vi "BIMS_Collector (2010_03).vi"() -> ()   [LabVIEW 2015]
doc: "This program is currently beta software. It is designed to address the data requirements defined primarily by the DHB Ballistic Test Report.\n\nThe general operation of this program is based on the Ballistics Version 2005 application developed internally by DuPont as a research tool for the Spruance Plant Ballistics Lab in Richmond, VA.\n\nPlease note that the original trigger control logic was modified and no longer depends on a safety interlock system to enable operation of a ballistic test.\n\nDuPont makes no warranties and assumes no liabilities in connection with any use of this program."
uses:
  <vilib>/addons/database/NI_Database_API.lvlib
  <vilib>/addons/database/Connection.llb/Conn Execute.vi
  <vilib>/addons/database/Recordset.llb/Rec Destroy - Connection.vi
  <vilib>/Utility/config.llb/NI_LVConfig.lvlib
  <vilib>/Utility/config.llb/Write Key (I32).vi
  Shot Record.ctl
  BIMS_Collector Globals.vi
  Collector State.ctl
  DataSource.ctl
  <vilib>/registry/registry.llb/Registry RtKey.ctl
  <vilib>/Utility/config.llb/Write Key (String).vi
  <vilib>/addons/database/Connection.llb/DB Tools Open Connec (Path).vi
panel:
  out "Loading":u16(ring)
  in  "runtimeMenusVisible":bool=TRUE
  in  "diagPageVisible":bool
  in  "RESET All":bool
  out "ConfigName":string
  out "TimeNow":string
  in  "EXIT":bool
  in  "mainTabCntrl":enum32{"Setup", "Measure", "History", "System"}(tab)=enum."System"
  in  "SampleEntryTabCntrl":enum32{"Environment", "Sample"}(tab)
  in  "ThreatDetails":u16(ring) caption="Detail"
  in  "ThreatGroups":u16(ring) caption="Group" items=["", "RCC", "FSP", "44 Magnum", "40 S&W", "9mm Luger", "357 Magnum", "357 Sig", "5.56 NATO / 223", "7.62 Win"]
  in  "PowderTypes":u16(ring) caption="Type" items=["", "ACCURATE, NO.2", "ACCURATE, NO.9", "Alliant Herc. Bullseye", "Alliant 2400", "Hercules", "Hi-Skor 700x", "Hi-Skor 800x", "IMR-4198", "IMR-4756", "IMR-4895", "Power Pistol", "Winchester Ball", "WINCHESTER-231", "WINCHESTER-296", "OTHER"]
  in  "Ballisticians":u16(ring) caption="Ballistician" items=["", "Luke Jeter", "Pat Fitzgerald", "James Singletary", "Aldo Tavarez"]
  in  "Recorders":u16(ring) caption="Recorder"
  in  "Shooters":u16(ring) caption="Shooter"
  in  "Methods":u16(ring) caption="Method" items=["", "V50", "NIJ", "V0", "Custom"]
  in  "RoomT":sgl caption="Temperature (° F)" format="%.1f"
  in  "RoomHum":sgl caption="Humidity (%)" min=0 max=100 format="%.1f"
  in  "SampleBackings":u16(ring)=3 caption="Type" items=["", "Clay", "Aluminum", "Air"]
  in  "clayCalArray":i16[](array[numeric])=[0, 0, 0, 0, 0] caption="Calibration (mm)" min=0 max=99 format="%02.0f"
  out "clayAverage":sgl caption="Clay Average (mm)" format="%#.1f"
  in  "clayTemp":sgl caption="Clay Temp (° F)" format="%.1f"
  out "threatDetails":T1 caption="Description"
  in  "SampleClamping":u16(ring) caption="Clamping" items=["", "None", "12 x 12", "12 x 15", "15 x 15 Flat", "15 x 15 Teeth", "16 x 16 Flat", "16 x 16 Teeth", "18 x 18", "20 x 20", "Hydro Pneumatic"]
  in  "Sample SubTabCntrl":T2(tab)
  in  "SampleID":string caption="Sample ID"
  in  "SampleDimensions":u16(ring) caption="Dimensions" items=["", "15 x 15", "12 x 12", "10.25 x 11.75", "15 x 16", "26 x 26", "8.5 x 11", "12 x 15", "16 x 16", "18 x 18", "20 x 16", "15 x 18", "24 x 24", "13 x 13", "7.5 x 7.5", "VEST PANEL", "CHEST PLATE", "HELMET", "NOT APPLICABLE"]
  in  "ModelMfrs":u16(ring) caption="Manufacturer" items=["DuPont Experimental", "Clark Schwebel", "Industriales Textiles", "Maydown", "Second Chance Body Armor", "Point Blank-Marine Interceptor", "Safari Land", "American Body Armor", "Europe", "Force One", "Textile Filter", "Hexcel Schwebel", "BGF", "M.C. GILL", "COLUMBIA", "Britax HEATH TECN", "ARLON", "TEX TECH INC.", "TELAIR", "CADDIN BODY ARMOR", "GEPCO", "3 TEX", "PACA BODY ARMOR", "VON ROL ISOLA", "SIOUX MANUFACTURING", "APEJ-TAIWAN", "FLOPPY BODY ARMOR", "UNICOR", "n/a", "Point Blank", "Diamond Back", "Other"]
  in  "SampleTypes":u16(ring) caption="Sample Type" items=["", "Fabric", "Hard", "Helmet", "Vest", "Paper"]
  in  "Submitters":u16(ring) caption="Submitter" items=["", "Aldo Tavarez", "James Singletary", "Jeff Hanks", "Karl Chang", "Minshon Chiou", "Other", "Navin Tejani", "Pat Fitzgerald", "Ron Egres", "Bryce VanArsdalen", "Kevin Mulcahy"]
  in  "ProjectID":string caption="Project ID"
  in  "BackLayers":i32 caption="# of Layers" min=0 max=99 step=5
  in  "FrontLayers":i32 caption="# of Layers" min=0 max=99 step=5
  in  "BackLayer":u16(ring) caption="Back Layer" items=["", "n/a", "CORDURA 500d"]
  in  "FrontLayer":u16(ring) caption="Front Layer" items=["", "n/a", "CORDURA 1000d"]
  out "totalNumLayers":i32 caption="Total # of Layers" min=0 max=100 step=5
  out "totalBAW":sgl caption="Total BAW (psf)" format="%.2f"
  in  "LayerTabControl":enum32{"1", "2", "3", "4", "5", "6"}(tab) caption="Inner Layers"
  out "fab1_totalWt":sgl caption="Fab1 Wt" min=0 max=99 step=5 format="%.2f"
  out "SampleAttribs_1":T3 caption="fabricAttribs_1"
  in  "Layer_1":T4={"plyNum"=0, "LotNum"="n/a", "RollNum"="n/a"} caption="Fabric #1" {"plyNum" min=0 max=99 step=5}
  in  "SampleStyle_1":u16(ring) items=["", "15492"]
  in  "Mfr_1":u16(ring) caption="vendor" items=["", "Barrday", "DSM", "DuPont AFS", "Dyneema", "Honeywell", "JPS", "TexTech"]
  in  "layerStitch_1":u16(ring) caption="Stitch" items=["", "1-inch quilt", "2-inch quilt", "Corner Bartack", "Corners", "Custom (Panel)", "Custom (Vest)", "Diamond", "Edge", "n/a", "Normal"]
  out "fab2_totalWt":sgl caption="Fab2 Wt" min=0 max=99 step=5 format="%.2f"
  out "SampleAttribs_2":T3 caption="fabricAttribs_2"
  in  "Layer_2":T4={"plyNum"=0, "LotNum"="n/a", "RollNum"="n/a"} caption="Fabric #2" {"plyNum" min=0 max=99 step=5}
  in  "SampleStyle_2":u16(ring)
  in  "Mfr_2":u16(ring) caption="vendor" items=["", "Barrday", "DSM", "DuPont AFS", "Dyneema", "Honeywell", "JPS", "TexTech"]
  in  "layerStitch_2":u16(ring) caption="Stitch" items=["", "1-inch quilt", "2-inch quilt", "Corner Bartack", "Corners", "Custom (Panel)", "Custom (Vest)", "Diamond", "Edge", "n/a", "Normal"]
  out "fab3_totalWt":sgl caption="Fab3 Wt" min=0 max=99 step=5 format="%.2f"
  out "SampleAttribs_3":T3 caption="fabricAttribs_3"
  in  "Layer_3":T4={"plyNum"=0, "LotNum"="n/a", "RollNum"="n/a"} caption="Fabric #3" {"plyNum" min=0 max=99 step=5}
  in  "SampleStyle_3":u16(ring)
  in  "Mfr_3":u16(ring) caption="vendor" items=["", "Barrday", "DSM", "DuPont AFS", "Dyneema", "Honeywell", "JPS", "TexTech"]
  in  "layerStitch_3":u16(ring) caption="Stitch" items=["", "1-inch quilt", "2-inch quilt", "Corner Bartack", "Corners", "Custom (Panel)", "Custom (Vest)", "Diamond", "Edge", "n/a", "Normal"]
  out "fab4_totalWt":sgl caption="Fab4 Wt" min=0 max=99 step=5 format="%.2f"
  out "SampleAttribs_4":T3 caption="fabricAttribs_4"
  in  "Layer_4":T4={"plyNum"=0, "LotNum"="n/a", "RollNum"="n/a"} caption="Fabric #4" {"plyNum" min=0 max=99 step=5}
  in  "SampleStyle_4":u16(ring)
  in  "Mfr_4":u16(ring) caption="vendor" items=["", "Barrday", "DSM", "DuPont AFS", "Dyneema", "Honeywell", "JPS", "TexTech"]
  in  "layerStitch_4":u16(ring) caption="Stitch" items=["", "1-inch quilt", "2-inch quilt", "Corner Bartack", "Corners", "Custom (Panel)", "Custom (Vest)", "Diamond", "Edge", "n/a", "Normal"]
  out "fab5_totalWt":sgl caption="Fab5 Wt" min=0 max=99 step=5 format="%.2f"
  out "SampleAttribs_5":T3 caption="fabricAttribs_5"
  in  "Layer_5":T4={"plyNum"=0, "LotNum"="n/a", "RollNum"="n/a"} caption="Fabric #5" {"plyNum" min=0 max=99 step=5}
  in  "SampleStyle_5":u16(ring)
  in  "Mfr_5":u16(ring) caption="vendor" items=["", "Barrday", "DSM", "DuPont AFS", "Dyneema", "Honeywell", "JPS", "TexTech"]
  in  "layerStitch_5":u16(ring) caption="Stitch" items=["", "1-inch quilt", "2-inch quilt", "Corner Bartack", "Corners", "Custom (Panel)", "Custom (Vest)", "Diamond", "Edge", "n/a", "Normal"]
  out "fab6_totalWt":sgl caption="Fab6 Wt" min=0 max=99 step=5 format="%.2f"
  out "SampleAttribs_6":T3 caption="fabricAttribs_6"
  in  "Layer_6":T4={"plyNum"=0, "LotNum"="n/a", "RollNum"="n/a"} caption="Fabric #6" {"plyNum" min=0 max=99 step=5}
  in  "SampleStyle_6":u16(ring)
  in  "Mfr_6":u16(ring) caption="vendor" items=["", "Barrday", "DSM", "DuPont AFS", "Dyneema", "Honeywell", "JPS", "TexTech"]
  in  "layerStitch_6":u16(ring) caption="Stitch" items=["", "1-inch quilt", "2-inch quilt", "Corner Bartack", "Corners", "Custom (Panel)", "Custom (Vest)", "Diamond", "Edge", "n/a", "Normal"]
  in  "SampleCoverings":u16(ring) caption="Sample Covering" items=["None", "RipStop", "Plastic bag", "Other"]
  in  "Assemblers":u16(ring) caption="Technician" items=["", "Not Known", "none", "Ron Egres", "Bryce VanArsdalen", "Mary Revels", "Matthew Street", "Patty Whitlow", "Tom Boyer"]
  in  "Thickness":dbl caption="Thickness (in)" format="%.3f"
  in  "totalSampleWt":sgl caption="Total Weight (lbs)" format="%.3f"
  in  "Comments":string caption="Remarks (optional):"
  in  "TestConditions":u16(ring) caption="Sample Condition" items=["", "Dry", "Wet", "Hot 160 DEG. F", "Cold", "Weapon Lubricant", "Motor Oil", "Conditioned", "Accelerated Aging"]
  in  "shotsTabCntrl":T5(tab)
  in  "Frag Rod":sgl format="%.1f"
  in  "MeasSrc":T6=enum."Screens" caption="Source"
  in  "Drag Corrected":bool=TRUE
  in  "ARM":bool
  in  "readyClock":bool caption="Clock"
  out "Impact/speed":sgl caption="Chronograph 1" min=0 max=10000 step=0.1 format="%.1f"
  out "SHOT STATUS":u16(ring) caption="Penetration" items=["Partial", "Complete"]
  out "residual/speed":sgl caption="Residual" min=0 max=10000 step=0.1 format="%.1f"
  out "SUBMIT DATE/TIME":string
  out "BACKFACE DEPTH":sgl caption="Backface\nDepth" min=0 max=200 step=5
  in  "MeasVelScrnSet1":sgl caption="Set #1" min=0 max=10000 step=0.1 format="%.1f"
  in  "Current/sthotstatus":u16(ring) caption="Penetration" items=["Partial", "Complete"]
  in  "Current/residual/speed":sgl caption="Residual Set" min=0 max=10000 step=0.1 format="%.1f"
  in  "currentDateTime":string caption="Date/Time"
  in  "MeasVelScrnSet2":sgl caption="Set #2" min=0 max=1000000 step=0.1 format="%.1f"
  out "%_Difference":sgl caption="% Vel Diff" format="%.3f"
  in  "backdepth":sgl caption="BF Depth"
  out "Redundant/speed":sgl caption="Chronograph 2" min=0 max=10000 step=0.1 format="%.1f"
  out "Current/avg/speed":sgl caption="Average" min=0 max=1000000 step=0.1 format="%.1f"
  out "Avg/speed":sgl caption="Average" min=0 max=10000 step=0.1 format="%.1f"
  out "SafetyInterlock":cluster{"ARMED":bool}
  out "DC_ factor":sgl=1.0 caption="DC Factor" format="%.4f"
  in  "Barrel Temp":sgl format="%.1f"
  in  "Shot Description":string caption="Description (optional)"
  in  "Powder Loading":sgl caption="Powder Load" min=0 max=100 step=0.1 format="%.3f"
  in  "Shot Angle":u16 max=90 step=1
  out "Projectile Mass":sgl caption="Projectile Mass (grains)" min=0 step=1
  in  "N.I.J":u16(ring) items=["n/a", "PASS", "FAIL"]
  out "Device S/N":string
  in  "addShot":bool caption="RANGE SETUP must be selected before shots can be added."
  in  "loadingUnits":enum32{"grams", "grains"}(radio)
  out "instruct_addShot":string="RANGE SETUP and THREAT must be selected before shots can be added."
  out "Set#1 Separation":sgl=4.0 caption="Outer" format="%.2f"
  out "Set#2 Separation":sgl=4.0 caption="Inner" format="%.2f"
  out "saveReq":string="Number of layers in sample ply specification and number of shots in shots table must be greater than 0 to enable saving."
  in  "VsVr Report":bool caption="Report"
  out "Table of Shots":string[][](table) caption="Shot Table"
  in  "MC Listbox of Shots":i32(listbox)
  in  "saveShots":bool
  in  "clearShots":bool
  out "highPartial":i32 caption="High Partial" min=0 max=10000 step=1
  out "lowComplete":i32 caption="Low Complete" min=0 max=10000 step=1
  out "rangeOfResults":i32 caption="Range of Results" min=0 max=10000 step=1
  out "zmr 2":sgl caption="ZMR" format="%.1f"
  out "computed_V50":sgl caption="V50" format="%.1f"
  out "Pairs":i16 min=0 max=100 step=1
  in  "reportV50":bool caption="Report"
  in  "maxDev":sgl=125.0 caption="Max Deviation" min=0 max=300 step=25
  in  "undoLastShot":bool
  in  "deleteShot":bool
  in  "nextShot":bool
  in  "SHOTS":T7[](array[typedef]) {"Frag Rod" format="%.1f"; "UncorrectedAvgVel_PB" format="%.1f"; "UncorrectedRed_PB" format="%.1f"; "strikeVel_PB" format="%.1f"; "velLoss_PB" format="%.1f"; "avgVel_PB" format="%.1f"; "Redundant_Velocity" format="%.1f"; "Energy Loss (J)" format="%.3e"; "Projectile Mass" min=0 step=1 format="%.4f"; "Corrected residual" format="%.2f"; "Uncorrected Residual" format="%.1f"; "Corrected Impact" format="%.2f"; "Uncorrected Impact" format="%.1f"; "Shot Angle" max=90 step=1; "SHOT STATUS" items=["Partial", "Complete"]; "IMPACT VELOCITY" min=0 max=10000 step=0.1 format="%.1f"; "Barrel Temperature" format="%.1f"; "Powder Loading" format="%.4f"; "RESIDUAL  VELOCITY" min=0 max=10000 step=0.1 format="%.1f"}
  out "velProfile":cluster{dbl, dbl}[](graph) caption="Shot Velocity Measurement Profile"
  out "velCompProf":cluster{"vStrike":dbl, "vA":dbl} caption="Velocity in fps\n(computed)"
  out "velMeasProf":T8 caption="Velocity in fps\n(measured)"
  out "relativeTime":cluster{"ts2":dbl, "ts3":dbl, "ts1":dbl} caption="Relative time\n(microsec)"
  out "displacement":T9={"ds_v2"=6.75, "ds2"=5.0833, "ds_vB"=4.9167, "ds3"=4.75, "ds_vAvg"=6.9167, "ds_v1"=7.0833, "ds1"=8.75, "ds_vA"=8.9167, "ds0"=9.0833} caption="Distance from\ntarget (ft)" {"ds0" format="%_4g"; "ds_vA" format="%_4g"; "ds1" format="%_4g"; "ds_v1" format="%_4g"; "ds_vAvg" format="%_4g"; "ds3" format="%_4g"; "ds_vB" format="%#_4g"; "ds2" format="%#_4g"; "ds_v2" format="%_4g"}
  out "arrIDC":dbl[](array[numeric]) caption="Instantaneous Drag Coefficient"
  in  "rangeSetup":u16(ring)=1 caption="Range Dimensions" items=["Short (small frag)", "Standard (handgun)", "Long (rifle)"]
  out "mid_to_targ_dist":sgl=5.0 caption="Mid To Target (ft)"
  in  "historyTabCntrl":enum32{"Powder Loading", "Panel Search"}(tab)=enum."Panel Search"
  in  "Threat.freeTxt":string caption="Threat"
  in  "Powder.freeTxt":string caption="Powder"
  in  "QueryLoad":bool
  in  "lkupEndDate":timestamp caption="End Date" format="%<%x>T"
  in  "lkupStartDate":timestamp caption="Begin Date" format="%<%x>T"
  out "Vel.vs.Loading":cluster{dbl[], dbl[]}(graph)
  out "v50_table":string[][](table)
  in  "maxRecs":u16=1001 caption="Max # of SHOT Records" min=1 max=10000 step=100
  out "ActualNumRecs":i32=1001 caption="Actual # Returned"
  in  "ThreatSize_0":u16(ring) caption="Threat Size" items=["", "2", "4", "16", "17", "44", "55", "62", "64", "85", "123", "124", "125", "148", "158", "166", "180", "207", "240"]
  in  "panelSearch":bool
  in  "Mfr_0":u16(ring) caption="Manufacturer" items=["", "Barrday", "DSM", "DuPont AFS", "Dyneema", "Honeywell", "JPS", "TexTech"]
  in  "SampleStyle_0":u16(ring) caption="Sample Style"
  in  "srchParams":T10={"maxPanels"=1001, "lkupPanelStartDate"=timestamp(0 s since 1904-01-01), "lkupPanelEndDate"=timestamp(3345122114.0909824 s since 1904-01-01)} {"lkupPanelEndDate" format="%<%x>T"; "lkupPanelStartDate" format="%<%x>T"; "maxPanels" min=1 max=10000 step=100}
  out "actualNumPanels":i32 caption="Actual # Returned"
  out "pastPanels":string[][](table)
  in  "Record #":i32=1 min=0 max=16
  in  "reportV50_History":bool
  out "SampleAttribs_0":T11 caption="fabricAttribs_1"
  in  "Requestors_0":u16(ring) caption="Requestor" items=["", "Aldo Tavarez", "Bryce VanArsdalen", "James Singletary", "Jeff Hanks", "Karl Chang", "Kevin Mulcahy", "Minshon Chiou", "Navin Tejani", "Other", "Pat Fitzgerald", "Ron Egres"]
  in  "aboutTabCntrl":T12(tab)
  in  "RefreshMetadata":bool
  out "LastShot":i32 caption="Shot"
  out "LastSample":i32 caption="Sample"
  in  "PublishNewRecords":bool
  in  "clearErrors":bool
  in  "useBMC":bool caption="Use Message Center?"
  in  "Server":string="esvrs11"
  in  "Site":string="ICE1"
  in  "TestStandards":u16(ring)=2 caption="Standard" items=["n/a", "NIJ 0101.04", "MIL-STD-662F"]
  in  "WeaponTypes":u16(ring) caption="Weapon" items=["", "Universal Receiver", "Other"]
  in  "processShots":bool
  out "DIO":u32=21 format="%.0b"
  in  "line direction map":i32=1792 format="%.0b"
  out "Corrected Average":sgl=1527.9313 format="%.2f"
  out "CorrectedVelScrnSet2":sgl=1551.8816 caption="Corrected Redundant" format="%.2f"
  out "conversion factor":sgl=0.3048037 format="%.5f"
  out "#_completes":i32
  out "#_partials":i32
  in  "percent warning":sgl=1.0 format="%.2f"
  in  "SoftwareVersion":dbl caption="Version" format="%.2f"
  out "impact/ID":u32=83886081 format="%.0x"
  out "residual/ID":u32=83951617 format="%.0x"
  out "Red/ID":u32=84017153 format="%.0x"
  out "correction coefficient":sgl format="%.8f"
  out "Corrected Residual":sgl=751.9905 format="%.2f"
  out "CorrectedVelScrnSet1":sgl=1503.981 format="%.2f"
  out "Barrel to Screen":sgl=7.8333 format="%.2f"
  in  "Set#1_to_Target":sgl=7.083333 format="%.2f"
  out "Residual/Separation":sgl=4.0 format="%.2f"
  in  "Residual/Target Dist":sgl=7.083333 format="%.2f"
  out "Z.M.R.":sgl min=0 step=0.1 format="%.1f"
  in  "old threat":u16
  out "Complete":sgl[](array[numeric]) format="%.2f"
  out "factor array":sgl[](array[numeric]) format="%.4f"
  out "Partial":sgl[](array[numeric]) format="%.2f"
  in  "DAQ Card":i16=1
  in  "Impact Timer":i16 min=0 max=3 step=1
  in  "Redundant Timer":i16=1 min=0 max=3 step=1
  in  "Residual  Timer":i16=2 min=0 max=3 step=1
  out "Impact factor":sgl=1.0 caption="Impact" min=0 max=1 format="%.5f"
  out "Residual factor":sgl=1.0 caption="Residual" min=0 max=1 format="%.5f"
  in  "Areal Density":dbl format="%.2f"
  in  "Areal density text":string
  in  "Fabric Description":string caption="Fabric Desc"
  in  "clayCalib":string="##-##-##-##-##" caption="Calibration"
  in  "lookupRec":bool caption="lookup"
  out "STOP (Shots MC LB)":bool=TRUE
  out "configPath":path=path "P:/Private/My Projects/AFS/BIMS/2008/BIMS_Collector.ini" caption="Configuration Path (INI)"
  in  "minV50":i32=1500 caption="Minimum V50"
  in  "Type of work":string="QC"
  in  "Threat":u16(ring) caption="Threat (long description)"
  out "massUnits":string="GRAMS" caption="Weight Units"
  out "lengthUnits":string="FOOT" caption="Distance Units"
  in  "SampleDescrip":u16(ring) caption="Misc. Sample Description (legacy)"
  in  "serialNum":string caption="Serial #"
  in  "Models":u16(ring) caption="Model #" items=["n/a"]
  in  "InterlockExists":bool=TRUE caption="Safety Interlock Hardware Exist?"
  in  "ScreenSetAvgg":bool caption="Average Screen Sets?"
  in  "Sort by AVG":bool=TRUE caption="Sort shots by average velocity"
  in  "useBallisitican":bool=TRUE caption="Use Ballistician field in Setup?"
  in  "useRecorder":bool caption="Use Recorder field in Setup?"
  in  "useShooter":bool caption="Use Shooter field in Setup?"
  out "SMErr":errorcluster
  out "U/I EvErr":errorcluster
  out "booleanDump":bool
  out "GrainSize":u16 caption="Grain"
  in  "LayerStitchTypes":u16(ring) caption="Stitch" items=["", "Custom (Vest)", "Corners", "1-inch quilt", "2-inch quilt", "Normal", "Custom (Panel)", "Corner Bartack", "Diamond", "Edge", "n/a"]
  # "Effectively restarts the application from scratch, as if the user pressed the EXIT button and then restarted the application."
  # "Configured for"
  # "Threat"
  # "*"
  # "*"
  # "Test"
  # "Powder"
  # "*"
  # "Personnel"
  # "Room"
  # "*"
  # "Backing"
  # "*"
  # "*"
  # "*"
  # "Body Side"
  # "Strike Face"
  # "Layer"
  # "Mfr"
  # "Style"
  # "# of Plies"
  # "Lot"
  # "Roll"
  # "Stitch"
  # "Internal ID"
  # "Fiber"
  # "Denier"
  # "Construction"
  # "Weave"
  # "Finish"
  # "Basis weight (oz/yd²)"
  # "Yarn Merge"
  # "Total Weight"
  # "*"
  # "*"
  # "*"
  # "1"
  # "2"
  # "3"
  # "4"
  # "5"
  # "6"
  # "Required"
  # "*"
  # "Timing System"
  # "Shot Parameters"
  # "cm"
  # "deg"
  # "degF"
  # "Velocity Measurements"
  # "Observations"
  # "Screens\nSeparation"
  # "Ft"
  # "Table Functions"
  # "Summary"
  # "Reports"
  # "Test Record"
  # "Edit Shot Records"
  # "Corrected"
  # "Shot #"
  # "t0"
  # "0"
  # "S Strike"
  # "0"
  # "Internal ID#"
  # "Fiber"
  # "Denier"
  # "Pick"
  # "Weave"
  # "Finish"
  # "oz/yd²"
  # "Asset"
  # "DuPont Ballistics Information Management System\n\nBIMS\nEnterprise Edition\n\n\nSample Performance\nData Collector\n\nMarch 2010"
  # "DuET Measurement System Technologies\nDUCOM 8 695-2330 for technical support\n\nCopyright © 2009 DuPont Company"
  # "Last Assigned\nRecord Numbers"
  # "Deployment Configuration"
  # "Data items support Point Blank requirements:"
  # "Correction Factors"
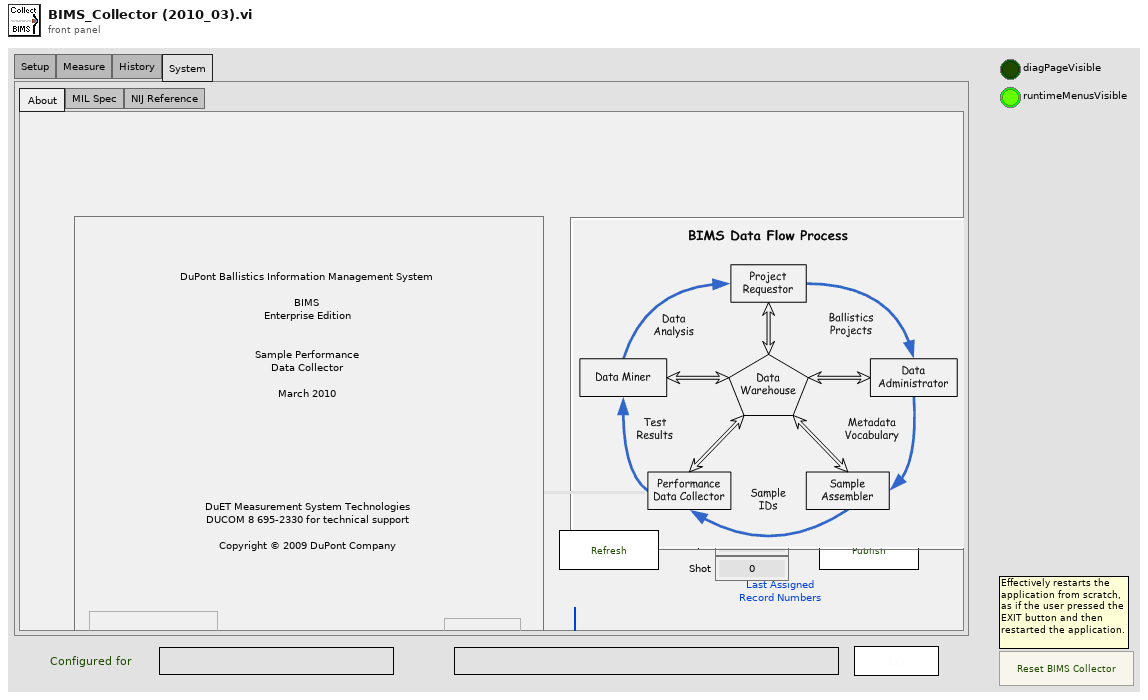
[diagram p1: front panel]
types:
  T1 = cluster{"barrelLength":string, "dragCorrection":string, "detailDescription":string, "barrelCaliber":string, "grainSize":string, "Make":string, "Model":string}
  T2 = enum32{"General Specification", "Ply Specification", "Preparation"}
  T3 = cluster{"Fabric.fiber":string, "Fabric.denier":string, "pick":string, "weave":string, "finish":string, "ozPerYd2":string, "fabricID_DHB":string, "yarnMerge":string}
  T4 = cluster{"plyNum":i32, "LotNum":string, "RollNum":string}
  T5 = enum32{"Ready-Aim-Fire", "Shots Table", "Edit", "Instantaneous DC"}
  T6 = typedef "DataSource.ctl" = enum16{"Simulated", "Radar", "Screens"}
  T7 = typedef "Shot Record.ctl" = cluster{"Uncorrected Impact":sgl, "Uncorrected Residual":sgl, "avgVel_PB":sgl, "IMPACT VELOCITY":sgl, "RESIDUAL  VELOCITY ":sgl, "Shot Description":string, "Powder Loading ":sgl, "Barrel Temperature":sgl, "TIME / DATE":string, "shot order":i32, "SHOT STATUS":u16, "Shot Angle":u16, "Corrected Impact":sgl, "Corrected residual":sgl, "Projectile Mass":sgl, "usedv50":bool, "Energy Loss (J)":sgl, "BackFace\nDepth":sgl, "BackFace\nDiameter":sgl, "Redundant_Velocity":sgl, "velLoss_PB":sgl, "strikeVel_PB":sgl, "UncorrectedRed_PB":sgl, "CorrectedRed_PB":sgl, "UncorrectedAvgVel_PB":sgl, "V50userExcl":bool, "Frag Rod":sgl}
  T8 = cluster{"v2":dbl, "vB":dbl, "vOuter":dbl, "v1":dbl, "vA":dbl, "vInner":dbl}
  T9 = cluster{"ds_v2":dbl, "ds2":dbl, "ds_vB":dbl, "ds3":dbl, "ds_vAvg":dbl, "ds_v1":dbl, "ds1":dbl, "ds_vA":dbl, "ds0":dbl}
  T10 = cluster{"maxPanels":u16, "lkupPanelStartDate":timestamp, "lkupPanelEndDate":timestamp}
  T11 = cluster{"Fabric.fiber":string, "Fabric.denier":string, "pick":string, "weave":string, "finish":string, "ozPerYd2":string, "fabricID_DHB":string, "asset":string}
  T12 = enum32{"About ", "MIL Spec", "NIJ Reference", "Internal Use"}
  T13 = typedef "Collector State.ctl" = enum16{"POLL", "INITIALIZE", "V50 Report or GET Record", "VsVr Report", "SAVE SHOTS", "ADD SHOT", "CLEAR SHOTS", "NEXT SHOT", "DELETE SHOT", "READY CLOCK", "PROC SHOTS", "CHECK DAQ"}
  T14 = enum8{"Enabled", "Disabled", "Disabled and Grayed Out"}
  T15 = enum32{"Page Enabled", "Page Disabled", "Page Disabled & Grayed"}
  T16 = typedef "Registry RtKey.ctl" = enum32{"HKEY_CLASSES_ROOT", "HKEY_CURRENT_USER", "HKEY_LOCAL_MACHINE", "HKEY_USERS", "HKEY_PERFORMANCE_DATA", "HKEY_CURRENT_CONFIG", "HKEY_DYN_DATA"}
  T17 = cluster{"[0]":string, "[1]":string, "[2]":string, "[3]":string, "[4]":string, "[5]":string, "[6]":string, "[7]":string, "[8]":string, "[9]":string}[]
  T18 = cluster{"[0]":string, "[1]":string, "[2]":string, "[3]":string, "[4]":string, "[5]":string, "[6]":string, "[7]":string, "[8]":string}[]
  T19 = typedef "Collector State.ctl" = enum16{"POLL", "INITIALIZE", "V50 Report or GET Record", "VsVr Report", "SAVE SHOTS", "ADD SHOT", "CLEAR SHOTS", "NEXT SHOT", "DELETE SHOT", "PROCESS SHOTS", "READY CLOCK", "CHECK DAQ"}
  T20 = cluster{"Fabric.fiber":string, "Fabric.denier":string, "pick":string, "weave":string, "finish":string, "ozPerYd2":string, "fabricID_DHB":string, "yarnMerge":string}[]
  T21 = cluster{"SampleTypes":refnum<vi>, "SampleDescrip":refnum<vi>}
  T22 = cluster{"max dev":sgl, "residual separation":sgl, "Set#1 Separation":sgl, "Set#2 Separation ":sgl, "impact target dist":sgl, "resid target dist":sgl, "barrel screen dist":sgl, "midpt_to_target_dist":sgl}
  T23 = cluster{"fiber":string, "denier":string, "pick":string, "weave":string, "finish":string, "ozPerYd2":string, "internal_ID":string, "asset":string}[]
  T24 = cluster{"numOfPlies":i32, "LotNum":string, "RollNum":string}[]
  T25 = cluster{string, string, string, string, string, string, string, string, "clayCalib":string, string}
  T26 = cluster{string, string, string, string, string, string, string}
  T27 = cluster{"SampleID":string, "element":string, "Type of work":string, "serialNum":string, "element":string, string, string, string, "element":string, string}
  T28 = cluster{"SampleID":string, "element":string, string, string, string, "element":string}
  T29 = cluster{"[0]":string, "[1]":string, "[2]":string, "[3]":string, "[4]":string, "[5]":string, "[6]":string, "[7]":string, "[8]":string, "[9]":string}
  T30 = cluster{"[0]":string, "[1]":string, "[2]":string, "[3]":string, "[4]":string, "[5]":string, "[6]":string, "[7]":string, "[8]":string}
  T31 = cluster{"element":string, "element":string, "grainSize":string, "element":string, "barrelLength":string, string, "element":string, "element":string, "element":string}
  T32 = cluster{"element":string, "grainSize":string, "element":string, "barrelLength":string, string, "element":string}
  T33 = typedef "NI_Database_API.lvlib/Conn ObjectReference.ctl" = refnum<k1>
  T34 = typedef "NI_Database_API.lvlib/Rec ObjectReference.ctl" = refnum<k1>
  T35 = typedef "NI_LVConfig.lvlib/Config Data RefNum.ctl" = refnum<k1>
  T36 = cluster{"task ID out":u32, "task ID out":u32, "task ID out":u32}
  T37 = enum32{"invalid app kind", "Development System", "Run Time System", "Student Edition", "Embedded LabVIEW", "Evaluation", "Custom"}
  T38 = typedef "LVRowAndColumnTypeDef.ctl" = cluster{"Row":i32, "Column":i32}
  T39 = cluster{"barrelLength":string, "dragCoefficient":string, "detailDescription":string, "barrelCaliber":string, "grainSize":string, "Make":string, "Model":string}
  T40 = cluster{"fiber":string, "denier":string, "construction":string, "weave":string, "finish":string, "ozPerYd2":string, "fabricStyle_DHB":string, "yarnMerge":string}
  T41 = cluster{"plyNum":i32, "LotNum":string, "RollNum":string}[]
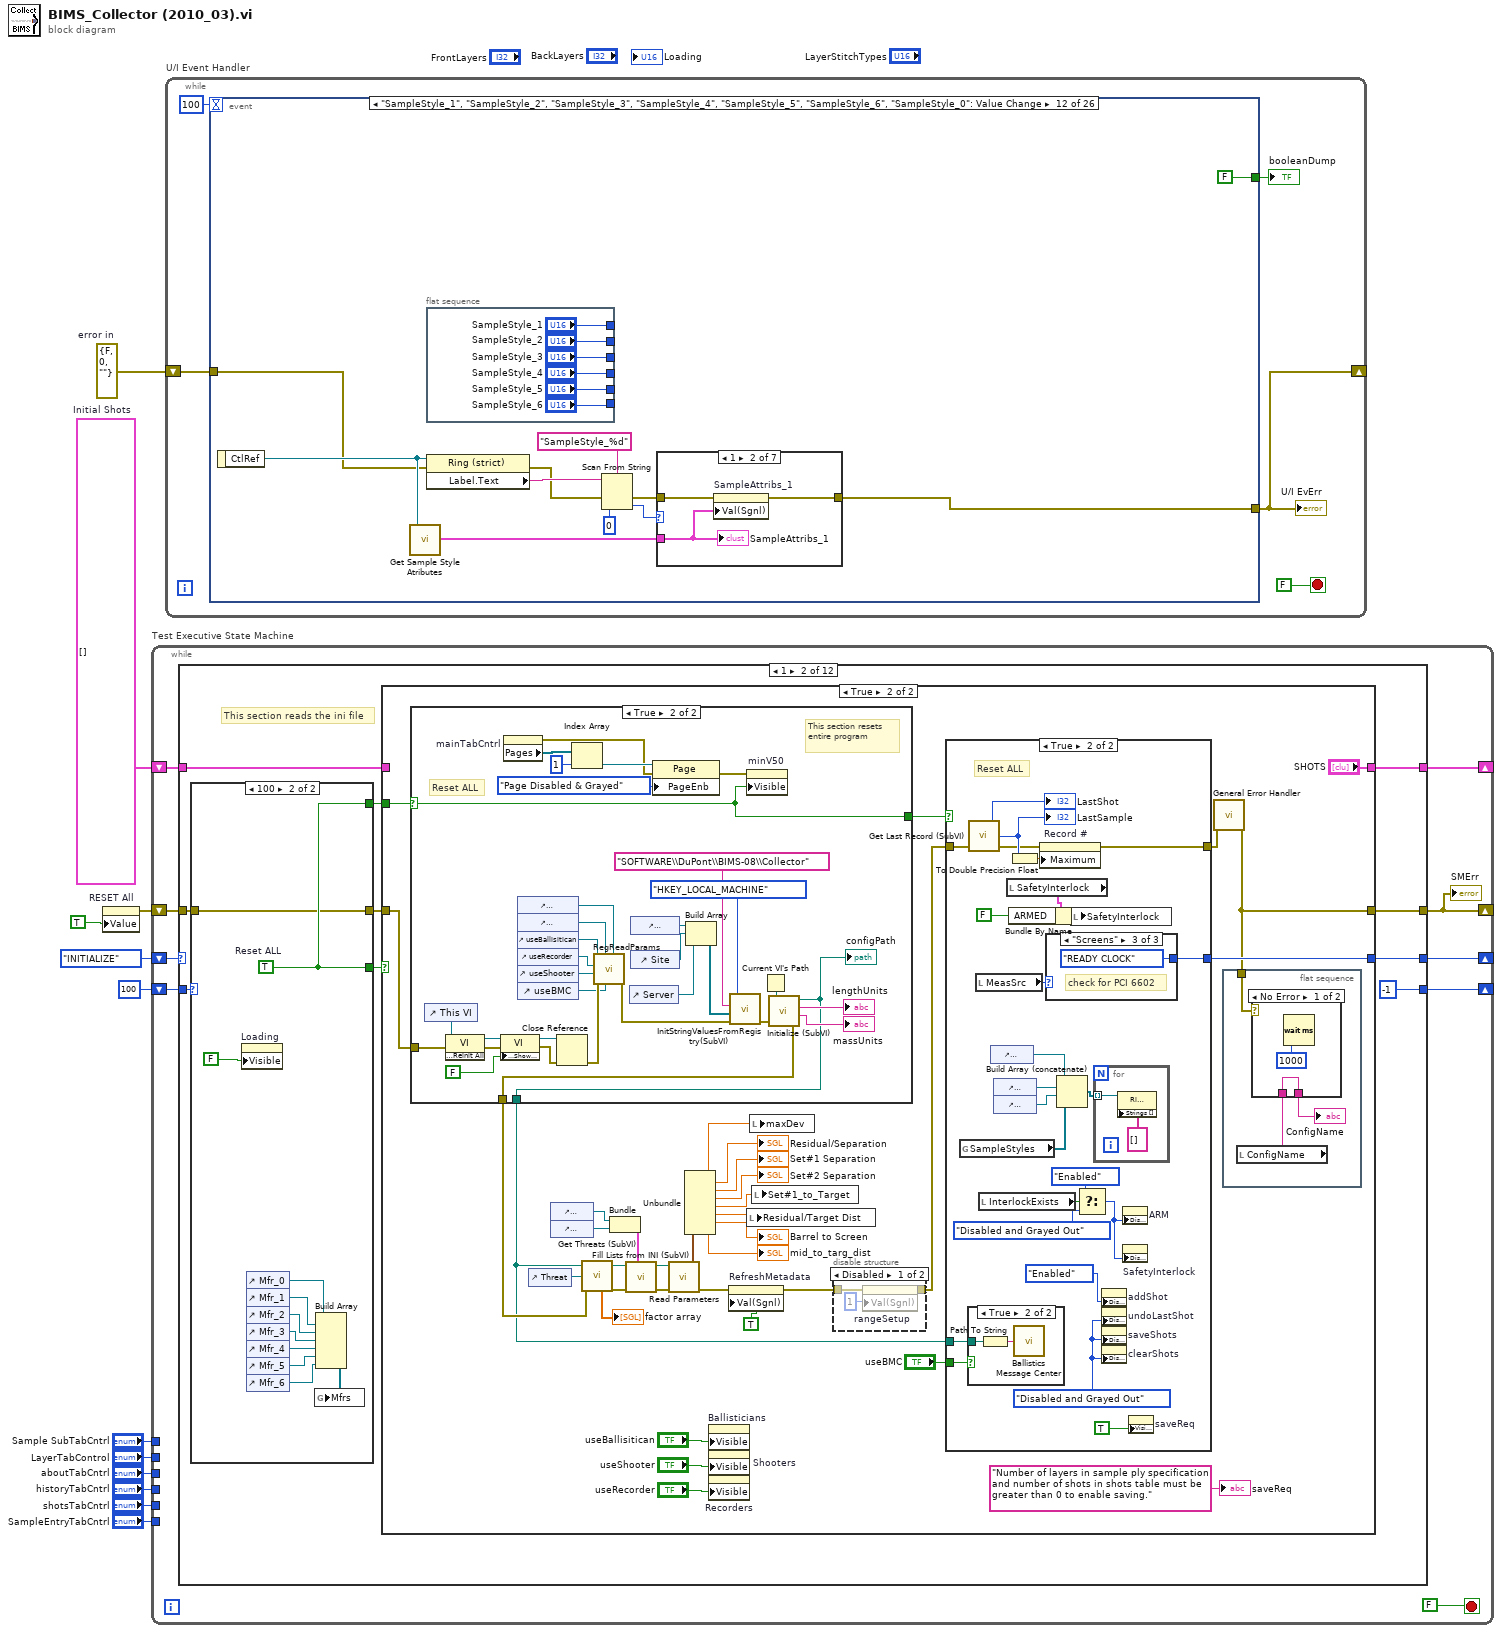
[diagram p0: block diagram]
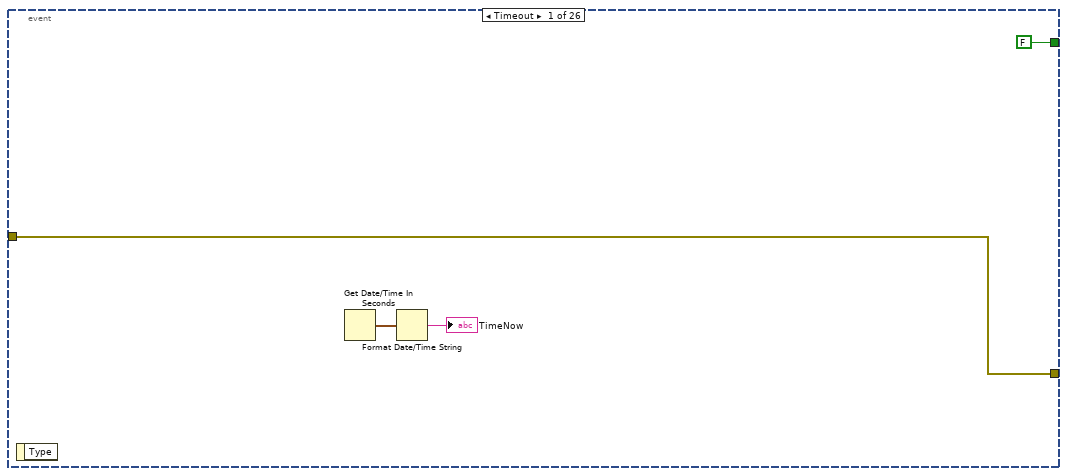
[diagram p2: hidden frame]
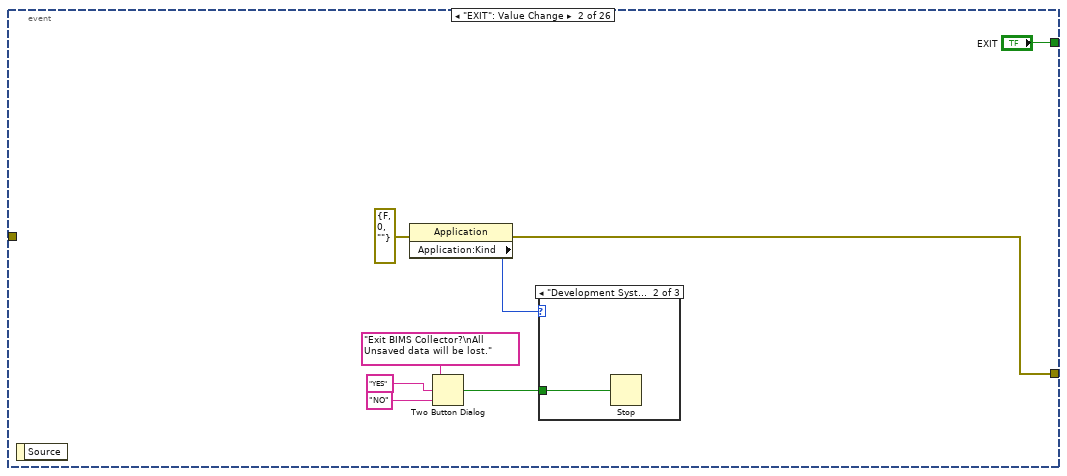
[diagram p3: hidden frame]
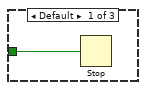
[diagram p4: hidden frame]
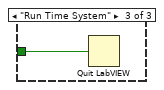
[diagram p5: hidden frame]
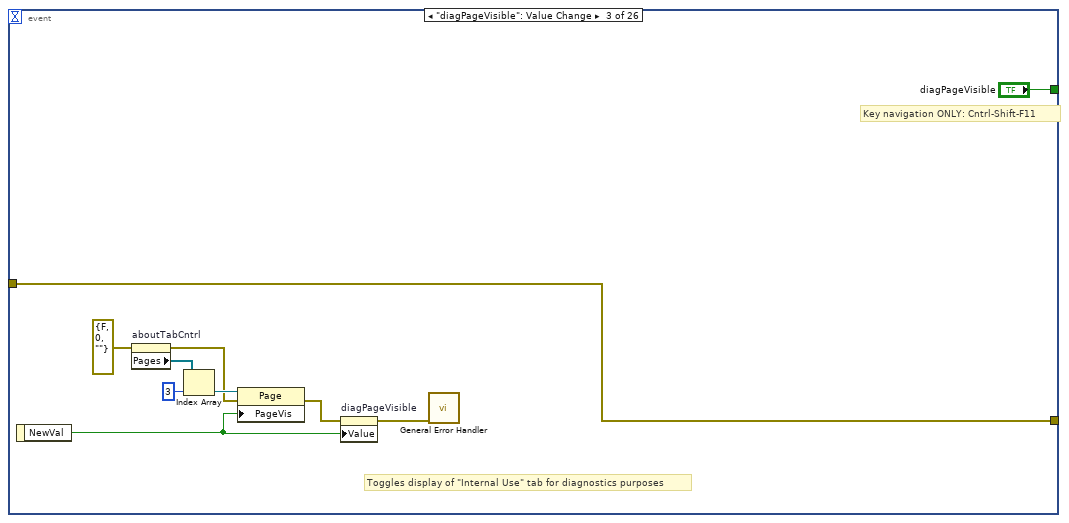
[diagram p6: hidden frame]
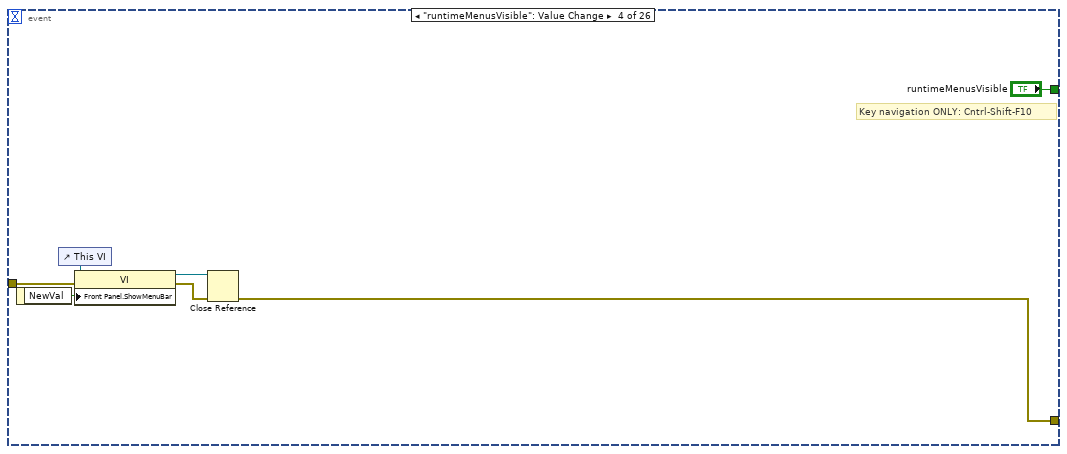
[diagram p7: hidden frame]
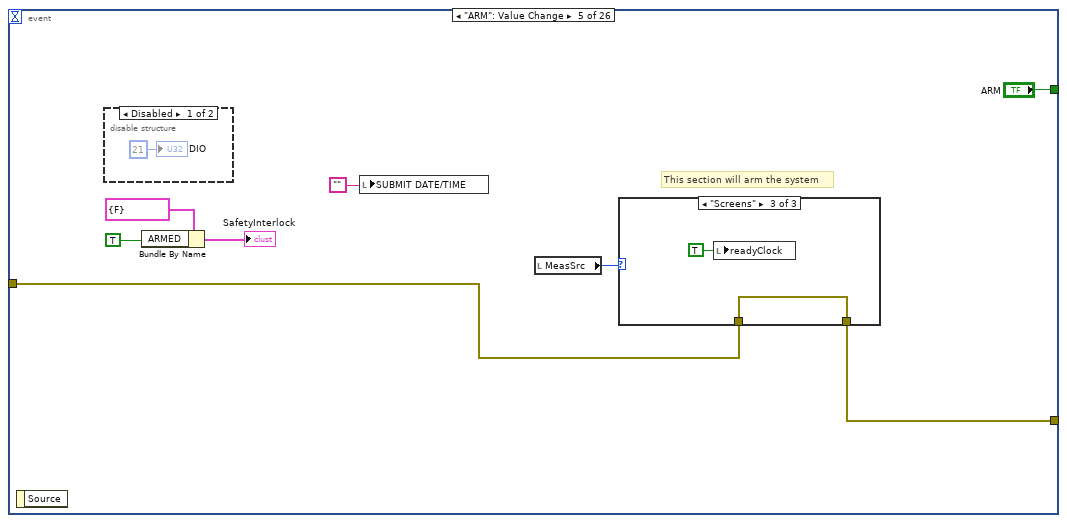
[diagram p8: hidden frame]
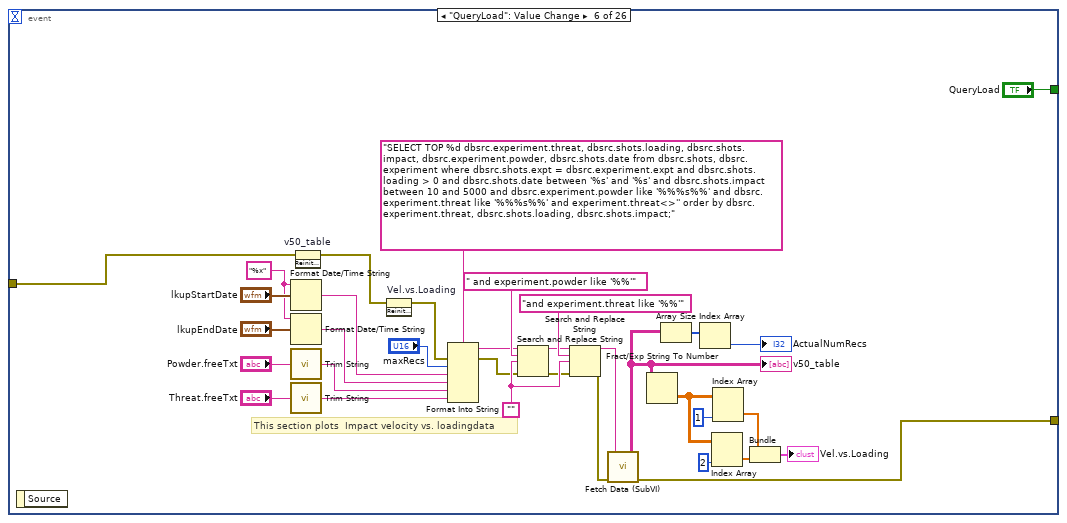
[diagram p12: hidden frame]
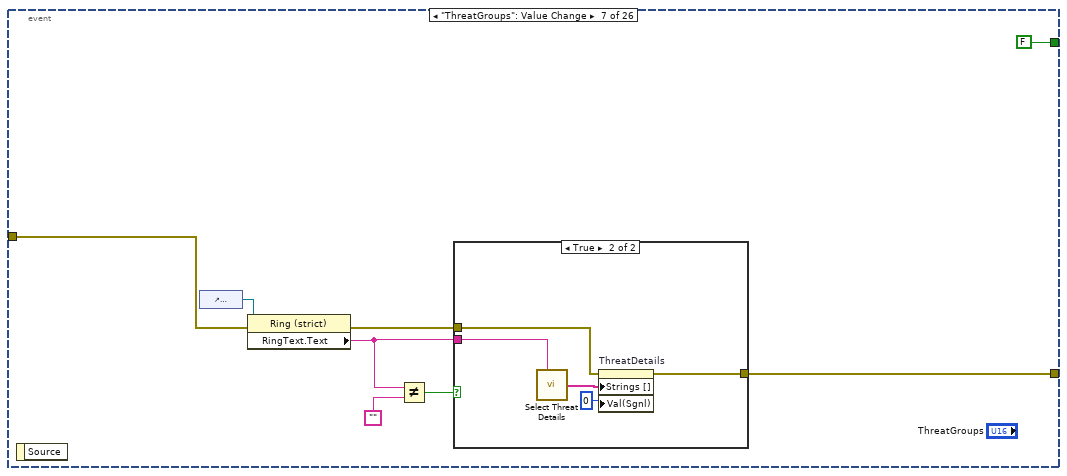
[diagram p13: hidden frame]
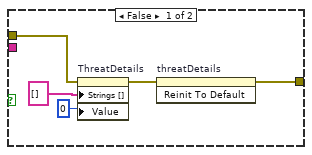
[diagram p14: hidden frame]
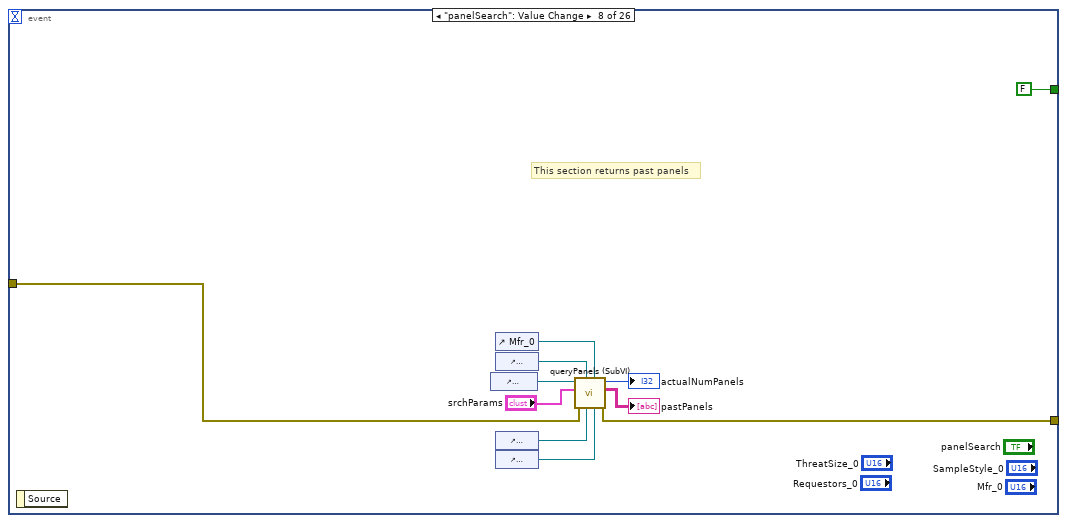
[diagram p15: hidden frame]
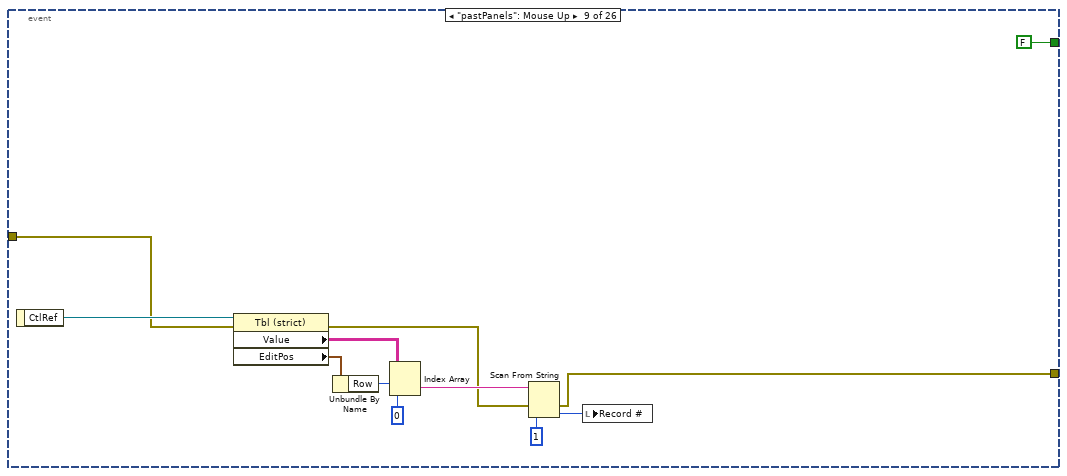
[diagram p16: hidden frame]
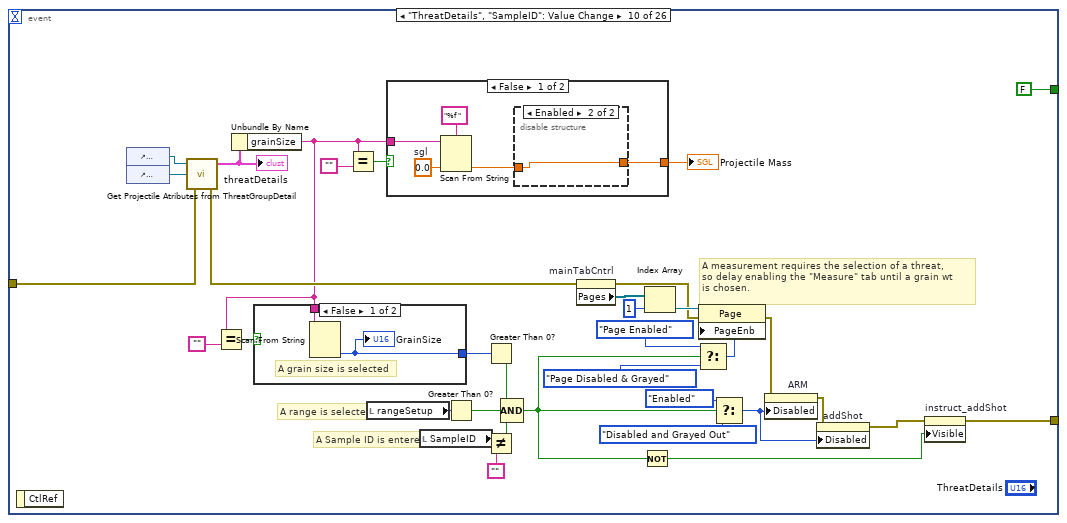
[diagram p17: hidden frame]
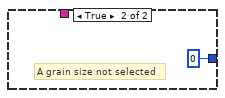
[diagram p18: hidden frame]
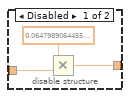
[diagram p19: hidden frame]
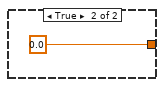
[diagram p20: hidden frame]
diagram:
  w7 = errorcluster {"status"=FALSE, "code"=0, "source"=""}  # error in
  w8 = T7[] []  # Initial Shots
  n1 = property on="RESET All" class="Bool (strict)"("Value"=TRUE ("RESET")) -> (error out=w10:errorcluster)  [unwired: 2 in, 1 out]
  n2 = while "Test Executive State Machine" {
    shift-left: 100 -> [w18]
    shift-right: [w19] -> _
    shift-left: Collector_State."INITIALIZE" ("progState") -> [w15]
    shift-right: [w20] -> _
    shift-right: [w16] -> _
    shift-left: w8 -> [w17]
    shift-right: [w13] -> _
    shift-left: w10 -> [w14]
    tunnel: "LayerTabControl" -> [_]
    tunnel: "aboutTabCntrl" -> [_]
    tunnel: "historyTabCntrl" -> [_]
    tunnel: "shotsTabCntrl" -> [_]
    tunnel: "SampleEntryTabCntrl" -> [_]
    tunnel: "Sample SubTabCntrl" -> [_]
    stop <- FALSE stop-if-true
    n3 = case shown="1" w15 {
      tunnel: [w38 w136 Collector_State."POLL" ("progState") Collector_State."POLL" ("progState") w1071 Collector_State."PROCESS SHOTS" ("progState") Collector_State."POLL" ("progState") Collector_State."PROCESS SHOTS" ("progState") Collector_State."PROCESS SHOTS" ("progState") Collector_State."POLL" ("progState") Collector_State."POLL" ("progState") w1734] -> w20
      tunnel: [-1 -1 ("index of element") -1 ("index of element") -1 ("index of element") w1070 -1 ("index of element") -1 -1 ("index of element") -1 ("index of element") -1 -1 ("index of element") w1733] -> w19
      tunnel: w18 -> [_ w137 _ _ _ _ _ _ _ _ _ _]
      tunnel: w17 -> [w34 w135 w291 w818 w1064 w1327 w1372 w1395 w1401 w1454 w1506 w1737]
      tunnel: [w34 w134 w291 w818 w1063 w1322 w1376 w1394 w1400 w1454 w1510 w1737] -> w16
      tunnel: w14 -> [_ w130 w288 w816 w1066 w1321 w1368 w1384 w1396 w1450 w1505 w1728]
      tunnel: [w28 w131 w287 w815 w1065 w1319 w1368 w1382 w1397 w1449 w1504 w1729] -> w13
      frame 0, Default {
        w54 = Collector_State."POLL"  # progStateType
        w44 = TRUE  # element
        w47 = 4  # SAVE
        # "This section checks for any buttons, maintains routine check of the paramters"
        n4 = case shown="\"Setup\", Default" "mainTabCntrl" {
          tunnel: w34 -> [_ w97 _ _]
          frame "Setup", Default {
            n5 = control-ref of="layerStitch_1"() -> (w65:refnum<vi>)
            n6 = control-ref of="layerStitch_2"() -> (w64:refnum<vi>)
            n7 = control-ref of="layerStitch_3"() -> (w63:refnum<vi>)
            n8 = control-ref of="layerStitch_4"() -> (w62:refnum<vi>)
            n9 = control-ref of="layerStitch_5"() -> (w61:refnum<vi>)
            n10 = control-ref of="layerStitch_6"() -> (w60:refnum<vi>)
            n11 = control-ref of="SampleStyle_0"() -> (w58:refnum<vi>)
            n12 = control-ref of="SampleStyle_1"() -> (w79:refnum<vi>)
            n13 = control-ref of="SampleStyle_2"() -> (w80:refnum<vi>)
            n14 = control-ref of="SampleStyle_3"() -> (w81:refnum<vi>)
            n15 = control-ref of="SampleStyle_4"() -> (w82:refnum<vi>)
            n16 = control-ref of="SampleStyle_5"() -> (w83:refnum<vi>)
            n17 = control-ref of="SampleStyle_6"() -> (w84:refnum<vi>)
            n18 = Build Array(w58, w79, w80, w81, w82, w83, w84) -> (w77:refnum<vi>[])
            n19 = global write "BIMS_Collector Globals.vi" "SampleStyles"(w77) -> ()
            n20 = Build Array(w65, w64, w63, w62, w61, w60) -> (w66:refnum<vi>[])
            n21 = global write "BIMS_Collector Globals.vi" "LayerStitchTypeRefs"(w66) -> ()
            n22 = local read "SampleAttribs_1"() -> (w71:T3)
            n23 = local read "SampleAttribs_2"() -> (w73:T3)
            n24 = local read "SampleAttribs_3"() -> (w74:T3)
            n25 = local read "SampleAttribs_4"() -> (w75:T3)
            n26 = local read "SampleAttribs_5"() -> (w76:T3)
            n27 = local read "SampleAttribs_6"() -> (w72:T3)
            n28 = Build Array(w71, w73, w74, w75, w76, w72) -> (w70:T20)
            n29 = global write "BIMS_Collector Globals.vi" "SampleAttribs"(w70) -> ()
            n30 = local read "Fabric Description"() -> (w69:string)
            n31 = control-ref of="Mfr_0"() -> (w59:refnum<vi>)
            n32 = control-ref of="Mfr_1"() -> (w90:refnum<vi>)
            n33 = control-ref of="Mfr_2"() -> (w89:refnum<vi>)
            n34 = control-ref of="Mfr_3"() -> (w88:refnum<vi>)
            n35 = control-ref of="Mfr_4"() -> (w87:refnum<vi>)
            n36 = control-ref of="Mfr_5"() -> (w86:refnum<vi>)
            n37 = control-ref of="Mfr_6"() -> (w85:refnum<vi>)
            n38 = String Subset(string=w69, length (rest)=75 ("length (rest)")) -> (substring=w68:string)  [unwired: 1 out]
            n39 = Build Array(w59, w90, w89, w88, w87, w86, w85) -> (w78:refnum<vi>[])
            n40 = local write "Fabric Description"(w68) -> ()
            n41 = global write "BIMS_Collector Globals.vi" "Mfrs"(w78) -> ()
          }
          frame "Measure" {
            # "Disable and gray out the \"Save\" button\nIF the shot table has no shots, \nOR if there are no plies; otherwise, enable it."
            # "Disable and gray out the \"Clear Shots\" button\nIF the shot table has no shots; otherwise, enable it."
            n42 = local read "totalNumLayers"() -> (w106:i32)
            n43 = Array Size(array=w97) -> (size(s)=w107:i32)
            n44 = Equal To 0?(x=w106) -> (x = 0?=w105:bool)
            n45 = Equal To 0?(x=w107) -> (x = 0?=w103:bool)
            n46 = Or(x=w103, y=w105) -> (x .or. y?=w96:bool)
            n47 = property on="saveReq" class="Str"("Visible"=w96) -> ()  [unwired: 2 in, 2 out]
            n48 = Select(t=T14."Disabled and Grayed Out" ("Disabled"), s=w103, f=T14."Enabled" ("Disabled")) -> (s? t:f=w104:T14)
            n49 = Select(t=T14."Disabled and Grayed Out" ("Disabled"), s=w96, f=T14."Enabled" ("Disabled")) -> (s? t:f=w91:T14)
            n50 = property on="reportV50" class="Bool"("Disabled"=w91) -> ()  [unwired: 2 in, 2 out]
            n51 = property on="saveShots" class="Bool"("Disabled"=w91) -> ()  [unwired: 2 in, 2 out]
            n52 = property on="clearShots" class="Bool"("Disabled"=w104) -> ()  [unwired: 2 in, 2 out]
            n53 = local read "Shot Description"() -> (w100:string)
            n54 = String Subset(string=w100, length (rest)=30 ("length (rest)")) -> (substring=w98:string)  [unwired: 1 out]
            n55 = local write "Shot Description"(w98) -> ()
            "SHOT STATUS" <- "Current/sthotstatus"
            "BACKFACE DEPTH" <- "backdepth"
          }
          frame "History" {
          }
          frame "System" {
          }
        }
        n56 = Get Date/Time String(want seconds? (F)=TRUE) -> (date string=w25:string, time string=w26:string)  [unwired: 2 in]
        n57 = call <vilib>:"Space Constant.vi"() -> ("String"=w23:string)
        n58 = Concatenate Strings(w25, w23, w26) -> (w24:string)
        n59 = local write "currentDateTime"(w24) -> ()
        n60 = Or(x="undoLastShot", y="deleteShot") -> (x .or. y?=w42:bool)
        n61 = Or(x="reportV50", y="reportV50_History") -> (x .or. y?=w50:bool)
        n62 = Build Array("RESET All", w50, "VsVr Report", "saveShots", "addShot", "clearShots", "nextShot", w42, "processShots", "readyClock") -> (w45:bool[])
        n63 = Search 1D Array(1D array=w45, element=w44) -> (index of element=w56:i32)  [unwired: 1 out]
        n64 = Increment(x=w56) -> (x+1=w57:i32)
        n65 = local read "SMErr"() -> (w27:errorcluster)
        n66 = Equal?(x=w57, y=w47) -> (x = y?=w48:bool)
        n67 = case shown="True" w48 {
          tunnel: w57 -> [w109 w121]
          tunnel: [w110 w126] -> w55
          tunnel: w27 -> [w108 w117]
          tunnel: [w108 w115] -> w28
          frame False {
            w112 = 0  # Not Found
            n68 = Equal?(x=w109, y=w112) -> (x = y?=w111:bool)
            n69 = case shown="True" w111 {
              tunnel: w109 -> [w113 _]
              tunnel: [w113 w114] -> w110
              frame False {
              }
              frame True {
                w114 = 11  # CheckDAQ
                # "USUAL SCENARIO"
              }
            }
          }
          frame True {
            # "Before allowing data record to be saved,\nprompt user to validate."
            n70 = call "Get Last Record (SubVI).vi"("error in"=w117) -> ("error out"=w116:errorcluster, "experiment record"=w118:i32, "shot record"=w119:i32)  [unwired: 2 out]
            n71 = local write "LastShot"(w119) -> ()
            n72 = local write "LastSample"(w118) -> ()
            n73 = To Double Precision Float(number=w118) -> (double precision float=w120:dbl)
            n74 = Two Button Dialog(message="Are ALL Data Valid?", 1:"NO" ("F button name (\"Cancel\")"), 2:"YES" ("T button name (\"OK\")")) -> (T button?=w125:bool)
            n75 = property on="Record #" class="DigNum (strict)"(error in=w116, "Maximum"=w120) -> (error out=w115:errorcluster)  [unwired: 1 in, 1 out]
            n76 = case shown="True" w125 {
              tunnel: [0 ("index of element") w128] -> w126
              tunnel: w121 -> [_ w128]
              frame False {
                # "POLL"
              }
              frame True {
              }
            }
          }
        }
        n77 = To Variant(anything=w55) -> (Variant=w53:variant)
        n78 = Variant To Data(type=w54, Variant=w53) -> (data=w38:T13)  [unwired: 1 in, 1 out]
        n79 = Wait (ms)(milliseconds to wait=u32 200 ("millisecond timer value")) -> ()  [unwired: 1 out]
        "STOP (Shots MC LB)" <- TRUE ("STOP (Shots MC LB)")
      }
      frame 1 {
        # "This section reads the ini file"
        n80 = case shown="100" w137 {
          tunnel: [w143 w162] -> w138
          tunnel: [w141 w162] -> w133
          tunnel: w130 -> [w140 w154]
          tunnel: [w139 w154] -> w129
          frame 0, Default {
            n81 = local read "RESET All"() -> (w142:bool)
            n82 = case shown="True" w142 {
              tunnel: [TRUE w150] -> w143
              tunnel: [FALSE w150] -> w141
              tunnel: w140 -> [w144 w147]
              tunnel: [w144 w147] -> w139
              frame False {
                # "Refresh"
              }
              frame True {
                n83 = Two Button Dialog(message="Resetting will remove all unsaved data.\n\nDo you really  want to reset? ", 1:"NO" ("F button name (\"Cancel\")"), 2:"YES" ("T button name (\"OK\")")) -> (T button?=w150:bool)
              }
            }
          }
          frame 100 {
            w162 = TRUE  # Reset ALL
            n84 = property on="Loading" class="Ring (strict)"("Visible"=FALSE) -> ()  [unwired: 2 in, 2 out]
            n85 = control-ref of="Mfr_0"() -> (w152:refnum<vi>)
            n86 = control-ref of="Mfr_1"() -> (w161:refnum<vi>)
            n87 = control-ref of="Mfr_2"() -> (w160:refnum<vi>)
            n88 = control-ref of="Mfr_3"() -> (w159:refnum<vi>)
            n89 = control-ref of="Mfr_4"() -> (w158:refnum<vi>)
            n90 = control-ref of="Mfr_5"() -> (w157:refnum<vi>)
            n91 = control-ref of="Mfr_6"() -> (w156:refnum<vi>)
            n92 = Build Array(w152, w161, w160, w159, w158, w157, w156) -> (w155:refnum<vi>[])
            n93 = global write "BIMS_Collector Globals.vi" "Mfrs"(w155) -> ()
          }
        }
        n94 = case shown="True" w138 {
          tunnel: [Collector_State."POLL" ("progState") w200] -> w136
          tunnel: w135 -> [w165 _]
          tunnel: [w165 "SHOTS"] -> w134
          tunnel: w133 -> [_ w201]
          tunnel: [w163 w180] -> w131
          tunnel: w129 -> [w163 w199]
          frame False {
            n95 = local write "RESET All"(FALSE ("RESET")) -> ()
          }
          frame True {
            n96 = case shown="True" w201 {
              selector: w201 -> [_ w231]
              tunnel: [w215 w231] -> w181
              tunnel: [w214 w246] -> w182
              tunnel: w199 -> [w214 w233]
              tunnel: [w213 w230] -> w178
              frame False {
                w215 = FALSE  # Reset All
                # "Refresh"
                n97 = local read "configPath"() -> (w213:path)
              }
              frame True {
                # "This section resets\nentire program"
                # "Reset ALL"
                n98 = control-ref of="This VI"() -> (w223:refnum<vi>)
                n99 = invoke on="Invoke Node" class="VI" method="Default Vals.Reinit All"(reference=w223, error in=w233) -> (reference out=w222:refnum<vi>, error out=w221:errorcluster)  [unwired: 1 in, 1 out]
                n100 = property class="VI"(reference=w222, error in=w221, "Front Panel.ShowMenuBar"=FALSE ("Front Panel Window:Show Menu Bar")) -> (reference out=w219:refnum<vi>, error out=w217:errorcluster)
                n101 = property on="mainTabCntrl" class="TabCtl (strict)"() -> (error out=w225:errorcluster, "Pages"=w227:refnum<vi>[])  [unwired: 2 in, 1 out]
                n102 = control-ref of="ScreenSetAvgg"() -> (w241:refnum<vi>)
                n103 = control-ref of="InterlockExists"() -> (w242:refnum<vi>)
                n104 = control-ref of="useBallisitican"() -> (w243:refnum<vi>)
                n105 = control-ref of="useRecorder"() -> (w244:refnum<vi>)
                n106 = control-ref of="useShooter"() -> (w245:refnum<vi>)
                n107 = control-ref of="useBMC"() -> (w216:refnum<vi>)
                n108 = Close Reference(reference=w219, error in (no error)=w217) -> (error out=w218:errorcluster)
                n109 = Index Array(array=w227, index=1) -> (element=w229:refnum<vi>)
                n110 = call "RegReadParams.vi"("ScreenSetAveraging_Ref"=w241, "useBMC_Ref"=w216, "InterlockExist_Ref"=w242, "errorIN"=w218, "useShooter_Ref"=w245, "useRecorder_Ref"=w244, "useBallistician_Ref"=w243) -> ("error out"=w240:errorcluster)  [unwired: 4 out]
                n111 = control-ref of="Server"() -> (w232:refnum<vi>)
                n112 = control-ref of="ConfigName"() -> (w236:refnum<vi>)
                n113 = control-ref of="Site"() -> (w234:refnum<vi>)
                n114 = property on="Property Node" class="Page"(reference=w229, error in=w225, "PageEnb"=T15."Page Disabled & Grayed" ("Page Enabled State")) -> (error out=w224:errorcluster)  [unwired: 1 out]
                n115 = Build Array(w236, w234, w232) -> (w237:refnum<vi>[])
                n116 = call "InitStringValuesFromRegistry(SubVI).vi"("error in"=w240, "String References"=w237, "subkey"="SOFTWARE\\DuPont\\BIMS-08\\Collector", "root key (HKEY_LOCAL_MACHINE)"=Registry_RtKey."HKEY_LOCAL_MACHINE") -> ("error out"=w239:errorcluster)  [unwired: 3 out]
                n117 = property on="minV50" class="DigNum (strict)"(error in=w224, "Visible"=w231) -> ()  [unwired: 1 in, 2 out]
                n118 = Current VI's Path() -> (path=w249:path)
                n119 = call "Initialize (SubVI).vi"("path"=w249, "error IN"=w239) -> ("pathConfigOUT"=w230:path, "lengthUnits"=→"lengthUnits":string, "massUnits"=→"massUnits":string, "error out"=w246:errorcluster)  [unwired: 1 out]
                "configPath" <- w230
              }
            }
            n120 = control-ref of="Threat"() -> (w185:refnum<vi>)
            n121 = control-ref of="SampleTypes"() -> (w187:refnum<vi>)
            n122 = control-ref of="SampleDescrip"() -> (w194:refnum<vi>)
            n123 = call "Get Threats (SubVI).vi"("pathConfigIN"=w178, "refThreat"=w185, "error in"=w182) -> ("pathConfigOUT"=w189:path, "factorOut"=→"factor array":sgl[], "error out"=w192:errorcluster)  [unwired: 4 out]
            n124 = Bundle("SampleTypes"=w187, "SampleDescrip"=w194) -> (w193:T21)  [unwired: 1 out]
            n125 = call "Fill Lists from INI (SubVI).vi"("clusterListboxes"=w193, "error in"=w192, "pathConfigIN"=w189) -> ("error out"=w191:errorcluster, "pathConfigOUT"=w190:path)  [unwired: 4 out]
            n126 = call "Read Parameters.vi"("error in (no error)"=w191, "appended path"=w190) -> ("error out"=w184:errorcluster, "rangeParams"=w186:T22)  [unwired: 4 out]
            n127 = Unbundle(w186) -> ("max dev"=w167:sgl, "residual separation"=→"Residual/Separation":sgl, "Set#1 Separation"=→"Set#1 Separation":sgl, "Set#2 Separation"=→"Set#2 Separation":sgl, "impact target dist"=w171:sgl, "resid target dist"=w172:sgl, "barrel screen dist"=→"Barrel to Screen":sgl, "midpt_to_target_dist"=→"mid_to_targ_dist":sgl)
            n128 = property on="Ballisticians" class="Ring (strict)"("Visible"="useBallisitican") -> ()  [unwired: 2 in, 2 out]
            n129 = property on="Shooters" class="Ring (strict)"("Visible"="useShooter") -> ()  [unwired: 2 in, 2 out]
            n130 = property on="Recorders" class="Ring (strict)"("Visible"="useRecorder") -> ()  [unwired: 2 in, 2 out]
            n131 = property on="RefreshMetadata" class="Bool (strict)"(error in=w184, "Val(Sgnl)"=TRUE) -> (error out=w179:errorcluster)  [unwired: 1 in, 1 out]
            n132 = local write "Residual/Target Dist"(w172) -> ()
            n133 = local write "maxDev"(w167) -> ()
            n134 = local write "Set#1_to_Target"(w171) -> ()
            n135 = disable-structure shown="Disabled" {
              disable-tunnel: w179 -> [w204 w206]
              disable-tunnel: [w203 w206] -> w175
              frame Disabled {
                n136 = property on="rangeSetup" class="Ring (strict)"(error in=w204, "Val(Sgnl)"=u16 1 ("Value (Signaling)")) -> (error out=w203:errorcluster)  [unwired: 1 in, 1 out]
              }
              frame Enabled {
              }
            }
            n137 = case shown="True" w181 {
              tunnel: [Collector_State."POLL" ("progState") w275] -> w200
              tunnel: [w250 w260] -> w198
              tunnel: w175 -> [w250 w269]
              tunnel: w178 -> [_ w259]
              tunnel: "useBMC" -> [_ w258]
              frame False {
                # "Refresh"
              }
              frame True {
                w252 = T14."Disabled and Grayed Out" ("Disabled")
                # "Reset ALL"
                n138 = global read "BIMS_Collector Globals.vi" "SampleStyles"() -> (w262:refnum<vi>[])
                n139 = case shown="True" w258 {
                  tunnel: w259 -> [_ w277]
                  frame False {
                  }
                  frame True {
                    n140 = Path To String(path=w277) -> (string=w278:string)
                    n141 = call "Ballistics Message Center.vi"("INI File Name"=w278) -> ()
                  }
                }
                n142 = call "Get Last Record (SubVI).vi"("error in"=w269) -> ("error out"=w261:errorcluster, "experiment record"=w267:i32, "shot record"=→"LastShot":i32)  [unwired: 2 out]
                "LastSample" <- w267
                n143 = local read "MeasSrc"() -> (w276:T6)
                n144 = local read "InterlockExists"() -> (w274:bool)
                n145 = control-ref of="ThreatDetails"() -> (w257:refnum<vi>)
                n146 = control-ref of="SampleStyle_0"() -> (w264:refnum<vi>)
                n147 = control-ref of="ThreatGroups"() -> (w263:refnum<vi>)
                n148 = local read "SafetyInterlock"() -> (w272:cluster{"ARMED":bool})
                n149 = Bundle By Name(cluster=w272, "ARMED"=FALSE) -> (w271:cluster{"ARMED":bool})
                n150 = To Double Precision Float(number=w267) -> (double precision float=w266:dbl)
                n151 = property on="Record #" class="DigNum (strict)"(error in=w261, "Maximum"=w266) -> (error out=w260:errorcluster)  [unwired: 1 in, 1 out]
                n152 = case shown="\"Screens\"" w276 {
                  tunnel: [Collector_State."POLL" ("progState") Collector_State."POLL" ("progState") Collector_State."READY CLOCK" ("progState")] -> w275
                  frame "Simulated", Default {
                  }
                  frame "Radar" {
                  }
                  frame "Screens" {
                    # "check for PCI 6602"
                  }
                }
                n153 = Build Array (concatenate)(w257, w264, w263, w262) -> (w265:refnum<vi>[])
                n154 = local write "SafetyInterlock"(w271) -> ()
                n155 = Select(t=T14."Enabled" ("Disabled"), s=w274, f=T14."Disabled and Grayed Out" ("Disabled")) -> (s? t:f=w273:T14)
                n156 = for {
                  tunnel: w265 -> [w279] mode=indexing
                  n157 = property on="Property Node" class="Ring (strict)"(reference=w279, "Strings []"=string[] []) -> ()  [unwired: 1 in, 2 out]
                }
                n158 = property on="addShot" class="Bool"("Disabled"=T14."Enabled") -> ()  [unwired: 2 in, 2 out]
                n159 = property on="undoLastShot" class="Bool"("Disabled"=w252) -> ()  [unwired: 2 in, 2 out]
                n160 = property on="saveShots" class="Bool"("Disabled"=w252) -> ()  [unwired: 2 in, 2 out]
                n161 = property on="clearShots" class="Bool"("Disabled"=w252) -> ()  [unwired: 2 in, 2 out]
                n162 = property on="ARM" class="Bool"("Disabled"=w273) -> ()  [unwired: 2 in, 2 out]
                n163 = property on="SafetyInterlock" class="Clust (strict)"("Disabled"=w273) -> ()  [unwired: 2 in, 2 out]
                n164 = property on="saveReq" class="Str"("Visible"=TRUE) -> ()  [unwired: 2 in, 2 out]
              }
            }
            n165 = call <vilib>:"General Error Handler.vi"("error in (no error)"=w198) -> ("error out"=w180:errorcluster)  [unwired: 2 in, 12 out]
            n166 = flat-sequence {
              tunnel: w180 -> [w207]
              frame #0 {
                n167 = local read "ConfigName"() -> (w208:string)
                n168 = case shown="No Error" w207 {
                  tunnel: [w211 "NOT READY!" ("ConfigName")] -> w209
                  tunnel: w208 -> [w211 _]
                  frame No Error {
                    n169 = Wait (ms)(milliseconds to wait=u32 1000) -> ()  [unwired: 1 out]
                  }
                  frame Error {
                  }
                }
                "ConfigName" <- w209
              }
            }
            "saveReq" <- "Number of layers in sample ply specification and number of shots in shots table must be greater than 0 to enable saving." ("saveReq")
          }
        }
      }
      frame 2 {
        w317 = TRUE  # Enable
        # "The custom Excel template file is \nexpected in the C:\\Ballistics folder."
        n170 = case shown="False" "lookupRec" {
          selector: "lookupRec" -> [_ w797]
          tunnel: [w334 w784] -> w315
          tunnel: [w333 w770] -> w314
          tunnel: [w332 w787] -> w313
          tunnel: [w331 w789] -> w312
          tunnel: [w330 w785] -> w311
          tunnel: [w329 w747] -> w310
          tunnel: [w328 w734] -> w297
          tunnel: [w327 w736] -> w296
          tunnel: [w326 w737] -> w295
          tunnel: [w325 "Record #"] -> w294
          tunnel: [w324 w786] -> w293
          tunnel: [w323 w736] -> w286
          tunnel: w291 -> [w322 _]
          tunnel: [w321 w759] -> w289
          tunnel: w288 -> [w321 w760]
          tunnel: [w320 w731] -> w284
          frame False {
            n171 = stacked-sequence {
              tunnel: [_ _ _ _ _ w657] -> w329
              tunnel: [_ w396 _ _ _ _] -> w333
              tunnel: [_ _ _ _ w501 _] -> w330
              tunnel: [_ _ _ w447 _ _] -> w331
              tunnel: [_ _ w418 _ _ _] -> w332
              tunnel: [w340 _ _ _ _ _] -> w334
              tunnel: [_ _ _ _ _ w663] -> w328
              tunnel: [_ _ _ _ _ w659] -> w327
              tunnel: [_ _ _ _ _ w658] -> w326
              tunnel: [_ _ _ _ _ w662] -> w325
              tunnel: [_ _ _ _ _ w661] -> w324
              tunnel: [_ _ _ _ _ w660] -> w323
              tunnel: w322 -> [_ _ w417 _ w500 _]
              frame #0 {
                # "FABRIC"
                n172 = local read "fab1_totalWt"() -> (w343:sgl)
                n173 = local read "fab3_totalWt"() -> (w345:sgl)
                n174 = local read "fab5_totalWt"() -> (w347:sgl)
                n175 = global read "BIMS_Collector Globals.vi" "LayerStitchTypeRefs"() -> (w335:refnum<vi>[])
                n176 = global read "BIMS_Collector Globals.vi" "SampleAttribs"() -> (w336:T23)
                n177 = global read "BIMS_Collector Globals.vi" "SampleStyles"() -> (w338:refnum<vi>[])
                n178 = global read "BIMS_Collector Globals.vi" "LayerSpecs"() -> (w337:T24)
                n179 = global read "BIMS_Collector Globals.vi" "Mfrs"() -> (w339:refnum<vi>[])
                n180 = local read "fab2_totalWt"() -> (w344:sgl)
                n181 = local read "fab4_totalWt"() -> (w346:sgl)
                n182 = local read "fab6_totalWt"() -> (w348:sgl)
                n183 = Build Array(w343, w344, w345, w346, w347, w348) -> (w342:sgl[])
                n184 = for {
                  tunnel: w342 -> [w350] mode=indexing
                  tunnel: [w356] -> w341 mode=indexing
                  tunnel: w336 -> [w354] mode=indexing
                  tunnel: w337 -> [w353] mode=indexing
                  tunnel: w339 -> [w352] mode=indexing
                  tunnel: w338 -> [w351] mode=indexing
                  tunnel: w335 -> [w349] mode=indexing
                  n185 = Less Or Equal To 0?(x=w350) -> (x <= 0?=w355:bool)
                  n186 = case shown="False" w355 {
                    tunnel: [w378 w380] -> w356
                    tunnel: w354 -> [w377 _]
                    tunnel: w353 -> [w362 _]
                    tunnel: w352 -> [w371 _]
                    tunnel: w351 -> [w368 _]
                    tunnel: w350 -> [w361 _]
                    tunnel: w349 -> [w357 _]
                    frame False {
                      n187 = Unbundle By Name(w362) -> ("numOfPlies"=w360:i32, "LotNum"=w374:string, "RollNum"=w375:string)
                      n188 = Unbundle By Name(w377) -> ("internal_ID"=w365:string, "fiber"=w366:string, "denier"=w373:string, "pick"=w372:string, "weave"=w363:string, "finish"=w364:string, "ozPerYd2"=w376:string)
                      n189 = Format Into String(w360) -> (resulting string=w370:string)  [unwired: 3 in, 1 out]
                      n190 = call "Dropdown Selection (SubVI).vi"("reference"=w371) -> ("element"=w369:string)
                      n191 = call "Dropdown Selection (SubVI).vi"("reference"=w368) -> ("element"=w367:string)
                      n192 = Format Into String(w361) -> (resulting string=w359:string)  [unwired: 3 in, 1 out]
                      n193 = call "Dropdown Selection (SubVI).vi"("reference"=w357) -> ("element"=w358:string)
                      n194 = Build Array(w370, w369, w367, w365, w366, w373, w372, w363, w364, w374, w375, w376, w359, w358) -> (w378:string[])
                    }
                    frame True {
                      n195 = call <vilib>:"Space Constant.vi"() -> ("String"=w381:string)
                      n196 = Initialize Array(w381, 12 ("dimension size")) -> (w380:string[])
                    }
                  }
                }
                n197 = Transpose 2D Array(2D array=w341) -> (transposed array=w340:string[][])
              }
              frame #1 {
                w382 = "%.1f" ("format string")
                # "muzzel / midpoint"
                # "muzzle / scr#1"
                # "muzzle / target"
                # "scr#2 / target"
                # "RANGE"
                n198 = local read "Set#1 Separation"() -> (w389:sgl)
                n199 = local read "mid_to_targ_dist"() -> (w386:sgl)
                n200 = local read "Barrel to Screen"() -> (w383:sgl)
                n201 = local read "clayAverage"() -> (w404:sgl)
                n202 = Divide(x=w389, y=sgl 2.0) -> (x/y=w384:sgl)
                n203 = local read "RoomHum"() -> (w399:sgl)
                n204 = local read "clayTemp"() -> (w402:sgl)
                n205 = local read "clayCalib"() -> (w405:string)
                n206 = local read "RoomT"() -> (w400:sgl)
                n207 = Add(x=w383, y=w386) -> (x+y=w390:sgl)
                n208 = Subtract(x=w383, y=w384) -> (x-y=w385:sgl)
                n209 = Subtract(x=w386, y=w384) -> (x-y=w387:sgl)
                n210 = Format Into String(w390) -> (resulting string=w391:string)  [unwired: 3 in, 1 out]
                n211 = Format Into String(w385) -> (resulting string=w392:string)  [unwired: 3 in, 1 out]
                n212 = Format Into String(w389) -> (resulting string=w393:string)  [unwired: 3 in, 1 out]
                n213 = Format Into String(w387) -> (resulting string=w394:string)  [unwired: 3 in, 1 out]
                n214 = Format Into String(w386) -> (resulting string=w395:string)  [unwired: 3 in, 1 out]
                n215 = Format Into String(w399) -> (resulting string=w397:string)  [unwired: 3 in, 1 out]
                n216 = Format Into String(format string=w382, w400) -> (resulting string=w398:string)  [unwired: 2 in, 1 out]
                n217 = Format Into String(format string=w382, w402) -> (resulting string=w401:string)  [unwired: 2 in, 1 out]
                n218 = Format Into String(format string=w382, w404) -> (resulting string=w403:string)  [unwired: 2 in, 1 out]
                n219 = Bundle(w391, w392, w393, w394, w395, w397, w398, w401, "clayCalib"=w405, w403) -> (w406:T25)  [unwired: 1 out]
                n220 = Cluster To Array(cluster=w406) -> (array=w396:string[])
              }
              frame #2 {
                # "RESULTS"
                n221 = control-ref of="Methods"() -> (w407:refnum<vi>)
                n222 = call "Dropdown Selection (SubVI).vi"("reference"=w407) -> ("element"=w408:string)
                n223 = for {
                  tunnel: w417 -> [w445] mode=indexing
                  tunnel: [w444] -> w416 mode=indexing
                  tunnel: [w443] -> w415
                  i -> [w443]
                  n224 = Unbundle By Name(w445) -> ("BackFace\nDepth"=w444:sgl)
                }
                n225 = Increment(x=w415) -> (x+1=w413:i32)
                n226 = Add Array Elements(numeric array=w416) -> (sum=w414:sgl)
                n227 = To Single Precision Float(number=w413) -> (single precision float=w412:sgl)
                n228 = Divide(x=w414, y=w412) -> (x/y=w411:sgl)
                n229 = Format Into String(format string="%1.1f", w411) -> (resulting string=w410:string)  [unwired: 2 in, 1 out]
                n230 = case shown="\"V50\"" w408 {
                  tunnel: [w433 w442] -> w420
                  tunnel: w410 -> [w421 w441]
                  frame "V50" {
                    w427 = "%1d" ("format string")
                    n231 = local read "Z.M.R."() -> (w425:sgl)
                    n232 = Less Than 0?(x=w425) -> (x < 0?=w426:bool)
                    n233 = local read "rangeOfResults"() -> (w429:i32)
                    n234 = local read "computed_V50"() -> (w432:sgl)
                    n235 = local read "lowComplete"() -> (w430:i32)
                    n236 = local read "highPartial"() -> (w431:i32)
                    n237 = case shown="True" w426 {
                      tunnel: w425 -> [w438 _]
                      tunnel: [w438 sgl 0.0 ("Z.M.R.")] -> w424
                      frame False {
                      }
                      frame True {
                      }
                    }
                    n238 = Format Into String(format string="%1.1f", w432) -> (resulting string=w436:string)  [unwired: 2 in, 1 out]
                    n239 = Format Into String(format string=w427, w431) -> (resulting string=w435:string)  [unwired: 2 in, 1 out]
                    n240 = Format Into String(format string=w427, w430) -> (resulting string=w434:string)  [unwired: 2 in, 1 out]
                    n241 = Format Into String(format string=w427, w429) -> (resulting string=w437:string)  [unwired: 2 in, 1 out]
                    n242 = Format Into String(format string="%1.1f", w424) -> (resulting string=w423:string)  [unwired: 2 in, 1 out]
                    n243 = Bundle(w436, w435, w434, w437, w423, w421, w421) -> (w433:T26)  [unwired: 1 out]
                  }
                  frame Default {
                    w440 = "" ("Empty String Constant")
                    n244 = Bundle(w440, w440, w440, w440, w440, w441, w441) -> (w442:T26)  [unwired: 1 out]
                  }
                }
                n245 = Cluster To Array(cluster=w420) -> (array=w419:string[])
                n246 = Build Array(w419) -> (w418:string[][])
              }
              frame #3 {
                # "SAMPLE"
                n247 = local read "Site"() -> (w446:string)
                n248 = case shown="\"SPR1\"" w446 {
                  tunnel: [w449 w473 w486] -> w447
                  frame "ICE1", Default {
                    # "PB Req"
                    n249 = control-ref of="Methods"() -> (w450:refnum<vi>)
                    n250 = call "Dropdown Selection (SubVI).vi"("reference"=w450) -> ("element"=w452:string)
                    n251 = Equal?(x=w452, y="V50") -> (x = y?=w451:bool)
                    n252 = local read "totalSampleWt"() -> (w462:sgl)
                    n253 = case shown="True" w451 {
                      tunnel: ["n/a" w472] -> w456
                      frame False {
                      }
                      frame True {
                        n254 = local read "minV50"() -> (w471:i32)
                        n255 = Format Into String(w471) -> (resulting string=w472:string)  [unwired: 3 in, 1 out]
                      }
                    }
                    n256 = control-ref of="SampleDimensions"() -> (w468:refnum<vi>)
                    n257 = control-ref of="SampleCoverings"() -> (w469:refnum<vi>)
                    n258 = control-ref of="Models"() -> (w455:refnum<vi>)
                    n259 = local read "serialNum"() -> (w464:string)
                    n260 = local read "SampleID"() -> (w466:string)
                    n261 = local read "Thickness"() -> (w459:dbl)
                    n262 = local read "totalBAW"() -> (w458:sgl)
                    n263 = call "Dropdown Selection (SubVI).vi"("reference"=w468) -> ("element"=w465:string)
                    n264 = call "Dropdown Selection (SubVI).vi"("reference"=w455) -> ("element"=w454:string)
                    n265 = call "Dropdown Selection (SubVI).vi"("reference"=w469) -> ("element"=w463:string)
                    n266 = Format Into String(w462) -> (resulting string=w461:string)  [unwired: 3 in, 1 out]
                    n267 = Format Into String(w459) -> (resulting string=w460:string)  [unwired: 3 in, 1 out]
                    n268 = Format Into String(w458) -> (resulting string=w457:string)  [unwired: 3 in, 1 out]
                    n269 = Bundle("SampleID"=w466, "element"=w465, "Type of work"="Type of work", "serialNum"=w464, "element"=w454, w461, w460, w457, "element"=w463, w456) -> (w467:T27)  [unwired: 1 out]
                    n270 = Cluster To Array(cluster=w467) -> (array=w449:string[])
                  }
                  frame "SPR0" {
                    n271 = local read "totalSampleWt"() -> (w479:sgl)
                    n272 = control-ref of="SampleDimensions"() -> (w484:refnum<vi>)
                    n273 = control-ref of="SampleCoverings"() -> (w485:refnum<vi>)
                    n274 = local read "SampleID"() -> (w482:string)
                    n275 = local read "Thickness"() -> (w476:dbl)
                    n276 = local read "totalBAW"() -> (w475:sgl)
                    n277 = call "Dropdown Selection (SubVI).vi"("reference"=w484) -> ("element"=w481:string)
                    n278 = call "Dropdown Selection (SubVI).vi"("reference"=w485) -> ("element"=w480:string)
                    n279 = Format Into String(w479) -> (resulting string=w478:string)  [unwired: 3 in, 1 out]
                    n280 = Format Into String(w476) -> (resulting string=w477:string)  [unwired: 3 in, 1 out]
                    n281 = Format Into String(w475) -> (resulting string=w474:string)  [unwired: 3 in, 1 out]
                    n282 = Bundle("SampleID"=w482, "element"=w481, w478, w477, w474, "element"=w480) -> (w483:T28)  [unwired: 1 out]
                    n283 = Cluster To Array(cluster=w483) -> (array=w473:string[])
                  }
                  frame "SPR1" {
                    n284 = local read "totalSampleWt"() -> (w492:sgl)
                    n285 = control-ref of="SampleDimensions"() -> (w497:refnum<vi>)
                    n286 = control-ref of="SampleCoverings"() -> (w498:refnum<vi>)
                    n287 = local read "SampleID"() -> (w495:string)
                    n288 = local read "Thickness"() -> (w489:dbl)
                    n289 = local read "totalBAW"() -> (w488:sgl)
                    n290 = call "Dropdown Selection (SubVI).vi"("reference"=w497) -> ("element"=w494:string)
                    n291 = call "Dropdown Selection (SubVI).vi"("reference"=w498) -> ("element"=w493:string)
                    n292 = Format Into String(w492) -> (resulting string=w491:string)  [unwired: 3 in, 1 out]
                    n293 = Format Into String(w489) -> (resulting string=w490:string)  [unwired: 3 in, 1 out]
                    n294 = Format Into String(w488) -> (resulting string=w487:string)  [unwired: 3 in, 1 out]
                    n295 = Bundle("SampleID"=w495, "element"=w494, w491, w490, w487, "element"=w493) -> (w496:T28)  [unwired: 1 out]
                    n296 = Cluster To Array(cluster=w496) -> (array=w486:string[])
                  }
                }
              }
              frame #4 {
                n297 = local read "Site"() -> (w499:string)
                n298 = case shown="\"ICE1\", Default" w499 {
                  tunnel: [w511 w561 w613] -> w501
                  tunnel: w500 -> [w504 w554 w606]
                  frame "ICE1", Default {
                    # "SHOT TABLE"
                    n299 = control-ref of="Methods"() -> (w503:refnum<vi>)
                    n300 = call "Dropdown Selection (SubVI).vi"("reference"=w503) -> ("element"=w502:string)
                    n301 = for {
                      tunnel: w504 -> [w543] mode=indexing
                      shift-right: [w520] -> _
                      shift-left: T17 [] -> [w522]
                      tunnel: [w520] -> w507
                      tunnel: w502 -> [w516]
                      n302 = Unbundle By Name(w543) -> ("shot order"=w542:i32, "Powder Loading"=w541:sgl, "Uncorrected Impact"=w540:sgl, "UncorrectedRed_PB"=w539:sgl, "UncorrectedAvgVel_PB"=w538:sgl, "velLoss_PB"=w537:sgl, "strikeVel_PB"=w536:sgl, "SHOT STATUS"=w525:u16, "usedv50"=w535:bool, "Shot Angle"=w517:u16, "BackFace\nDepth"=w518:sgl)
                      n303 = case shown="\"V50\"" w516 {
                        tunnel: w535 -> [w545 _]
                        tunnel: [w544 w549] -> w534
                        tunnel: w517 -> [_ w548]
                        frame "V50" {
                          n304 = case shown="True" w545 {
                            tunnel: ["" ("Empty String Constant") "*"] -> w544
                            frame False {
                            }
                            frame True {
                            }
                          }
                        }
                        frame Default {
                          n305 = Format Into String(w548) -> (resulting string=w549:string)  [unwired: 3 in, 1 out]
                        }
                      }
                      n306 = case shown="1" w525 {
                        tunnel: ["P" "C"] -> w524
                        frame 0, Default {
                        }
                        frame 1 {
                        }
                      }
                      n307 = Format Into String(format string="%2d", w542) -> (resulting string=w527:string)  [unwired: 2 in, 1 out]
                      n308 = Format Into String(w541) -> (resulting string=w528:string)  [unwired: 3 in, 1 out]
                      n309 = Format Into String(w540) -> (resulting string=w529:string)  [unwired: 3 in, 1 out]
                      n310 = Format Into String(w539) -> (resulting string=w530:string)  [unwired: 3 in, 1 out]
                      n311 = Format Into String(w538) -> (resulting string=w531:string)  [unwired: 3 in, 1 out]
                      n312 = Format Into String(w537) -> (resulting string=w532:string)  [unwired: 3 in, 1 out]
                      n313 = Format Into String(w536) -> (resulting string=w533:string)  [unwired: 3 in, 1 out]
                      n314 = Format Into String(w518) -> (resulting string=w526:string)  [unwired: 3 in, 1 out]
                      n315 = Build Array(w527, w528, w529, w530, w531, w532, w533, w524, w534, w526) -> (w521:string[])
                      n316 = Array To Cluster(array=w521) -> (cluster=w523:T29)
                      n317 = Build Array (concatenate)(w522, w523) -> (w520:T17)
                    }
                    n318 = Array Size(array=w507) -> (size(s)=w509:i32)
                    n319 = Equal To 0?(x=w509) -> (x = 0?=w505:bool)
                    n320 = case shown="True" w505 {
                      tunnel: [w512 T17 [{"[0]"="", "[1]"="", "[2]"="", "[3]"="", "[4]"="", "[5]"="", "[6]"="", "[7]"="", "[8]"="", "[9]"=""}]] -> w506
                      tunnel: w507 -> [w512 _]
                      frame False {
                      }
                      frame True {
                      }
                    }
                    n321 = Sort 1D Array(array=w506) -> (sorted array=w508:T17)
                    n322 = for {
                      tunnel: w508 -> [w515] mode=indexing
                      tunnel: [w514] -> w511 mode=indexing
                      n323 = Cluster To Array(cluster=w515) -> (array=w514:string[])
                    }
                  }
                  frame "SPR0" {
                    # "SHOT TABLE"
                    n324 = control-ref of="Methods"() -> (w553:refnum<vi>)
                    n325 = call "Dropdown Selection (SubVI).vi"("reference"=w553) -> ("element"=w552:string)
                    n326 = for {
                      tunnel: w554 -> [w591] mode=indexing
                      shift-right: [w572] -> _
                      shift-left: T18 [] -> [w574]
                      tunnel: [w572] -> w557
                      tunnel: w552 -> [w568]
                      n327 = Unbundle By Name(w591) -> ("shot order"=w590:i32, "Powder Loading"=w589:sgl, "Uncorrected Impact"=w588:sgl, "UncorrectedRed_PB"=w587:sgl, "strikeVel_PB"=w586:sgl, "SHOT STATUS"=w577:u16, "usedv50"=w585:bool, "Shot Angle"=w569:u16, "BackFace\nDepth"=w570:sgl, "V50userExcl"=w567:bool, "Shot Description"=w566:string)
                      n328 = case shown="\"V50\"" w568 {
                        tunnel: w585 -> [w594 _]
                        tunnel: [w593 w601] -> w584
                        tunnel: w569 -> [_ w600]
                        tunnel: w567 -> [w592 _]
                        frame "V50" {
                          n329 = case shown="True" w592 {
                            tunnel: w594 -> [w596 _]
                            tunnel: [w595 "!"] -> w593
                            frame False {
                              n330 = case shown="False" w596 {
                                tunnel: ["" ("Empty String Constant") "*"] -> w595
                                frame False {
                                }
                                frame True {
                                }
                              }
                            }
                            frame True {
                            }
                          }
                        }
                        frame Default {
                          n331 = Format Into String(w600) -> (resulting string=w601:string)  [unwired: 3 in, 1 out]
                        }
                      }
                      n332 = case shown="1" w577 {
                        tunnel: ["P" "C"] -> w576
                        frame 0, Default {
                        }
                        frame 1 {
                        }
                      }
                      n333 = Format Into String(format string="%2d", w590) -> (resulting string=w579:string)  [unwired: 2 in, 1 out]
                      n334 = Format Into String(w589) -> (resulting string=w580:string)  [unwired: 3 in, 1 out]
                      n335 = Format Into String(w588) -> (resulting string=w581:string)  [unwired: 3 in, 1 out]
                      n336 = Format Into String(w587) -> (resulting string=w582:string)  [unwired: 3 in, 1 out]
                      n337 = Format Into String(w586) -> (resulting string=w583:string)  [unwired: 3 in, 1 out]
                      n338 = Format Into String(w570) -> (resulting string=w578:string)  [unwired: 3 in, 1 out]
                      n339 = Build Array(w579, w580, w581, w582, w583, w576, w584, w578, w566) -> (w573:string[])
                      n340 = Array To Cluster(array=w573) -> (cluster=w575:T30)
                      n341 = Build Array (concatenate)(w574, w575) -> (w572:T18)
                    }
                    n342 = Array Size(array=w557) -> (size(s)=w559:i32)
                    n343 = Equal To 0?(x=w559) -> (x = 0?=w555:bool)
                    n344 = case shown="True" w555 {
                      tunnel: [w562 T18 [{"[0]"="", "[1]"="", "[2]"="", "[3]"="", "[4]"="", "[5]"="", "[6]"="", "[7]"="", "[8]"=""}]] -> w556
                      tunnel: w557 -> [w562 _]
                      frame False {
                      }
                      frame True {
                      }
                    }
                    n345 = Sort 1D Array(array=w556) -> (sorted array=w558:T18)
                    n346 = for {
                      tunnel: w558 -> [w565] mode=indexing
                      tunnel: [w564] -> w561 mode=indexing
                      n347 = Cluster To Array(cluster=w565) -> (array=w564:string[])
                    }
                  }
                  frame "SPR1" {
                    # "SHOT TABLE"
                    n348 = control-ref of="Methods"() -> (w605:refnum<vi>)
                    n349 = call "Dropdown Selection (SubVI).vi"("reference"=w605) -> ("element"=w604:string)
                    n350 = for {
                      tunnel: w606 -> [w643] mode=indexing
                      shift-right: [w624] -> _
                      shift-left: T18 [] -> [w626]
                      tunnel: [w624] -> w609
                      tunnel: w604 -> [w620]
                      n351 = Unbundle By Name(w643) -> ("shot order"=w642:i32, "Powder Loading"=w641:sgl, "Uncorrected Impact"=w640:sgl, "UncorrectedRed_PB"=w639:sgl, "strikeVel_PB"=w638:sgl, "SHOT STATUS"=w629:u16, "usedv50"=w637:bool, "Shot Angle"=w621:u16, "BackFace\nDepth"=w622:sgl, "V50userExcl"=w619:bool, "Shot Description"=w618:string)
                      n352 = case shown="\"V50\"" w620 {
                        tunnel: w637 -> [w646 _]
                        tunnel: [w645 w653] -> w636
                        tunnel: w621 -> [_ w652]
                        tunnel: w619 -> [w644 _]
                        frame "V50" {
                          n353 = case shown="True" w644 {
                            tunnel: w646 -> [w648 _]
                            tunnel: [w647 "!"] -> w645
                            frame False {
                              n354 = case shown="False" w648 {
                                tunnel: ["" ("Empty String Constant") "*"] -> w647
                                frame False {
                                }
                                frame True {
                                }
                              }
                            }
                            frame True {
                            }
                          }
                        }
                        frame Default {
                          n355 = Format Into String(w652) -> (resulting string=w653:string)  [unwired: 3 in, 1 out]
                        }
                      }
                      n356 = case shown="1" w629 {
                        tunnel: ["P" "C"] -> w628
                        frame 0, Default {
                        }
                        frame 1 {
                        }
                      }
                      n357 = Format Into String(format string="%2d", w642) -> (resulting string=w631:string)  [unwired: 2 in, 1 out]
                      n358 = Format Into String(w641) -> (resulting string=w632:string)  [unwired: 3 in, 1 out]
                      n359 = Format Into String(w640) -> (resulting string=w633:string)  [unwired: 3 in, 1 out]
                      n360 = Format Into String(w639) -> (resulting string=w634:string)  [unwired: 3 in, 1 out]
                      n361 = Format Into String(w638) -> (resulting string=w635:string)  [unwired: 3 in, 1 out]
                      n362 = Format Into String(w622) -> (resulting string=w630:string)  [unwired: 3 in, 1 out]
                      n363 = Build Array(w631, w632, w633, w634, w635, w628, w636, w630, w618) -> (w625:string[])
                      n364 = Array To Cluster(array=w625) -> (cluster=w627:T30)
                      n365 = Build Array (concatenate)(w626, w627) -> (w624:T18)
                    }
                    n366 = Array Size(array=w609) -> (size(s)=w611:i32)
                    n367 = Equal To 0?(x=w611) -> (x = 0?=w607:bool)
                    n368 = case shown="True" w607 {
                      tunnel: [w614 T18 [{"[0]"="", "[1]"="", "[2]"="", "[3]"="", "[4]"="", "[5]"="", "[6]"="", "[7]"="", "[8]"=""}]] -> w608
                      tunnel: w609 -> [w614 _]
                      frame False {
                      }
                      frame True {
                      }
                    }
                    n369 = Sort 1D Array(array=w608) -> (sorted array=w610:T18)
                    n370 = for {
                      tunnel: w610 -> [w617] mode=indexing
                      tunnel: [w616] -> w613 mode=indexing
                      n371 = Cluster To Array(cluster=w617) -> (array=w616:string[])
                    }
                  }
                }
              }
              frame #5 {
                n372 = local read "Site"() -> (w656:string)
                n373 = case shown="\"SPR1\"" w656 {
                  tunnel: [w687 w708 w728] -> w663
                  tunnel: [w686 w707 w727] -> w662
                  tunnel: [w685 w706 w726] -> w661
                  tunnel: [w684 w691 w711] -> w660
                  tunnel: ["" ("projNum") w691 w711] -> w659
                  tunnel: [w682 w705 w725] -> w658
                  tunnel: [w666 w694 w714] -> w657
                  frame "ICE1", Default {
                    # "THREAT"
                    # "Range # (supports a PB reporting requirement)"
                    # "Project Name goes here.\nSupports a PB reporting requirement."
                    # "GENERAL"
                    n374 = local read "threatDetails"() -> (w665:T1)
                    n375 = Unbundle By Name(w665) -> ("barrelLength"=w669:string)
                    n376 = Unbundle By Name(w665) -> ("grainSize"=w664:string)
                    n377 = local read "Shot Angle"() -> (w670:u16)
                    n378 = control-ref of="WeaponTypes"() -> (w679:refnum<vi>)
                    n379 = control-ref of="ThreatGroups"() -> (w678:refnum<vi>)
                    n380 = control-ref of="PowderTypes"() -> (w677:refnum<vi>)
                    n381 = control-ref of="Recorders"() -> (w680:refnum<vi>)
                    n382 = control-ref of="Shooters"() -> (w681:refnum<vi>)
                    n383 = Format Into String(w670) -> (resulting string=w671:string)  [unwired: 3 in, 1 out]
                    n384 = call "Dropdown Selection (SubVI).vi"("reference"=w679) -> ("element"=w675:string)
                    n385 = call "Dropdown Selection (SubVI).vi"("reference"=w678) -> ("element"=w674:string)
                    n386 = call "Dropdown Selection (SubVI).vi"("reference"=w677) -> ("element"=w673:string)
                    n387 = call "Dropdown Selection (SubVI).vi"("reference"=w680) -> ("element"=w672:string)
                    n388 = call "Dropdown Selection (SubVI).vi"("reference"=w681) -> ("element"=w668:string)
                    n389 = local read "Comments"() -> (w685:string)
                    n390 = local read "ProjectID"() -> (w682:string)
                    n391 = local read "LastSample"() -> (w690:i32)
                    n392 = Bundle("element"=w675, "element"=w674, "grainSize"=w664, "element"=w673, "barrelLength"=w669, w671, "element"="1", "element"=w668, "element"=w672) -> (w676:T31)  [unwired: 1 out]
                    n393 = control-ref of="TestStandards"() -> (w689:refnum<vi>)
                    n394 = control-ref of="Methods"() -> (w688:refnum<vi>)
                    n395 = Cluster To Array(cluster=w676) -> (array=w666:string[])
                    n396 = call "Dropdown Selection (SubVI).vi"("reference"=w689) -> ("element"=w684:string)
                    n397 = call "Dropdown Selection (SubVI).vi"("reference"=w688) -> ("element"=w687:string)
                    n398 = Increment(x=w690) -> (x+1=w686:i32)
                  }
                  frame "SPR0" {
                    w691 = "" ("projNum")
                    # "THREAT"
                    # "Project Name goes here.\nSupports a PB reporting requirement."
                    # "GENERAL"
                    n399 = local read "threatDetails"() -> (w693:T1)
                    n400 = Unbundle By Name(w693) -> ("barrelLength"=w696:string)
                    n401 = Unbundle By Name(w693) -> ("grainSize"=w692:string)
                    n402 = local read "Shot Angle"() -> (w697:u16)
                    n403 = control-ref of="ThreatGroups"() -> (w703:refnum<vi>)
                    n404 = control-ref of="PowderTypes"() -> (w702:refnum<vi>)
                    n405 = control-ref of="Ballisticians"() -> (w704:refnum<vi>)
                    n406 = Format Into String(w697) -> (resulting string=w698:string)  [unwired: 3 in, 1 out]
                    n407 = call "Dropdown Selection (SubVI).vi"("reference"=w703) -> ("element"=w700:string)
                    n408 = call "Dropdown Selection (SubVI).vi"("reference"=w702) -> ("element"=w699:string)
                    n409 = call "Dropdown Selection (SubVI).vi"("reference"=w704) -> ("element"=w695:string)
                    n410 = local read "Comments"() -> (w706:string)
                    n411 = local read "ProjectID"() -> (w705:string)
                    n412 = local read "LastSample"() -> (w710:i32)
                    n413 = Bundle("element"=w700, "grainSize"=w692, "element"=w699, "barrelLength"=w696, w698, "element"=w695) -> (w701:T32)  [unwired: 1 out]
                    n414 = control-ref of="Methods"() -> (w709:refnum<vi>)
                    n415 = Cluster To Array(cluster=w701) -> (array=w694:string[])
                    n416 = call "Dropdown Selection (SubVI).vi"("reference"=w709) -> ("element"=w708:string)
                    n417 = Increment(x=w710) -> (x+1=w707:i32)
                  }
                  frame "SPR1" {
                    w711 = "" ("projNum")
                    # "THREAT"
                    # "Project Name goes here.\nSupports a PB reporting requirement."
                    # "GENERAL"
                    n418 = local read "threatDetails"() -> (w713:T1)
                    n419 = Unbundle By Name(w713) -> ("barrelLength"=w716:string)
                    n420 = Unbundle By Name(w713) -> ("grainSize"=w712:string)
                    n421 = local read "Shot Angle"() -> (w717:u16)
                    n422 = control-ref of="ThreatGroups"() -> (w723:refnum<vi>)
                    n423 = control-ref of="PowderTypes"() -> (w722:refnum<vi>)
                    n424 = control-ref of="Ballisticians"() -> (w724:refnum<vi>)
                    n425 = Format Into String(w717) -> (resulting string=w718:string)  [unwired: 3 in, 1 out]
                    n426 = call "Dropdown Selection (SubVI).vi"("reference"=w723) -> ("element"=w720:string)
                    n427 = call "Dropdown Selection (SubVI).vi"("reference"=w722) -> ("element"=w719:string)
                    n428 = call "Dropdown Selection (SubVI).vi"("reference"=w724) -> ("element"=w715:string)
                    n429 = local read "Comments"() -> (w726:string)
                    n430 = local read "ProjectID"() -> (w725:string)
                    n431 = local read "LastSample"() -> (w730:i32)
                    n432 = Bundle("element"=w720, "grainSize"=w712, "element"=w719, "barrelLength"=w716, w718, "element"=w715) -> (w721:T32)  [unwired: 1 out]
                    n433 = control-ref of="Methods"() -> (w729:refnum<vi>)
                    n434 = Cluster To Array(cluster=w721) -> (array=w714:string[])
                    n435 = call "Dropdown Selection (SubVI).vi"("reference"=w729) -> ("element"=w728:string)
                    n436 = Increment(x=w730) -> (x+1=w727:i32)
                  }
                }
              }
            }
            n437 = Get Date/Time String() -> (date string=w320:string)  [unwired: 3 in, 1 out]
          }
          frame True {
            w736 = ""
            # "date"
            # "method"
            # "general"
            # "remark"
            # "threat"
            # "shots"
            # "sample"
            # "results"
            # "range"
            # "fabric"
            # "query db with the entered record number and use result to populate the xlt"
            n438 = Not(x=w797) -> (.not. x?=w796:bool)
            n439 = local write "lookupRec"(w796) -> ()
            n440 = Format Into String(format string="SELECT * FROM Experiments\nWHERE expt=%d;" ("query string"), error in=w760, "Record #") -> (resulting string=w793:string, error out=w761:errorcluster)  [unwired: 1 in]
            n441 = call "Fetch Data (SubVI).vi"("error IN"=w761, "query string"=w793) -> ("error OUT"=w759:errorcluster, "recordset data"=w795:string[][])  [unwired: 4 out]
            n442 = Index Array(array=w795) -> (element=w732:string[])  [unwired: 2 in]
            n443 = Index Array(array=w732, index=111) -> (element=w763:string)
            n444 = local read "Set#1 Separation"() -> (w777:sgl)
            n445 = call "Load Shots (SubVI).vi"("Record #"="Record #", "Method"=w763) -> ("Shot Array"=w785:string[][], "AvgDef"=w768:dbl)  [unwired: 1 in]
            n446 = local read "mid_to_targ_dist"() -> (w780:sgl)
            n447 = local read "Barrel to Screen"() -> (w783:sgl)
            n448 = Format Into String(w768) -> (resulting string=w766:string)  [unwired: 3 in, 1 out]
            n449 = Match Pattern(string=w763, regular expression="N.I.J.") -> (offset past match=w765:i32)  [unwired: 4 out]
            n450 = Greater Or Equal To 0?(x=w765) -> (x >= 0?=w762:bool)
            n451 = Divide(x=w777, y=sgl 2.0) -> (x/y=w782:sgl)
            n452 = case shown="False" w762 {
              tunnel: [w808 w809] -> w767
              tunnel: w766 -> [w805 w811]
              tunnel: w732 -> [w807 _]
              frame False {
                n453 = Index Array(array=w807, index #1=94 ("index"), index #2=119 ("index"), index #5=115 ("index")) -> (element #1=w806:string, element #2=w804:string, element #3=w803:string, element #4=w802:string, element #5=w801:string)  [unwired: 2 in]
                n454 = Build Array(w806, w804, w803, w802, w801, w805) -> (w808:string[])
              }
              frame True {
                w810 = "" ("Empty String Constant")
                n455 = Build Array(w810, w810, w810, w810, w810, w811, w811) -> (w809:string[])
              }
            }
            n456 = Add(x=w783, y=w780) -> (x+y=w776:sgl)
            n457 = Subtract(x=w783, y=w782) -> (x-y=w781:sgl)
            n458 = Subtract(x=w780, y=w782) -> (x-y=w779:sgl)
            n459 = Index Array(array=w732, index #1=91 ("index"), index #2=89 ("index"), index #3=97 ("index"), index #4=12 ("index"), index #5=7 ("index")) -> (element #1=w748:string, element #2=w746:string, element #3=w745:string, element #4=w742:string, element #5=w741:string)
            n460 = Index Array(array=w732, index #1=113 ("index"), index #2=112 ("index"), index #3=103 ("index")) -> (element #1=w757:string, element #2=w756:string, element #3=w755:string, element #4=w754:string, element #5=w750:string)  [unwired: 2 in]
            n461 = Format Into String(w776) -> (resulting string=w775:string)  [unwired: 3 in, 1 out]
            n462 = Format Into String(w781) -> (resulting string=w774:string)  [unwired: 3 in, 1 out]
            n463 = Format Into String(w777) -> (resulting string=w773:string)  [unwired: 3 in, 1 out]
            n464 = Format Into String(w779) -> (resulting string=w772:string)  [unwired: 3 in, 1 out]
            n465 = Format Into String(w780) -> (resulting string=w771:string)  [unwired: 3 in, 1 out]
            n466 = Build Array(w748, w746, w745, "", w742, w741) -> (w747:string[])
            n467 = Array Subset(array=w732, index=5, length=1) -> (w789:string[])
            n468 = Build Array(w775, w774, w773, w772, w771, w757, w756, w755, w754, w750) -> (w770:string[])
            n469 = Index Array(array=w732, index #1=4 ("index"), index #2=111 ("index")) -> (element #1=w737:string, element #2=w734:string)
            n470 = Index Array(array=w732, index=107) -> (element=w786:string)
            n471 = Index Array(array=w732, index=2) -> (element=w731:string)
            n472 = Build Array(w767) -> (w787:string[][])
            n473 = call "Get Model Construction.vi"("panel record"=w732) -> ("Fabric Array"=w784:string[][])
          }
        }
        n474 = To Variant(anything=w315) -> (Variant=w309:variant)
        n475 = To Variant(anything=w314) -> (Variant=w308:variant)
        n476 = To Variant(anything=w313) -> (Variant=w307:variant)
        n477 = To Variant(anything=w312) -> (Variant=w306:variant)
        n478 = To Variant(anything=w311) -> (Variant=w305:variant)
        n479 = To Variant(anything=w310) -> (Variant=w304:variant)
        n480 = To Variant(anything=w297) -> (Variant=w303:variant)
        n481 = To Variant(anything=w296) -> (Variant=w302:variant)
        n482 = To Variant(anything=w295) -> (Variant=w301:variant)
        n483 = To Variant(anything=w294) -> (Variant=w298:variant)
        n484 = To Variant(anything=w293) -> (Variant=w299:variant)
        n485 = To Variant(anything=w286) -> (Variant=w300:variant)
        n486 = To Variant(anything=w284) -> (Variant=w285:variant)
        n487 = call "TestReport_XL.vi"("Enable"=w317, "blockFabric"=w309, "blockRange"=w308, "blockResults"=w307, "blockSample"=w306, "blockShotTbl"=w305, "error in (no error)"=w289, "blockThreat"=w304, "testDate"=w285, "method"=w303, "projName"=w302, "projNum"=w301, "recNum"=w298, "remark"=w299, "standard"=w300) -> ("error out"=w316:errorcluster)  [unwired: 4 in, 8 out]
        n488 = call <vilib>:"Simple Error Handler.vi"("error in (no error)"=w316) -> ("error out"=w318:errorcluster)  [unwired: 1 in, 7 out]
        n489 = case shown="Error" w318 {
          selector: w318 -> [w812 w814]
          tunnel: [w812 w814] -> w287
          frame No Error {
            n490 = One Button Dialog(message=" V50 Ballistic Test Report is ready") -> ()  [unwired: 2 out]
          }
          frame Error {
          }
        }
      }
      frame 3 {
        w844 = TRUE  # Enable
        # "The custom Excel template file is \nexpected in the C:\\Ballistics folder."
        n491 = stacked-sequence {
          tunnel: [_ _ _ _ _ w1035] -> w837
          tunnel: [_ w908 _ _ _ _] -> w841
          tunnel: [_ _ _ _ w992 _] -> w838
          tunnel: [_ _ _ w959 _ _] -> w839
          tunnel: [_ _ w930 _ _ _] -> w840
          tunnel: [w852 _ _ _ _ _] -> w842
          tunnel: [_ _ _ _ _ w1056] -> w824
          tunnel: [_ _ _ _ _ "" ("projNum")] -> w823
          tunnel: [_ _ _ _ _ w1051] -> w822
          tunnel: [_ _ _ _ _ w1055] -> w821
          tunnel: [_ _ _ _ _ w1054] -> w820
          tunnel: [_ _ _ _ _ w1053] -> w819
          tunnel: w818 -> [_ _ w929 _ w985 _]
          frame #0 {
            # "FABRIC"
            n492 = local read "fab1_totalWt"() -> (w855:sgl)
            n493 = local read "fab3_totalWt"() -> (w857:sgl)
            n494 = local read "fab5_totalWt"() -> (w859:sgl)
            n495 = global read "BIMS_Collector Globals.vi" "LayerStitchTypeRefs"() -> (w847:refnum<vi>[])
            n496 = global read "BIMS_Collector Globals.vi" "SampleAttribs"() -> (w848:T23)
            n497 = global read "BIMS_Collector Globals.vi" "SampleStyles"() -> (w850:refnum<vi>[])
            n498 = local read "fab2_totalWt"() -> (w856:sgl)
            n499 = local read "fab4_totalWt"() -> (w858:sgl)
            n500 = local read "fab6_totalWt"() -> (w860:sgl)
            n501 = global read "BIMS_Collector Globals.vi" "LayerSpecs"() -> (w849:T24)
            n502 = global read "BIMS_Collector Globals.vi" "Mfrs"() -> (w851:refnum<vi>[])
            n503 = Build Array(w855, w856, w857, w858, w859, w860) -> (w854:sgl[])
            n504 = for {
              tunnel: w854 -> [w862] mode=indexing
              tunnel: [w868] -> w853 mode=indexing
              tunnel: w848 -> [w866] mode=indexing
              tunnel: w849 -> [w865] mode=indexing
              tunnel: w851 -> [w864] mode=indexing
              tunnel: w850 -> [w863] mode=indexing
              tunnel: w847 -> [w861] mode=indexing
              n505 = Less Or Equal To 0?(x=w862) -> (x <= 0?=w867:bool)
              n506 = case shown="False" w867 {
                tunnel: [w890 w892] -> w868
                tunnel: w866 -> [w889 _]
                tunnel: w865 -> [w874 _]
                tunnel: w864 -> [w883 _]
                tunnel: w863 -> [w880 _]
                tunnel: w862 -> [w873 _]
                tunnel: w861 -> [w869 _]
                frame False {
                  n507 = Unbundle By Name(w874) -> ("numOfPlies"=w872:i32, "LotNum"=w886:string, "RollNum"=w887:string)
                  n508 = Unbundle By Name(w889) -> ("internal_ID"=w877:string, "fiber"=w878:string, "denier"=w885:string, "pick"=w884:string, "weave"=w875:string, "finish"=w876:string, "ozPerYd2"=w888:string)
                  n509 = Format Into String(w872) -> (resulting string=w882:string)  [unwired: 3 in, 1 out]
                  n510 = call "Dropdown Selection (SubVI).vi"("reference"=w883) -> ("element"=w881:string)
                  n511 = call "Dropdown Selection (SubVI).vi"("reference"=w880) -> ("element"=w879:string)
                  n512 = call "Dropdown Selection (SubVI).vi"("reference"=w869) -> ("element"=w870:string)
                  n513 = Format Into String(w873) -> (resulting string=w871:string)  [unwired: 3 in, 1 out]
                  n514 = Build Array(w882, w881, w879, w877, w878, w885, w884, w875, w876, w886, w887, w888, w871, w870) -> (w890:string[])
                }
                frame True {
                  n515 = call <vilib>:"Space Constant.vi"() -> ("String"=w893:string)
                  n516 = Initialize Array(w893, 12 ("dimension size")) -> (w892:string[])
                }
              }
            }
            n517 = Transpose 2D Array(2D array=w853) -> (transposed array=w852:string[][])
          }
          frame #1 {
            w894 = "%.1f" ("format string")
            # "muzzel / midpoint"
            # "muzzle / scr#1"
            # "muzzle / target"
            # "scr#2 / target"
            # "RANGE"
            n518 = local read "Set#1 Separation"() -> (w901:sgl)
            n519 = local read "mid_to_targ_dist"() -> (w898:sgl)
            n520 = local read "Barrel to Screen"() -> (w895:sgl)
            n521 = local read "clayAverage"() -> (w916:sgl)
            n522 = Divide(x=w901, y=sgl 2.0) -> (x/y=w896:sgl)
            n523 = local read "RoomHum"() -> (w911:sgl)
            n524 = local read "clayTemp"() -> (w914:sgl)
            n525 = local read "clayCalib"() -> (w917:string)
            n526 = local read "RoomT"() -> (w912:sgl)
            n527 = Add(x=w895, y=w898) -> (x+y=w902:sgl)
            n528 = Subtract(x=w895, y=w896) -> (x-y=w897:sgl)
            n529 = Subtract(x=w898, y=w896) -> (x-y=w899:sgl)
            n530 = Format Into String(w902) -> (resulting string=w903:string)  [unwired: 3 in, 1 out]
            n531 = Format Into String(w897) -> (resulting string=w904:string)  [unwired: 3 in, 1 out]
            n532 = Format Into String(w901) -> (resulting string=w905:string)  [unwired: 3 in, 1 out]
            n533 = Format Into String(w899) -> (resulting string=w906:string)  [unwired: 3 in, 1 out]
            n534 = Format Into String(w898) -> (resulting string=w907:string)  [unwired: 3 in, 1 out]
            n535 = Format Into String(w911) -> (resulting string=w909:string)  [unwired: 3 in, 1 out]
            n536 = Format Into String(format string=w894, w912) -> (resulting string=w910:string)  [unwired: 2 in, 1 out]
            n537 = Format Into String(format string=w894, w914) -> (resulting string=w913:string)  [unwired: 2 in, 1 out]
            n538 = Format Into String(format string=w894, w916) -> (resulting string=w915:string)  [unwired: 2 in, 1 out]
            n539 = Bundle(w903, w904, w905, w906, w907, w909, w910, w913, "clayCalib"=w917, w915) -> (w918:T25)  [unwired: 1 out]
            n540 = Cluster To Array(cluster=w918) -> (array=w908:string[])
          }
          frame #2 {
            # "RESULTS"
            n541 = control-ref of="Methods"() -> (w919:refnum<vi>)
            n542 = call "Dropdown Selection (SubVI).vi"("reference"=w919) -> ("element"=w920:string)
            n543 = for {
              tunnel: w929 -> [w957] mode=indexing
              tunnel: [w956] -> w928 mode=indexing
              tunnel: [w955] -> w927
              i -> [w955]
              n544 = Unbundle By Name(w957) -> ("BackFace\nDepth"=w956:sgl)
            }
            n545 = Increment(x=w927) -> (x+1=w925:i32)
            n546 = Add Array Elements(numeric array=w928) -> (sum=w926:sgl)
            n547 = To Single Precision Float(number=w925) -> (single precision float=w924:sgl)
            n548 = Divide(x=w926, y=w924) -> (x/y=w923:sgl)
            n549 = Format Into String(format string="%1.1f", w923) -> (resulting string=w922:string)  [unwired: 2 in, 1 out]
            n550 = case shown="\"V50\"" w920 {
              tunnel: [w945 w954] -> w932
              tunnel: w922 -> [w933 w953]
              frame "V50" {
                w939 = "%1d" ("format string")
                n551 = local read "Z.M.R."() -> (w937:sgl)
                n552 = Less Than 0?(x=w937) -> (x < 0?=w938:bool)
                n553 = local read "rangeOfResults"() -> (w941:i32)
                n554 = local read "computed_V50"() -> (w944:sgl)
                n555 = local read "lowComplete"() -> (w942:i32)
                n556 = local read "highPartial"() -> (w943:i32)
                n557 = case shown="True" w938 {
                  tunnel: w937 -> [w950 _]
                  tunnel: [w950 sgl 0.0 ("Z.M.R.")] -> w936
                  frame False {
                  }
                  frame True {
                  }
                }
                n558 = Format Into String(format string="%1.1f", w944) -> (resulting string=w948:string)  [unwired: 2 in, 1 out]
                n559 = Format Into String(format string=w939, w943) -> (resulting string=w947:string)  [unwired: 2 in, 1 out]
                n560 = Format Into String(format string=w939, w942) -> (resulting string=w946:string)  [unwired: 2 in, 1 out]
                n561 = Format Into String(format string=w939, w941) -> (resulting string=w949:string)  [unwired: 2 in, 1 out]
                n562 = Format Into String(format string="%1.1f", w936) -> (resulting string=w935:string)  [unwired: 2 in, 1 out]
                n563 = Bundle(w948, w947, w946, w949, w935, w933, w933) -> (w945:T26)  [unwired: 1 out]
              }
              frame Default {
                w952 = "" ("Empty String Constant")
                n564 = Bundle(w952, w952, w952, w952, w952, w953, w953) -> (w954:T26)  [unwired: 1 out]
              }
            }
            n565 = Cluster To Array(cluster=w932) -> (array=w931:string[])
            n566 = Build Array(w931) -> (w930:string[][])
          }
          frame #3 {
            # "PB Req"
            # "SAMPLE"
            n567 = control-ref of="Methods"() -> (w960:refnum<vi>)
            n568 = call "Dropdown Selection (SubVI).vi"("reference"=w960) -> ("element"=w962:string)
            n569 = Equal?(x=w962, y="V50") -> (x = y?=w961:bool)
            n570 = local read "totalSampleWt"() -> (w972:sgl)
            n571 = case shown="True" w961 {
              tunnel: ["n/a" w982] -> w966
              frame False {
              }
              frame True {
                n572 = local read "minV50"() -> (w981:i32)
                n573 = Format Into String(w981) -> (resulting string=w982:string)  [unwired: 3 in, 1 out]
              }
            }
            n574 = local read "Type of work"() -> (w958:string)
            n575 = control-ref of="SampleDimensions"() -> (w978:refnum<vi>)
            n576 = control-ref of="SampleCoverings"() -> (w979:refnum<vi>)
            n577 = control-ref of="Models"() -> (w965:refnum<vi>)
            n578 = local read "serialNum"() -> (w974:string)
            n579 = local read "SampleID"() -> (w976:string)
            n580 = local read "Thickness"() -> (w969:dbl)
            n581 = local read "totalBAW"() -> (w968:sgl)
            n582 = call "Dropdown Selection (SubVI).vi"("reference"=w978) -> ("element"=w975:string)
            n583 = call "Dropdown Selection (SubVI).vi"("reference"=w965) -> ("element"=w964:string)
            n584 = call "Dropdown Selection (SubVI).vi"("reference"=w979) -> ("element"=w973:string)
            n585 = Format Into String(w972) -> (resulting string=w971:string)  [unwired: 3 in, 1 out]
            n586 = Format Into String(w969) -> (resulting string=w970:string)  [unwired: 3 in, 1 out]
            n587 = Format Into String(w968) -> (resulting string=w967:string)  [unwired: 3 in, 1 out]
            n588 = Bundle("SampleID"=w976, "element"=w975, "Type of work"=w958, "serialNum"=w974, "element"=w964, w971, w970, w967, "element"=w973, w966) -> (w977:T27)  [unwired: 1 out]
            n589 = Cluster To Array(cluster=w977) -> (array=w959:string[])
          }
          frame #4 {
            # "SHOT TABLE"
            n590 = control-ref of="Methods"() -> (w984:refnum<vi>)
            n591 = call "Dropdown Selection (SubVI).vi"("reference"=w984) -> ("element"=w983:string)
            n592 = for {
              tunnel: w985 -> [w1024] mode=indexing
              shift-right: [w1001] -> _
              shift-left: T17 [] -> [w1003]
              tunnel: [w1001] -> w988
              tunnel: w983 -> [w997]
              n593 = Unbundle By Name(w1024) -> ("shot order"=w1023:i32, "Powder Loading"=w1022:sgl, "Uncorrected Impact"=w1021:sgl, "UncorrectedRed_PB"=w1020:sgl, "UncorrectedAvgVel_PB"=w1019:sgl, "velLoss_PB"=w1018:sgl, "strikeVel_PB"=w1017:sgl, "SHOT STATUS"=w1006:u16, "usedv50"=w1016:bool, "Shot Angle"=w998:u16, "BackFace\nDepth"=w999:sgl)
              n594 = case shown="\"V50\"" w997 {
                tunnel: w1016 -> [w1026 _]
                tunnel: [w1025 w1030] -> w1015
                tunnel: w998 -> [_ w1029]
                frame "V50" {
                  n595 = case shown="True" w1026 {
                    tunnel: ["" ("Empty String Constant") "*"] -> w1025
                    frame False {
                    }
                    frame True {
                    }
                  }
                }
                frame Default {
                  n596 = Format Into String(w1029) -> (resulting string=w1030:string)  [unwired: 3 in, 1 out]
                }
              }
              n597 = case shown="1" w1006 {
                tunnel: ["P" "C"] -> w1005
                frame 0, Default {
                }
                frame 1 {
                }
              }
              n598 = Format Into String(format string="%2d", w1023) -> (resulting string=w1008:string)  [unwired: 2 in, 1 out]
              n599 = Format Into String(w1022) -> (resulting string=w1009:string)  [unwired: 3 in, 1 out]
              n600 = Format Into String(w1021) -> (resulting string=w1010:string)  [unwired: 3 in, 1 out]
              n601 = Format Into String(w1020) -> (resulting string=w1011:string)  [unwired: 3 in, 1 out]
              n602 = Format Into String(w1019) -> (resulting string=w1012:string)  [unwired: 3 in, 1 out]
              n603 = Format Into String(w1018) -> (resulting string=w1013:string)  [unwired: 3 in, 1 out]
              n604 = Format Into String(w1017) -> (resulting string=w1014:string)  [unwired: 3 in, 1 out]
              n605 = Format Into String(w999) -> (resulting string=w1007:string)  [unwired: 3 in, 1 out]
              n606 = Build Array(w1008, w1009, w1010, w1011, w1012, w1013, w1014, w1005, w1015, w1007) -> (w1002:string[])
              n607 = Array To Cluster(array=w1002) -> (cluster=w1004:T29)
              n608 = Build Array (concatenate)(w1003, w1004) -> (w1001:T17)
            }
            n609 = Array Size(array=w988) -> (size(s)=w990:i32)
            n610 = Equal To 0?(x=w990) -> (x = 0?=w986:bool)
            n611 = case shown="True" w986 {
              tunnel: [w993 T17 [{"[0]"="", "[1]"="", "[2]"="", "[3]"="", "[4]"="", "[5]"="", "[6]"="", "[7]"="", "[8]"="", "[9]"=""}]] -> w987
              tunnel: w988 -> [w993 _]
              frame False {
              }
              frame True {
              }
            }
            n612 = Sort 1D Array(array=w987) -> (sorted array=w989:T17)
            n613 = for {
              tunnel: w989 -> [w996] mode=indexing
              tunnel: [w995] -> w992 mode=indexing
              n614 = Cluster To Array(cluster=w996) -> (array=w995:string[])
            }
          }
          frame #5 {
            # "THREAT"
            # "Range # (supports a PB reporting requirement)"
            # "Project Name goes here.\nSupports a PB reporting requirement."
            # "GENERAL"
            n615 = local read "threatDetails"() -> (w1034:T1)
            n616 = Unbundle By Name(w1034) -> ("barrelLength"=w1038:string)
            n617 = Unbundle By Name(w1034) -> ("grainSize"=w1033:string)
            n618 = local read "Shot Angle"() -> (w1039:u16)
            n619 = control-ref of="WeaponTypes"() -> (w1048:refnum<vi>)
            n620 = control-ref of="ThreatGroups"() -> (w1047:refnum<vi>)
            n621 = control-ref of="PowderTypes"() -> (w1046:refnum<vi>)
            n622 = control-ref of="Recorders"() -> (w1049:refnum<vi>)
            n623 = control-ref of="Shooters"() -> (w1050:refnum<vi>)
            n624 = Format Into String(w1039) -> (resulting string=w1040:string)  [unwired: 3 in, 1 out]
            n625 = call "Dropdown Selection (SubVI).vi"("reference"=w1048) -> ("element"=w1044:string)
            n626 = call "Dropdown Selection (SubVI).vi"("reference"=w1047) -> ("element"=w1043:string)
            n627 = call "Dropdown Selection (SubVI).vi"("reference"=w1046) -> ("element"=w1042:string)
            n628 = call "Dropdown Selection (SubVI).vi"("reference"=w1049) -> ("element"=w1041:string)
            n629 = call "Dropdown Selection (SubVI).vi"("reference"=w1050) -> ("element"=w1037:string)
            n630 = Bundle("element"=w1044, "element"=w1043, "grainSize"=w1033, "element"=w1042, "barrelLength"=w1038, w1040, "element"="1", "element"=w1037, "element"=w1041) -> (w1045:T31)  [unwired: 1 out]
            n631 = Cluster To Array(cluster=w1045) -> (array=w1035:string[])
            n632 = local read "Comments"() -> (w1054:string)
            n633 = local read "ProjectID"() -> (w1051:string)
            n634 = local read "LastSample"() -> (w1059:i32)
            n635 = control-ref of="TestStandards"() -> (w1058:refnum<vi>)
            n636 = control-ref of="Methods"() -> (w1057:refnum<vi>)
            n637 = call "Dropdown Selection (SubVI).vi"("reference"=w1058) -> ("element"=w1053:string)
            n638 = call "Dropdown Selection (SubVI).vi"("reference"=w1057) -> ("element"=w1056:string)
            n639 = Increment(x=w1059) -> (x+1=w1055:i32)
          }
        }
        n640 = To Variant(anything=w842) -> (Variant=w836:variant)
        n641 = To Variant(anything=w841) -> (Variant=w835:variant)
        n642 = To Variant(anything=w840) -> (Variant=w834:variant)
        n643 = To Variant(anything=w839) -> (Variant=w833:variant)
        n644 = To Variant(anything=w838) -> (Variant=w832:variant)
        n645 = To Variant(anything=w837) -> (Variant=w831:variant)
        n646 = To Variant(anything=w824) -> (Variant=w830:variant)
        n647 = To Variant(anything=w823) -> (Variant=w829:variant)
        n648 = To Variant(anything=w822) -> (Variant=w828:variant)
        n649 = To Variant(anything=w821) -> (Variant=w825:variant)
        n650 = To Variant(anything=w820) -> (Variant=w826:variant)
        n651 = To Variant(anything=w819) -> (Variant=w827:variant)
        n652 = call "TestReport_XL.vi"("Enable"=w844, "blockFabric"=w836, "blockRange"=w835, "blockResults"=w834, "blockSample"=w833, "blockShotTbl"=w832, "error in (no error)"=w816, "blockThreat"=w831, "method"=w830, "projName"=w829, "projNum"=w828, "recNum"=w825, "remark"=w826, "standard"=w827) -> ("error out"=w843:errorcluster)  [unwired: 5 in, 8 out]
        n653 = call <vilib>:"Simple Error Handler.vi"("error in (no error)"=w843) -> ("error out"=w845:errorcluster)  [unwired: 1 in, 7 out]
        n654 = case shown="No Error" w845 {
          selector: w845 -> [w1060 w1062]
          tunnel: [w1060 w1062] -> w815
          frame No Error {
            n655 = One Button Dialog(message=" VsVr Ballistic Test Report is ready") -> ()  [unwired: 2 out]
          }
          frame Error {
          }
        }
      }
      frame 4 {
        # "This section saves the shots to the data base"
        n656 = stacked-sequence {
          seq-local: [w1128 _ _] -> [_ w1214 _]
          seq-local: [w1130 _ _] -> [_ w1211 _]
          seq-local: [_ w1199 _] -> [_ _ w1228]
          seq-local: [_ w1201 _] -> [_ _ w1227]
          seq-local: [w1126 _ _] -> [_ _ w1220]
          seq-local: [w1100 _ _] -> [_ w1157 _]
          tunnel: [_ _ w1222] -> w1068
          tunnel: [_ _ w1225] -> w1069
          tunnel: w1064 -> [_ w1166 w1219]
          tunnel: w1066 -> [w1102 _ _]
          tunnel: ["SampleDescrip" _ _] -> _
          tunnel: ["Areal Density" _ _] -> _
          tunnel: ["Areal density text" _ _] -> _
          tunnel: ["SoftwareVersion" _ _] -> _
          tunnel: ["Fabric Description" _ _] -> _
          tunnel: ["Threat" _ _] -> _
          tunnel: ["old threat" _ _] -> _
          tunnel: ["line direction map" _ _] -> _
          tunnel: ["Methods" _ _] -> _
          tunnel: ["SampleCoverings" _ _] -> _
          tunnel: ["Ballisticians" _ _] -> _
          tunnel: ["Submitters" _ _] -> _
          tunnel: ["SampleDimensions" _ _] -> _
          tunnel: ["PowderTypes" _ _] -> _
          tunnel: ["SampleTypes" _ _] -> _
          tunnel: ["TestConditions" _ _] -> _
          tunnel: ["ModelMfrs" _ _] -> _
          tunnel: ["Assemblers" _ _] -> _
          tunnel: ["N.I.J" _ _] -> _
          tunnel: ["SampleClamping" _ _] -> _
          tunnel: ["FrontLayer" _ _] -> _
          tunnel: ["BackLayer" _ _] -> _
          frame #0 {
            # "Legacy requirements:"
            # "Shared requirements:"
            n657 = local read "fab1_totalWt"() -> (w1138:sgl)
            n658 = local read "fab2_totalWt"() -> (w1137:sgl)
            n659 = local read "fab3_totalWt"() -> (w1136:sgl)
            n660 = local read "fab4_totalWt"() -> (w1135:sgl)
            n661 = local read "fab5_totalWt"() -> (w1134:sgl)
            n662 = local read "fab6_totalWt"() -> (w1133:sgl)
            n663 = Build Array(w1138, w1137, w1136, w1135, w1134, w1133) -> (w1132:sgl[])
            n664 = call "SQL Statement for Sample Descritpion.vi"("error IN"=w1102, "Layer Weight Array"=w1132, "VALUES clause IN"=" VALUES (%d " ("SQL statement IN"), "INSERT clause IN"="INSERT INTO Experiments " ("SQL statement IN")) -> ("error OUT"=w1101:errorcluster, "VALUES clause OUT"=w1131:string, "INSERT clause OUT"=w1129:string)  [unwired: 1 out]
            n665 = local read "LastSample"() -> (w1127:i32)
            n666 = Increment(x=w1127) -> (x+1=w1126:i32)
            n667 = local read "rangeOfResults"() -> (w1104:i32)
            n668 = local read "lowComplete"() -> (w1105:i32)
            n669 = local read "clayAverage"() -> (w1107:sgl)
            n670 = local read "highPartial"() -> (w1106:i32)
            n671 = control-ref of="SampleClamping"() -> (w1099:refnum<vi>)
            n672 = control-ref of="BackLayer"() -> (w1075:refnum<vi>)
            n673 = control-ref of="FrontLayer"() -> (w1074:refnum<vi>)
            n674 = control-ref of="Ballisticians"() -> (w1121:refnum<vi>)
            n675 = control-ref of="Shooters"() -> (w1117:refnum<vi>)
            n676 = control-ref of="Recorders"() -> (w1116:refnum<vi>)
            n677 = control-ref of="Submitters"() -> (w1120:refnum<vi>)
            n678 = control-ref of="SampleCoverings"() -> (w1113:refnum<vi>)
            n679 = control-ref of="ThreatGroups"() -> (w1112:refnum<vi>)
            n680 = call "Dropdown Selection (SubVI).vi"("reference"=w1121) -> ("element"=w1119:string)
            n681 = call "Dropdown Selection (SubVI).vi"("reference"=w1117) -> ("element"=w1115:string)
            n682 = call "Dropdown Selection (SubVI).vi"("reference"=w1116) -> ("element"=w1114:string)
            n683 = call "Dropdown Selection (SubVI).vi"("reference"=w1120) -> ("element"=w1118:string)
            n684 = call "Dropdown Selection (SubVI).vi"("reference"=w1113) -> ("element"=w1111:string)
            n685 = call "Dropdown Selection (SubVI).vi"("reference"=w1112) -> ("element"=w1110:string)
            n686 = call "Dropdown Selection (SubVI).vi"("reference"=w1099) -> ("element"=w1098:string)
            n687 = call "Dropdown Selection (SubVI).vi"("reference"=w1075) -> ("element"=w1073:string)
            n688 = call "Dropdown Selection (SubVI).vi"("reference"=w1074) -> ("element"=w1072:string)
            n689 = flat-sequence {
              tunnel: ["TestStandards"] -> _
              tunnel: ["Shooters"] -> _
              tunnel: ["Recorders"] -> _
              tunnel: ["WeaponTypes"] -> _
              tunnel: ["Models"] -> _
              tunnel: ["serialNum"] -> _
              tunnel: ["layerStitch_1"] -> _
              tunnel: ["layerStitch_2"] -> _
              tunnel: ["layerStitch_3"] -> _
              tunnel: ["layerStitch_4"] -> _
              tunnel: ["layerStitch_5"] -> _
              tunnel: ["layerStitch_6"] -> _
              tunnel: ["minV50"] -> _
              frame #0 {
                # "PB-only requirements:"
              }
            }
            n690 = Concatenate Strings(w1129, ", expt, [date], Ballistician1, Ballistician2, Ballistician3, Submitter1, SampleCovering, ProjectileType, ClayTemp, ClayCalibration, ClayAvgThickness, highPartial, lowComplete, rangeOfResults, clamping, FrontPly, BackPly," ("Substring")) -> (w1128:string)
            n691 = Format Into String(format string=", %d, #%s#, '%s', '%s', '%s', '%s', '%s', '%s', %.1f, '%s', %.1f, %d, %d, %d, '%s', '%s', '%s'" ("Format String"), initial string=w1131, error in=w1101, w1126, "currentDateTime", w1119, w1115, w1114, w1118, w1111, w1110, "clayTemp", "clayCalib", w1107, w1106, w1105, w1104, w1098, w1073, w1072) -> (resulting string=w1130:string, error out=w1100:errorcluster)
          }
          frame #1 {
            w1213 = " Angle, Conditions, SampleType, ThreatGrain, ThreatDetail, V50dc, V50, maker, thickness, powder, numshots, backing, totalnumberplys, testcomments, NIJ1, method, temperature, humidity, Dimensions, zmr, ProjectID, SampleID, panelmaker, panelWeight, totalBAW)"  # INSERT clause continued
            # "Although shot angle is defined for the overall\nexperiment, it is also recorded for each shot."
            n692 = local read "computed_V50"() -> (w1209:sgl)
            n693 = local read "Drag Corrected"() -> (w1204:bool)
            n694 = local read "Impact factor"() -> (w1206:sgl)
            n695 = Array Size(array=w1166) -> (size(s)=w1197:i32)
            n696 = Select(t=w1206, s=w1204, f=sgl 1.0) -> (s? t:f=w1205:sgl)
            n697 = Divide(x=w1209, y=w1205) -> (x/y=w1208:sgl)
            n698 = control-ref of="ModelMfrs"() -> (w1192:refnum<vi>)
            n699 = control-ref of="PowderTypes"() -> (w1190:refnum<vi>)
            n700 = call "Dropdown Selection (SubVI).vi"("reference"=w1192) -> ("element"=w1191:string)
            n701 = call "Dropdown Selection (SubVI).vi"("reference"=w1190) -> ("element"=w1174:string)
            n702 = local read "GrainSize"() -> (w1155:u16)
            n703 = local read "Z.M.R."() -> (w1180:sgl)
            n704 = local read "Shot Angle"() -> (w1168:u16)
            n705 = Less Than 0?(x=w1180) -> (x < 0?=w1179:bool)
            n706 = local read "totalNumLayers"() -> (w1196:i32)
            n707 = control-ref of="ThreatDetails"() -> (w1152:refnum<vi>)
            n708 = control-ref of="SampleTypes"() -> (w1162:refnum<vi>)
            n709 = control-ref of="TestConditions"() -> (w1181:refnum<vi>)
            n710 = control-ref of="SampleBackings"() -> (w1189:refnum<vi>)
            n711 = Format Into String(w1155) -> (resulting string=w1154:string)  [unwired: 3 in, 1 out]
            n712 = local read "totalBAW"() -> (w1182:sgl)
            n713 = case shown="True" w1179 {
              tunnel: w1180 -> [w1217 _]
              tunnel: [w1217 sgl 0.0 ("Z.M.R.")] -> w1178
              frame False {
              }
              frame True {
              }
            }
            n714 = control-ref of="SampleDimensions"() -> (w1185:refnum<vi>)
            n715 = control-ref of="N.I.J"() -> (w1187:refnum<vi>)
            n716 = control-ref of="Methods"() -> (w1172:refnum<vi>)
            n717 = control-ref of="Assemblers"() -> (w1183:refnum<vi>)
            n718 = call "Dropdown Selection (SubVI).vi"("reference"=w1152) -> ("element"=w1153:string)
            n719 = call "Dropdown Selection (SubVI).vi"("reference"=w1162) -> ("element"=w1161:string)
            n720 = call "Dropdown Selection (SubVI).vi"("reference"=w1181) -> ("element"=w1167:string)
            n721 = call "Dropdown Selection (SubVI).vi"("reference"=w1189) -> ("element"=w1188:string)
            n722 = Equal?(x=w1154, y="") -> (x = y?=w1176:bool)
            n723 = call "Dropdown Selection (SubVI).vi"("reference"=w1187) -> ("element"=w1186:string)
            n724 = call "Dropdown Selection (SubVI).vi"("reference"=w1172) -> ("element"=w1171:string)
            n725 = call "Dropdown Selection (SubVI).vi"("reference"=w1185) -> ("element"=w1184:string)
            n726 = call "Dropdown Selection (SubVI).vi"("reference"=w1183) -> ("element"=w1173:string)
            n727 = case shown="False" w1176 {
              tunnel: [w1215 "0" ("element")] -> w1175
              tunnel: w1154 -> [w1215 _]
              frame False {
              }
              frame True {
              }
            }
            n728 = call "Prepare DB Connect Path (SubVI).vi"("connectString"=path "BIMS_Collector.udl", "error in"=w1157) -> ("appended path"=w1156:path, "error out"=w1158:errorcluster)  [unwired: 1 out]
            n729 = Format Into String(format string=", %d, '%s', '%s', '%s', '%s', %.4f, %.1f, '%s', %.4f, '%s', %d, '%s', %d, '%s', '%s', '%s', %.1f, %.1f, '%s', %.1f, '%s', '%s', '%s', %.1f, %.1f);" ("Format String"), initial string=w1211, error in=w1158, w1168, w1167, w1161, w1175, w1153, w1209, w1208, w1191, "Thickness", w1174, w1197, w1188, w1196, "Comments", w1186, w1171, "RoomT", "RoomHum", w1184, w1178, "ProjectID", "SampleID", w1173, "totalSampleWt", w1182) -> (resulting string=w1210:string, error out=w1160:errorcluster)
            n730 = call-poly <vilib>:"DB Tools Open Connection.vi"("error in (no error)"=w1160, "connection information"=w1156) -> ("error out"=w1169:errorcluster, "connection reference"=w1170:T33)  [unwired: 3 in, 3 out]
            n731 = Concatenate Strings(w1214, w1213, w1210) -> (w1203:string)
            n732 = call-poly <vilib>:"DB Tools Execute Query.vi"("error in (no error)"=w1169, "SQL query"=w1203, "connection reference"=w1170) -> ("error out"=w1202:errorcluster, "recordset reference"=w1200:T34)  [unwired: 1 in, 4 out]
            n733 = call-poly <vilib>:"DB Tools Free Object.vi"("error in (no error)"=w1202, "recordset reference"=w1200) -> ("error out"=w1201:errorcluster, "connection reference"=w1199:T33)  [unwired: 8 out]
          }
          frame #2 {
            # "Experiment.expt"
            n734 = local read "LastShot"() -> (w1226:i32)
            n735 = Increment(x=w1226) -> (x+1=w1224:i32)
            n736 = for {
              tunnel: w1219 -> [w1272] mode=indexing
              tunnel: w1228 -> [w1247]
              tunnel: w1227 -> [w1231]
              tunnel: [w1245] -> w1221
              tunnel: [w1246] -> w1223
              tunnel: w1224 -> [w1252]
              tunnel: [w1244] -> w1225
              tunnel: w1220 -> [w1240]
              i -> [w1244]
              w1232 = sgl 1.0 ("f")
              # "Shot.id"
              n737 = Add(x=w1252, y=w1244) -> (x+y=w1251:i32)
              n738 = Unbundle By Name(w1272) -> ("IMPACT VELOCITY"=w1258:sgl, "Redundant_Velocity"=w1237:sgl, "RESIDUAL  VELOCITY"=w1236:sgl, "Shot Description"=w1238:string, "Powder Loading"=w1262:sgl, "Barrel Temperature"=w1263:sgl, "TIME / DATE"=w1264:string, "shot order"=w1265:i32, "Shot Angle"=w1266:u16, "BackFace\nDepth"=w1267:sgl, "BackFace\nDiameter"=w1268:sgl, "SHOT STATUS"=w1270:u16, "Projectile Mass"=w1261:sgl, "usedv50"=w1260:bool, "Energy Loss (J)"=w1259:sgl, "avgVel_PB"=w1243:sgl, "velLoss_PB"=w1242:sgl, "strikeVel_PB"=w1241:sgl, "Frag Rod"=w1229:sgl)
              n739 = local read "Drag Corrected"() -> (w1234:bool)
              n740 = local read "Residual factor"() -> (w1256:sgl)
              n741 = local read "Impact factor"() -> (w1233:sgl)
              n742 = Greater Than 0?(x=w1270) -> (x > 0?=w1269:bool)
              n743 = Select(t=w1233, s=w1234, f=w1232) -> (s? t:f=w1254:sgl)
              n744 = Select(t=w1233, s=w1234, f=w1232) -> (s? t:f=w1239:sgl)
              n745 = Select(t=w1256, s=w1234, f=w1232) -> (s? t:f=w1255:sgl)
              n746 = Divide(x=w1258, y=w1254) -> (x/y=w1253:sgl)
              n747 = Divide(x=w1237, y=w1239) -> (x/y=w1235:sgl)
              n748 = Divide(x=w1236, y=w1255) -> (x/y=w1257:sgl)
              n749 = Format Into String(format string="INSERT INTO shots (impactdc, redundantdc, residualdc,  comment, loading, barreltemp, [date], [order], shotangle, bfdepth, bfdiameter, [complete], expt, id, weight,usedv50, loss, residual, impact, redundant, avgVel_PB, velLoss_PB, strikeVel_PB, fragRod)  VALUES (%.1f, %.1f, %.1f, '%s', %.4f, %.1f, #%s#, %d, %d, %.3f, %.3f, %d, %d, %d, %.4f, %d, %.4f, %.1f, %.1f, %.1f, %.1f, %.1f, %.1f, %.1f)" ("Substring"), error in=w1231, w1258, w1237, w1236, w1238, w1262, w1263, w1264, w1265, w1266, w1267, w1268, w1269, w1240, w1251, w1261, w1260, w1259, w1257, w1253, w1235, w1243, w1242, w1241, w1229) -> (resulting string=w1248:string, error out=w1230:errorcluster)  [unwired: 1 in]
              n750 = call-poly <vilib>:"DB Tools Execute Query.vi"("error in (no error)"=w1230, "SQL query"=w1248, "connection reference"=w1247) -> ("error out"=w1250:errorcluster, "recordset reference"=w1249:T34)  [unwired: 1 in, 4 out]
              n751 = call-poly <vilib>:"DB Tools Free Object.vi"("error in (no error)"=w1250, "recordset reference"=w1249) -> ("error out"=w1245:errorcluster, "connection reference"=w1246:T33)  [unwired: 8 out]
            }
            n752 = call <vilib>:"DB Tools Close Connection.vi"("error in (no error)"=w1221, "connection reference"=w1223) -> ("error out"=w1222:errorcluster)  [unwired: 5 out]
          }
        }
        n753 = local read "configPath"() -> (w1067:path)
        n754 = case shown="No Error" w1068 {
          selector: w1068 -> [w1284 w1311]
          tunnel: [-1 -1] -> w1070
          tunnel: [Collector_State."POLL" ("progState") Collector_State."POLL" ("progState")] -> w1071
          tunnel: w1069 -> [w1295 _]
          tunnel: w1067 -> [w1279 _]
          tunnel: [w1278 w1309] -> w1065
          tunnel: w1064 -> [w1276 w1308]
          tunnel: [w1274 w1308] -> w1063
          frame No Error {
            w1285 = "Data Base Parameters" ("section")
            n755 = local read "LastShot"() -> (w1296:i32)
            n756 = Array Size(array=w1276) -> (size(s)=w1275:i32)
            n757 = flat-sequence {
              tunnel: w1278 -> [_]
              tunnel: w1273 -> [w1306]
              tunnel: [w1306] -> w1274
              frame #0 {
                w1299 = T14."Disabled and Grayed Out" ("Disabled")
                n758 = property on="saveReq" class="Str"("Visible"=TRUE) -> ()  [unwired: 2 in, 2 out]
                n759 = local write "SampleID"("") -> ()
                n760 = property on="clearShots" class="Bool"("Disabled"=T14."Enabled") -> ()  [unwired: 2 in, 2 out]
                n761 = property on="addShot" class="Bool"("Disabled"=w1299) -> ()  [unwired: 2 in, 2 out]
                n762 = property on="undoLastShot" class="Bool"("Disabled"=w1299) -> ()  [unwired: 2 in, 2 out]
                n763 = property on="saveShots" class="Bool"("Disabled"=w1299) -> ()  [unwired: 2 in, 2 out]
                n764 = One Button Dialog(message="Data Saved. Enter new Sample ID.") -> ()  [unwired: 1 in, 1 out]
                n765 = property on="mainTabCntrl" class="TabCtl (strict)"("Value"=enum32{"Setup", "Measure", "History", "System"}."Setup" ("mainTabCntrl")) -> ()  [unwired: 2 in, 2 out]
                n766 = property on="SampleEntryTabCntrl" class="TabCtl (strict)"("Value"=enum32{"Environment", "Sample"}."Sample" ("SampleEntryTabCntrl")) -> ()  [unwired: 2 in, 2 out]
                n767 = property on="Sample SubTabCntrl" class="TabCtl (strict)"("Value"=T2."General Specification" ("Sample SubTabCntrl")) -> ()  [unwired: 2 in, 2 out]
              }
            }
            n768 = Increment(x=w1296) -> (x+1=w1290:i32)
            n769 = call <vilib>:"Open Config Data (compatibility).vi"("error in (no error)"=w1284, "configuration file path"=w1279) -> ("error out"=w1289:errorcluster, "refnum"=w1288:T35)  [unwired: 7 in, 1 out]
            n770 = Add(x=w1290, y=w1295) -> (x+y=w1291:i32)
            n771 = local read "LastSample"() -> (w1292:i32)
            n772 = for {
              N: w1275 -> [_]
              shift-right: [w1297] -> w1273
              shift-left: w1276 -> [w1298]
              n773 = Delete From Array(array=w1298) -> (array with subset deleted=w1297:T7[])  [unwired: 2 in, 1 out]
            }
            n774 = local write "LastShot"(w1291) -> ()
            n775 = call-poly <vilib>:"Write Key.vi"("section"=w1285, "error in (no error)"=w1289, "value"=w1291, "key"="Last Shot Saved ", "refnum"=w1288) -> ("error out"=w1287:errorcluster, "refnum out"=w1286:T35)  [unwired: 5 out]
            n776 = Increment(x=w1292) -> (x+1=w1280:i32)
            n777 = local write "LastSample"(w1280) -> ()
            n778 = call-poly <vilib>:"Write Key.vi"("section"=w1285, "error in (no error)"=w1287, "value"=w1280, "key"="Last Panel Saved ", "refnum"=w1286) -> ("error out"=w1277:errorcluster)  [unwired: 6 out]
            n779 = To Double Precision Float(number=w1280) -> (double precision float=w1283:dbl)
            n780 = call <vilib>:"Close Config Data.vi"("error in (no error)"=w1277, "refnum"=w1286) -> ("error out"=w1278:errorcluster)  [unwired: 1 in, 8 out]
            n781 = property on="Record #" class="DigNum (strict)"("Maximum"=w1283) -> ()  [unwired: 2 in, 2 out]
            n782 = property on="SHOTS" class="Arr (strict)"("Val(Sgnl)"=w1273) -> ()  [unwired: 2 in, 2 out]
          }
          frame Error {
            n783 = One Button Dialog(message="Error saving Data. ") -> ()  [unwired: 2 out]
            n784 = call <vilib>:"General Error Handler.vi"("error in (no error)"=w1311) -> ("error out"=w1309:errorcluster)  [unwired: 2 in, 12 out]
          }
        }
      }
      frame 5 {
        # "Shot Order"
        # "This section accepts new data to the shot table."
        n785 = property on="undoLastShot" class="Bool"(error in=w1321, "Disabled"=u8 0) -> (error out=w1320:errorcluster)  [unwired: 1 in, 1 out]
        n786 = local read "residual/speed"() -> (w1347:sgl)
        n787 = local read "Impact/speed"() -> (w1351:sgl)
        n788 = Array Size(array=w1327) -> (size(s)=w1332:i32)
        n789 = Increment(x=w1332) -> (x+1=w1352:i32)
        n790 = case shown="\"grains\"" "loadingUnits" {
          tunnel: [w1359 w1360] -> w1316
          tunnel: "Powder Loading" -> [w1359 w1361]
          frame "grams", Default {
            # "Always save in grams."
          }
          frame "grains" {
            # "Always save in grams."
            n791 = Multiply(x=w1361, y=sgl 0.06479891) -> (x*y=w1360:sgl)
          }
        }
        n792 = local read "Current/residual/speed"() -> (w1335:sgl)
        n793 = local read "CorrectedVelScrnSet2"() -> (w1356:sgl)
        n794 = local read "MeasVelScrnSet2"() -> (w1353:sgl)
        n795 = local read "CorrectedVelScrnSet1"() -> (w1336:sgl)
        n796 = local read "MeasVelScrnSet1"() -> (w1354:sgl)
        n797 = local read "Current/avg/speed"() -> (w1358:sgl)
        n798 = local read "Corrected Residual"() -> (w1334:sgl)
        n799 = local read "BACKFACE DEPTH"() -> (w1338:sgl)
        n800 = local read "Redundant/speed"() -> (w1355:sgl)
        n801 = local read "conversion factor"() -> (w1345:sgl)
        n802 = local read "Projectile Mass"() -> (w1324:sgl)
        n803 = local read "SHOT STATUS"() -> (w1331:u16)
        n804 = local read "Avg/speed"() -> (w1357:sgl)
        n805 = Multiply(x=w1351, y=w1345) -> (x*y=w1343:sgl)
        n806 = Multiply(x=w1345, y=w1347) -> (x*y=w1344:sgl)
        n807 = Multiply(x=w1343, y=w1343) -> (x*y=w1339:sgl)
        n808 = Multiply(x=w1344, y=w1344) -> (x*y=w1340:sgl)
        n809 = Subtract(x=w1339, y=w1340) -> (x-y=w1341:sgl)
        n810 = Format Date/Time String(time format string (%c)="%x   %H:%M:%S") -> (date/time string=w1348:string)  [unwired: 2 out]
        "SUBMIT DATE/TIME" <- w1348
        n811 = Compound Arithmetic op=MULTIPLY(w1324, w1341, sgl 0.0005 ("Input")) -> (w1346:sgl)
        n812 = Index Array(array=w1327) -> (element=w1330:T7)  [unwired: 1 in]
        n813 = Bundle By Name(cluster=w1330, "TIME / DATE"=w1348, "shot order"=w1352, "IMPACT VELOCITY"=w1351, "RESIDUAL  VELOCITY"=w1347, "Shot Description"="Shot Description", "Powder Loading"=w1316, "Barrel Temperature"="Barrel Temp", "SHOT STATUS"=w1331, "BackFace\nDepth"=w1338, "Shot Angle"="Shot Angle", "Uncorrected Impact"=w1354, "Corrected Impact"=w1336, "Uncorrected Residual"=w1335, "Corrected residual"=w1334, "Projectile Mass"=w1324, "Energy Loss (J)"=w1346, "UncorrectedRed_PB"=w1353, "Redundant_Velocity"=w1355, "CorrectedRed_PB"=w1356, "UncorrectedAvgVel_PB"=w1358, "avgVel_PB"=w1357, "Frag Rod"="Frag Rod", "V50userExcl"=FALSE) -> (w1333:T7)
        n814 = Build Array (concatenate)(w1327, w1333) -> (w1323:T7[])
        n815 = stacked-sequence {
          tunnel: w1323 -> [w1366]
          tunnel: [w1366] -> w1322
          tunnel: w1320 -> [w1365]
          tunnel: [w1364] -> w1319
          frame #0 {
            n816 = property on="shotsTabCntrl" class="TabCtl (strict)"(error in=w1365, "Value"=T5."Shots Table" ("shotsTabCntrl")) -> (error out=w1364:errorcluster)  [unwired: 1 in, 1 out]
            n817 = local write "backdepth"(sgl 0.0 ("BACKFACE DEPTH")) -> ()
          }
        }
      }
      frame 6 {
        # "This section will clear the shot table and re-enable the \"ADD SHOT\" button to get ready for a new test panel."
        n818 = Two Button Dialog(message="Shot table cleared even if not saved. Are you sure?", 1:"NO" ("F button name (\"Cancel\")"), 2:"YES" ("T button name (\"OK\")")) -> (T button?=w1371:bool)
        n819 = case shown="True" w1371 {
          tunnel: [w1377 T7[] [] ("SHOTS")] -> w1376
          tunnel: w1372 -> [w1377 _]
          frame False {
          }
          frame True {
            w1378 = T14."Disabled and Grayed Out" ("Disabled")
            n820 = invoke on="Table of Shots" class="Tbl (strict)" method="Reinit To Default"() -> ()  [unwired: 3 in, 3 out]
            n821 = invoke on="SHOTS" class="Arr (strict)" method="Reinit To Default"() -> ()  [unwired: 3 in, 3 out]
            n822 = property on="addShot" class="Bool"("Disabled"=T14."Enabled") -> ()  [unwired: 2 in, 2 out]
            n823 = property on="clearShots" class="Bool"("Disabled"=w1378) -> ()  [unwired: 2 in, 2 out]
            n824 = property on="undoLastShot" class="Bool"("Disabled"=w1378) -> ()  [unwired: 2 in, 2 out]
            n825 = property on="saveShots" class="Bool"("Disabled"=w1378) -> ()  [unwired: 2 in, 2 out]
            n826 = property on="saveReq" class="Str"("Visible"=TRUE) -> ()  [unwired: 2 in, 2 out]
          }
        }
      }
      frame 7 {
        n827 = property on="SHOTS" class="Arr (strict)"(error in=w1384) -> (error out=w1383:errorcluster, "Index Values"=w1388:u32[])  [unwired: 1 in, 1 out]
        n828 = Array Size(array=w1395) -> (size(s)=w1391:i32)
        n829 = Index Array "Index Array"(array=w1388) -> (element=w1393:u32)  [unwired: 1 in]
        n830 = To Unsigned Long Integer(number=w1391) -> (unsigned 32bit integer=w1387:u32)
        n831 = Increment(x=w1393) -> (x+1=w1392:u32)
        n832 = Quotient & Remainder(x=w1392, y=w1387) -> (x-y*floor(x/y)=w1390:u32)  [unwired: 1 out]
        n833 = Replace Array Subset "Replace Array Subset"(array=w1388, new element=w1390) -> (w1389:u32[])  [unwired: 1 in]
        n834 = property on="SHOTS" class="Arr (strict)"(error in=w1383, "Index Values"=w1389) -> (error out=w1382:errorcluster, "Value"=w1394:T7[])  [unwired: 1 in, 1 out]
      }
      frame 8 {
        # "This section undoes new shot data OR deletes the currently accessed previous shot"
        n835 = local read "deleteShot"() -> (w1402:bool)
        n836 = case shown="True" w1402 {
          tunnel: w1401 -> [w1405 w1418]
          tunnel: [w1406 w1419] -> w1400
          frame False {
            n837 = Array Size(array=w1405) -> (size(s)=w1403:i32)
            n838 = while {
              tunnel: [w1409] -> w1404
              tunnel: w1403 -> [w1411]
              tunnel: w1405 -> [w1413] mode=indexing
              i -> [w1409]
              stop <- w1412 stop-if-true
              n839 = Unbundle By Name(w1413) -> ("shot order"=w1410:i32)
              n840 = Equal?(x=w1410, y=w1411) -> (x = y?=w1412:bool)
            }
            n841 = Delete From Array "Delete From Array"(array=w1405, index=w1404) -> (array with subset deleted=w1406:T7[])  [unwired: 1 in, 1 out]
            n842 = local write "SUBMIT DATE/TIME"("" ("Empty String Constant")) -> ()
            n843 = property on="undoLastShot" class="Bool"("Disabled"=u8 2) -> ()  [unwired: 2 in, 2 out]
          }
          frame True {
            n844 = property on="SHOTS" class="Arr (strict)"() -> ("Index Values"=w1427:u32[])  [unwired: 2 in, 2 out]
            n845 = local write "deleteShot"(FALSE) -> ()
            n846 = Index Array(array=w1427, index=0 ("Index")) -> (element=w1417:u32)
            n847 = To Long Integer(number=w1417) -> (32bit integer=w1414:i32)
            n848 = Index Array(array=w1418, index=w1414) -> (element=w1416:T7)
            n849 = Unbundle By Name(w1416) -> ("shot order"=w1415:i32)
            n850 = Format Into String(format string="The currently displayed Shot, #%d", w1415) -> (resulting string=w1424:string)  [unwired: 2 in, 1 out]
            n851 = Concatenate Strings(w1424, ", will be deleted.  IT CANNOT RECOVERED!  Do you want to DELETE the shot?" ("message")) -> (w1423:string)
            n852 = Two Button Dialog(message=w1423, 1:"NO I do NOT want to delete.  Cancel Request" ("F button name (\"Cancel\")"), 2:"YES I want to delete the shot" ("T button name (\"OK\")")) -> (T button?=w1430:bool)
            n853 = case shown="True" w1430 {
              tunnel: w1418 -> [w1443 w1446]
              tunnel: [w1443 w1448] -> w1421
              tunnel: w1414 -> [_ w1445]
              tunnel: [10000 ("shot order") w1447] -> w1420
              frame False {
              }
              frame True {
                n854 = Index Array(array=w1446, index=w1445) -> (element=w1444:T7)
                n855 = Unbundle By Name(w1444) -> ("shot order"=w1447:i32)
                n856 = Delete From Array(array=w1446, index=w1445) -> (array with subset deleted=w1448:T7[])  [unwired: 1 in, 1 out]
              }
            }
            n857 = for {
              tunnel: [w1437] -> w1419 mode=indexing
              tunnel: w1421 -> [w1432] mode=indexing
              tunnel: w1420 -> [w1436]
              n858 = Unbundle By Name(w1432) -> ("shot order"=w1434:i32)
              n859 = Decrement(x=w1434) -> (x-1=w1433:i32)
              n860 = Greater?(x=w1434, y=w1436) -> (0:w1435:bool)
              n861 = case shown="True" w1435 {
                tunnel: w1433 -> [_ w1440]
                tunnel: w1432 -> [w1438 w1441]
                tunnel: [w1438 w1439] -> w1437
                frame False {
                }
                frame True {
                  n862 = Bundle By Name(cluster=w1441, "shot order"=w1440) -> (w1439:T7)
                }
              }
            }
          }
        }
        n863 = property on="SHOTS" class="Arr (strict)"(error in=w1396, "Val(Sgnl)"=w1400) -> (error out=w1397:errorcluster)  [unwired: 1 in, 1 out]
      }
      frame 9 {
        n864 = local write "SUBMIT DATE/TIME"("" ("Empty String Constant")) -> ()
        n865 = Concatenate Strings("L|", "6|") -> (w1455:string)
        n866 = case shown="\"Simulated\", Default" "MeasSrc" {
          tunnel: w1455 -> [_ _ w1471]
          tunnel: w1450 -> [w1461 w1466 w1470]
          tunnel: [w1459 w1466 w1467] -> w1449
          frame "Simulated", Default {
            n867 = flat-sequence {
              tunnel: w1461 -> [w1462]
              tunnel: [w1462] -> w1460
              tunnel: [w1464] -> w1459
              tunnel: w1460 -> [w1464]
              frame #0 {
                n868 = local write "readyClock"(FALSE ("RANGE RESET")) -> ()
              }
              frame #1 {
                n869 = Wait (ms)(milliseconds to wait=u32 100) -> ()  [unwired: 1 out]
              }
            }
          }
          frame "Radar" {
          }
          frame "Screens" {
            w1477 = u32 22 items=["NI-DAQ version", "device name", "base address", "data transfer mode for analog input", "data transfer mode for analog output group 1", "data transfer mode for analog output group 2", "data transfer mode for GPCTR 0", "data transfer mode for GPCTR 1", "data transfer mode for digital I/O group 1", "data transfer mode for digital I/O group 2", "device type code", "DMA A level", "DMA B level", "DMA C level", "interrupt A level", "interrupt B level", "reserved", "lpt device mode", "DAQCard-700 counter 1 source", "interrupt generation mode", "device state during suspend mode", "computer name", "serial number", "counter type", "Scarab A Memory Size", "Scarab B Memory Size"] ("information type")
            w1476 = u32 1  # device
            n870 = Concatenate Strings(w1471, "2|") -> (w1472:string)
            n871 = call <vilib>:"Get DAQ Device Information.vi"("error in (no error)"=w1470, "information type"=w1477, "task ID or device"=w1476) -> ("error out"=w1469:errorcluster, "information string"=w1475:string)  [unwired: 7 out]
            n872 = disable-structure "Diagram Disable Structure" shown="Enabled" {
              disable-tunnel: w1472 -> [w1482 _]
              disable-tunnel: w1469 -> [w1479 w1484]
              disable-tunnel: [w1478 w1484] -> w1468
              frame Disabled {
                n873 = Current VI's Path() -> (path=w1483:path)
                n874 = call "Where Am I (SubVI).vi"("TL Calling Location"=w1482, "Call VI path"=w1483) -> ("I'm here"=w1481:string)
                n875 = call "Error Check (SubVI).vi"("calling VI"=w1481, "tag #"=0, "error IN"=w1479) -> ("error OUT"=w1478:errorcluster)  [unwired: 2 in]
              }
              frame Enabled {
                # "Debug code is disabled"
              }
            }
            n876 = case shown="Error" w1468 {
              selector: w1468 -> [w1485 _]
              tunnel: w1475 -> [w1495 _]
              tunnel: [w1495 "DEVICE NOT READY!" ("information string")] -> w1474
              tunnel: [w1486 errorcluster {"status"=FALSE, "code"=0, "source"=""} ("error out")] -> w1467
              frame No Error {
                # "assign task IDs to counters"
                n877 = call "Config Counter to Measure Two Edge Separation.vi"("error IN"=w1485, "Counter"="Impact Timer", "device"="DAQ Card") -> ("error out"=w1497:errorcluster, "task ID out"=w1491:u32)  [unwired: 1 in]
                "impact/ID" <- w1491
                n878 = local write "readyClock"(FALSE ("RANGE RESET")) -> ()
                n879 = call "Config Counter to Measure Two Edge Separation.vi"("error IN"=w1497, "Counter"="Residual  Timer", "device"="DAQ Card") -> ("error out"=w1499:errorcluster, "task ID out"=w1489:u32)  [unwired: 1 in]
                "residual/ID" <- w1489
                n880 = call "Config Counter to Measure Two Edge Separation.vi"("error IN"=w1499, "Counter"="Redundant Timer", "device"="DAQ Card") -> ("error out"=w1498:errorcluster, "task ID out"=w1490:u32)  [unwired: 1 in]
                "Red/ID" <- w1490
                n881 = Bundle("task ID out"=w1491, "task ID out"=w1490, "task ID out"=w1489) -> (w1487:T36)  [unwired: 1 out]
                n882 = call <vilib>:"Simple Error Handler.vi"("error in (no error)"=w1498) -> ("error out"=w1486:errorcluster)  [unwired: 1 in, 7 out]
                n883 = global write "BIMS_Collector Globals.vi" "Screens"(w1487) -> ()
              }
              frame Error {
                n884 = One Button Dialog(message="Error initializing Timer board.  Switching to simulation") -> ()  [unwired: 2 out]
                n885 = local write "MeasSrc"(DataSource."Simulated" ("MeasSrc")) -> ()
              }
            }
            "Device S/N" <- w1474
          }
        }
      }
      frame 9 {
        n886 = local write "processShots"(FALSE ("ProcessShots")) -> ()
        n887 = local read "Drag Corrected"() -> (w1509:bool)
        n888 = stacked-sequence {
          seq-local: [_ w1567 _ _] -> [_ _ w1596 w1646]
          seq-local: [w1531 _ _ _] -> [_ w1563 _ _]
          seq-local: [w1529 _ _ _] -> [_ w1564 _ _]
          seq-local: [w1530 _ _ _] -> [_ w1565 _ _]
          tunnel: [_ _ _ w1640] -> w1510
          tunnel: w1509 -> [w1533 w1566 _ _]
          tunnel: w1506 -> [_ w1562 _ _]
          tunnel: w1505 -> [w1528 _ _ _]
          tunnel: [w1528 _ _ _] -> w1504
          frame #0 {
            n889 = disable-structure "Diagram Disable Structure" shown="Enabled" {
              disable-tunnel: [w1550 w1557] -> w1538
              frame Disabled {
                n890 = local read "factor array"() -> (w1552:sgl[])
                n891 = local read "Threat"() -> (w1549:u16)
                n892 = To Long Integer(number=w1549) -> (32bit integer=w1551:i32)
                n893 = Index Array(array=w1552, index=w1551) -> (element=w1550:sgl)
              }
              frame Enabled {
                n894 = local read "threatDetails"() -> (w1556:T1)
                n895 = Unbundle By Name(w1556) -> ("dragCorrection"=w1554:string)
                n896 = Not Equal?(x=w1554, y="") -> (x != y?=w1555:bool)
                n897 = case shown="True" w1555 {
                  tunnel: [sgl 1.0 ("default value 1") w1560] -> w1557
                  tunnel: w1554 -> [_ w1559]
                  frame False {
                  }
                  frame True {
                    n898 = Scan From String(input string=w1559, default 1=sgl 0.0 ("default value 1")) -> (output 1=w1560:sgl)  [unwired: 3 in, 3 out]
                  }
                }
              }
            }
            "correction coefficient" <- w1538
            n899 = local read "Current/avg/speed"() -> (w1534:sgl)
            n900 = local read "mid_to_targ_dist"() -> (w1535:sgl)
            n901 = local read "lengthUnits"() -> (w1532:string)
            n902 = call "Compute Strike Velocity.vi"("drag coefficient"=w1538, "decay distance"=w1535, "raw velocity"=w1534, "distance units"=w1532) -> ("correction factor"=w1531:sgl, "strike velocity"=w1536:sgl)  [unwired: 1 out]
            "DC_ factor" <- w1531
            "Corrected Average" <- w1536
            n903 = call "Velocity Correction.vi"("raw impact"="MeasVelScrnSet1", "distance units"=w1532, "raw redundant"="MeasVelScrnSet2", "raw residual"="Current/residual/speed", "screen set midpt to target"="Set#1_to_Target", "residual screen to target"="Residual/Target Dist", "correction coefficient"=w1538) -> ("corrected impact"=w1543:sgl, "corrected redundant"=w1539:sgl, "corrected residual"=w1541:sgl, "impact factor"=w1529:sgl, "conversion factor"=→"conversion factor":sgl, "residual factor"=w1530:sgl)  [unwired: 3 out]
            "Residual factor" <- w1530
            "Impact factor" <- w1529
            "CorrectedVelScrnSet1" <- w1543
            "Corrected Residual" <- w1541
            "CorrectedVelScrnSet2" <- w1539
            n904 = Select(t=w1539, s=w1533, f="MeasVelScrnSet2") -> (s? t:f=→"Redundant/speed":sgl)
            n905 = Select(t=w1536, s=w1533, f=w1534) -> (s? t:f=→"Avg/speed":sgl)
            n906 = Select(t=w1543, s=w1533, f="MeasVelScrnSet1") -> (s? t:f=→"Impact/speed":sgl)
            n907 = Select(t=w1541, s=w1533, f="Current/residual/speed") -> (s? t:f=→"residual/speed":sgl)
            n908 = Add(x="MeasVelScrnSet2", y="MeasVelScrnSet1") -> (x+y=w1515:sgl)
            n909 = Subtract(x="MeasVelScrnSet2", y="MeasVelScrnSet1") -> (x-y=w1514:sgl)
            n910 = Divide(x=w1515, y=sgl 200.0) -> (x/y=w1516:sgl)
            n911 = Divide(x=w1514, y=w1516) -> (x/y=w1520:sgl)
            "%_Difference" <- w1520
            n912 = Absolute Value(x=w1520) -> (abs(x)=w1522:sgl)
            n913 = Less?(x=w1522, y="percent warning") -> (x < y?=w1527:bool)
            n914 = Select(t=u32 65343, s=w1527, f=u32 15668992) -> (s? t:f=w1523:u32)
            n915 = Select(t=u32 0, s=w1527, f=u32 16777226) -> (s? t:f=w1526:u32)
            n916 = property on="%_Difference" class="DigNum (strict)"("Numeric Text.Text Colors:BG Color"=w1523, "NumText.TextColor"=w1526) -> ()  [unwired: 2 in, 2 out]
          }
          frame #1 {
            # "<-- DC_factor (for Average of impact and redundant)"
            # "IF drag corrected THEN apply factors"
            # "Residual factor"
            # "Impact factor\n(also applies to\nredundant velocity)"
            n917 = for {
              tunnel: w1562 -> [w1575] mode=indexing
              tunnel: w1565 -> [w1584]
              tunnel: w1564 -> [w1579]
              tunnel: w1566 -> [w1573]
              tunnel: [w1586] -> w1567 mode=indexing
              tunnel: w1563 -> [w1568]
              n918 = Unbundle By Name(w1575) -> ("UncorrectedAvgVel_PB"=w1574:sgl)
              n919 = Unbundle By Name(w1575) -> ("Uncorrected Impact"=w1578:sgl)
              n920 = Unbundle By Name(w1575) -> ("Uncorrected Residual"=w1583:sgl)
              n921 = Unbundle By Name(w1575) -> ("UncorrectedRed_PB"=w1581:sgl)
              n922 = Multiply(x=w1568, y=w1574) -> (x*y=w1571:sgl)
              n923 = Multiply(x=w1579, y=w1581) -> (x*y=w1580:sgl)
              n924 = Multiply(x=w1579, y=w1578) -> (x*y=w1569:sgl)
              n925 = Multiply(x=w1584, y=w1583) -> (x*y=w1576:sgl)
              n926 = Select(t=w1571, s=w1573, f=w1574) -> (s? t:f=w1572:sgl)
              n927 = Select(t=w1580, s=w1573, f=w1581) -> (s? t:f=w1582:sgl)
              n928 = Select(t=w1576, s=w1573, f=w1583) -> (s? t:f=w1585:sgl)
              n929 = Select(t=w1569, s=w1573, f=w1578) -> (s? t:f=w1577:sgl)
              n930 = Subtract(x=w1572, y=w1571) -> (x-y=w1570:sgl)
              n931 = Bundle By Name(cluster=w1575, "velLoss_PB"=w1570, "strikeVel_PB"=w1571, "avgVel_PB"=w1572, "CorrectedRed_PB"=w1580, "Redundant_Velocity"=w1582, "Corrected Impact"=w1569, "IMPACT VELOCITY"=w1577, "Corrected residual"=w1576, "RESIDUAL  VELOCITY"=w1585) -> (w1586:T7)
            }
          }
          frame #2 {
            w1597 = sgl[] [] ("Partial")
            # "This section calculates the V50"
            n932 = for {
              shift-right: [w1621] -> w1599
              shift-left: w1597 -> [w1622]
              shift-right: [w1619] -> w1598
              shift-left: w1597 -> [w1620]
              tunnel: w1596 -> [w1613] mode=indexing
              n933 = Unbundle By Name(w1613) -> ("SHOT STATUS"=w1618:u16)
              n934 = Unbundle By Name(w1613) -> ("V50userExcl"=w1612:bool)
              n935 = Unbundle By Name(w1613) -> ("IMPACT VELOCITY"=w1617:sgl)
              n936 = Unbundle By Name(w1613) -> ("strikeVel_PB"=w1616:sgl)
              n937 = Select(t=w1616, s="ScreenSetAvgg", f=w1617) -> (s? t:f=w1615:sgl)
              n938 = case shown="False" w1612 {
                tunnel: w1622 -> [w1628 w1638]
                tunnel: [w1627 w1638] -> w1621
                tunnel: w1620 -> [w1626 w1637]
                tunnel: [w1625 w1637] -> w1619
                tunnel: w1618 -> [w1624 _]
                tunnel: w1615 -> [w1623 _]
                frame False {
                  n939 = case shown="1" w1624 {
                    tunnel: w1623 -> [w1629 w1633]
                    tunnel: [w1632 w1634] -> w1627
                    tunnel: w1628 -> [w1631 w1634]
                    tunnel: w1626 -> [w1630 w1636]
                    tunnel: [w1630 w1635] -> w1625
                    frame 0, Default {
                      n940 = Build Array (concatenate)(w1631, w1629) -> (w1632:sgl[])
                    }
                    frame 1 {
                      n941 = Build Array (concatenate)(w1636, w1633) -> (w1635:sgl[])
                    }
                  }
                }
                frame True {
                }
              }
            }
            n942 = Sort 1D Array(array=w1599) -> (sorted array=w1611:sgl[])
            n943 = Sort 1D Array(array=w1598) -> (sorted array=w1604:sgl[])
            "Complete" <- w1604
            n944 = Reverse 1D Array(array=w1611) -> (reversed array=w1602:sgl[])
            "Partial" <- w1602
            n945 = Array Size(array=w1604) -> (size(s)=→"#_completes":i32)
            n946 = Array Size(array=w1602) -> (size(s)=→"#_partials":i32)
            n947 = Array Max & Min(array=w1602) -> (max value=w1608:sgl)  [unwired: 3 out]
            n948 = Array Max & Min(array=w1604) -> (min value=w1606:sgl)  [unwired: 3 out]
            n949 = call "Compute V50.vi"("Partial"=w1602, "Maximum Deviation"="maxDev", "Complete"=w1604) -> ("Pairs"=→"Pairs":i16, "zmr"=w1587:sgl, "V50"=→"computed_V50":sgl)  [unwired: 2 out]
            "Z.M.R." <- w1587
            n950 = To Long Integer(number=w1608) -> (32bit integer=→"highPartial":i32)
            n951 = To Long Integer(number=w1606) -> (32bit integer=→"lowComplete":i32)
            n952 = Absolute Value(x=w1587) -> (abs(x)=→"zmr 2":sgl)
            n953 = Less Than 0?(x=w1587) -> (x < 0?=w1590:bool)
            n954 = Select(t="Low C minus High P", s=w1590, f="ZMR") -> (s? t:f=w1593:string)
            n955 = Select(t=u32 65336, s=w1590, f=u32 16755266) -> (s? t:f=w1594:u32)
            n956 = property on="zmr 2" class="DigNum (strict)"("Caption.Text"=w1593, "Numeric Text.Text Colors:BG Color"=w1594) -> ()  [unwired: 2 in, 2 out]
          }
          frame #3 {
            n957 = local read "Pairs"() -> (w1651:i16)
            n958 = Sort 1D Array(array=w1646) -> (sorted array=w1649:T7[])
            n959 = for {
              tunnel: w1649 -> [w1695] mode=indexing
              tunnel: w1651 -> [w1705]
              shift-right: [w1704] -> _
              shift-left: i16 0 -> [w1703]
              tunnel: [w1697] -> w1647 mode=indexing
              # "this section marks the lowest completes that are used in V50"
              n960 = Unbundle By Name(w1695) -> ("SHOT STATUS"=w1701:u16, "Projectile Mass"=w1699:sgl, "avgVel_PB"=w1698:sgl, "RESIDUAL  VELOCITY"=w1700:sgl)
              n961 = Unbundle By Name(w1695) -> ("V50userExcl"=w1696:bool)
              n962 = local read "conversion factor"() -> (w1707:sgl)
              n963 = case shown="False" w1696 {
                tunnel: w1705 -> [w1718 _]
                tunnel: [w1717 w1727] -> w1704
                tunnel: w1703 -> [w1716 w1727]
                tunnel: [w1715 FALSE] -> w1702
                tunnel: w1701 -> [w1714 _]
                frame False {
                  n964 = case shown="1" w1714 {
                    tunnel: w1718 -> [_ w1725]
                    tunnel: [FALSE w1724] -> w1715
                    tunnel: [w1720 w1723] -> w1717
                    tunnel: w1716 -> [w1720 w1721]
                    frame 0, Default {
                    }
                    frame 1 {
                      n965 = Less?(x=w1721, y=w1725) -> (x < y?=w1724:bool)
                      n966 = Add(x=w1721, y=i16 1 ("t")) -> (x+y=w1723:i16)
                    }
                  }
                }
                frame True {
                }
              }
              n967 = Multiply(x=w1707, y=w1700) -> (x*y=w1708:sgl)
              n968 = Multiply(x=w1698, y=w1707) -> (x*y=w1709:sgl)
              n969 = Multiply(x=w1709, y=w1709) -> (x*y=w1713:sgl)
              n970 = Multiply(x=w1708, y=w1708) -> (x*y=w1712:sgl)
              n971 = Subtract(x=w1713, y=w1712) -> (x-y=w1711:sgl)
              n972 = Compound Arithmetic op=MULTIPLY(w1699, w1711, sgl 0.0005 ("Input")) -> (w1706:sgl)
              n973 = Bundle By Name(cluster=w1695, "usedv50"=w1702, "Energy Loss (J)"=w1706) -> (w1697:T7)
            }
            n974 = Reverse 1D Array(array=w1647) -> (reversed array=w1648:T7[])
            n975 = for {
              tunnel: w1648 -> [w1671] mode=indexing
              tunnel: w1651 -> [w1678]
              shift-right: [w1676] -> _
              shift-left: i16 0 -> [w1677]
              tunnel: [w1674] -> w1640 mode=indexing
              # "chooses highest partials used in v50"
              n976 = Unbundle By Name(w1671) -> ("SHOT STATUS"=w1679:u16, "usedv50"=w1673:bool)
              n977 = Unbundle By Name(w1671) -> ("V50userExcl"=w1672:bool)
              n978 = case shown="True" w1672 {
                tunnel: w1679 -> [w1685 _]
                tunnel: w1678 -> [w1684 _]
                tunnel: w1677 -> [w1683 w1694]
                tunnel: [w1682 w1694] -> w1676
                tunnel: [w1681 FALSE ("usedv50")] -> w1675
                tunnel: w1673 -> [w1680 _]
                frame False {
                  n979 = case shown="1" w1685 {
                    tunnel: w1684 -> [w1689 _]
                    tunnel: [w1688 w1692] -> w1681
                    tunnel: w1683 -> [w1686 w1691]
                    tunnel: [w1687 w1691] -> w1682
                    tunnel: w1680 -> [_ w1692]
                    frame 0, Default {
                      n980 = Less?(x=w1686, y=w1689) -> (x < y?=w1688:bool)
                      n981 = Add(x=w1686, y=i16 1) -> (x+y=w1687:i16)
                    }
                    frame 1 {
                    }
                  }
                }
                frame True {
                }
              }
              n982 = Bundle By Name(cluster=w1671, "usedv50"=w1675) -> (w1674:T7)
            }
            n983 = for {
              shift-right: [w1657] -> w1639
              shift-left: sgl[] [] ("Partial") -> [w1654]
              tunnel: w1640 -> [w1656] mode=indexing
              n984 = local read "ScreenSetAvgg"() -> (w1661:bool)
              n985 = Unbundle By Name(w1656) -> ("IMPACT VELOCITY"=w1659:sgl)
              n986 = Unbundle By Name(w1656) -> ("V50userExcl"=w1655:bool, "usedv50"=w1653:bool)
              n987 = Unbundle By Name(w1656) -> ("strikeVel_PB"=w1660:sgl)
              n988 = Select(t=w1660, s=w1661, f=w1659) -> (s? t:f=w1658:sgl)
              n989 = case shown="False" w1655 {
                tunnel: w1658 -> [w1662 _]
                tunnel: [w1663 w1670] -> w1657
                tunnel: w1654 -> [w1664 w1670]
                tunnel: w1653 -> [w1665 _]
                frame False {
                  n990 = case shown="True" w1665 {
                    tunnel: w1664 -> [w1666 w1669]
                    tunnel: [w1666 w1668] -> w1663
                    tunnel: w1662 -> [_ w1667]
                    frame False {
                    }
                    frame True {
                      n991 = Build Array (concatenate)(w1669, w1667) -> (w1668:sgl[])
                    }
                  }
                }
                frame True {
                }
              }
            }
            n992 = Array Max & Min(array=w1639) -> (max value=w1645:sgl, min value=w1644:sgl)  [unwired: 2 out]
            n993 = property on="SHOTS" class="Arr (strict)"("Val(Sgnl)"=w1640) -> ()  [unwired: 2 in, 2 out]
            n994 = Subtract(x=w1645, y=w1644) -> (x-y=w1643:sgl)
            n995 = To Long Integer(number=w1643) -> (32bit integer=→"rangeOfResults":i32)
          }
        }
      }
      frame 11 {
        n996 = local read "SafetyInterlock"() -> (w1736:cluster{"ARMED":bool})
        n997 = Unbundle By Name(w1736) -> ("ARMED"=w1735:bool)
        n998 = Not(x="InterlockExists") -> (.not. x?=w1731:bool)
        n999 = Or(x=w1735, y=w1731) -> (x .or. y?=w1732:bool)
        n1000 = case shown="True" w1732 {
          tunnel: [Collector_State."POLL" ("progState") w1745] -> w1734
          tunnel: [-1 ("index of element") w1744] -> w1733
          tunnel: "InterlockExists" -> [_ w1743]
          tunnel: [w1738 w1742] -> w1729
          tunnel: w1728 -> [w1738 w1741]
          frame False {
          }
          frame True {
            n1001 = stacked-sequence {
              tunnel: [_ Collector_State."PROCESS SHOTS" ("progState")] -> w1745
              tunnel: [_ -1] -> w1744
              tunnel: w1743 -> [w1748 _]
              tunnel: [w1746 _] -> w1742
              tunnel: w1741 -> [w1747 _]
              frame #0 {
                n1002 = local read "MeasSrc"() -> (w1750:T6)
                n1003 = case shown="\"Simulated\", Default" w1750 {
                  tunnel: [w1753 w1777 w1788] -> w1749
                  tunnel: w1748 -> [_ _ w1786]
                  tunnel: w1747 -> [w1751 w1776 w1784]
                  tunnel: [w1751 w1776 w1785] -> w1746
                  frame "Simulated", Default {
                    # "Simulated"
                    n1004 = local read "minV50"() -> (w1759:i32)
                    n1005 = local read "Powder Loading"() -> (w1775:sgl)
                    n1006 = To Single Precision Float(number=w1759) -> (single precision float=w1758:sgl)
                    n1007 = call "Get Shell Speed.vi"("loading"=w1775, "v50"=w1758) -> ("impact"=w1763:sgl, "residual"=w1770:sgl)  [unwired: 1 in, 2 out]
                    n1008 = Random Number (0-1)() -> (number: 0 to 1=w1768:dbl)
                    n1009 = To Single Precision Float(number=w1768) -> (single precision float=w1764:sgl)
                    n1010 = Multiply(x=w1764, y=sgl 0.002) -> (x*y=w1767:sgl)
                    n1011 = local read "SafetyInterlock"() -> (w1754:cluster{"ARMED":bool})
                    n1012 = Add(x=w1767, y=sgl 0.999) -> (x+y=w1765:sgl)
                    n1013 = Greater Than 0?(x=w1770) -> (x > 0?=w1772:bool)
                    n1014 = Multiply(x=w1763, y=w1765) -> (x*y=w1762:sgl)
                    n1015 = Bundle By Name(cluster=w1754, "ARMED"=FALSE) -> (w1755:cluster{"ARMED":bool})
                    n1016 = Add(x=w1763, y=w1762) -> (x+y=w1760:sgl)
                    n1017 = Select(t=u16 1, s=w1772, f=u16 0) -> (s? t:f=w1771:u16)
                    n1018 = local write "readyClock"(TRUE ("RANGE RESET")) -> ()
                    n1019 = local write "SafetyInterlock"(w1755) -> ()
                    n1020 = Divide(x=w1760, y=sgl 2.0 ("v50")) -> (x/y=w1753:sgl)
                    n1021 = local write "Current/residual/speed"(w1770) -> ()
                    n1022 = local write "SHOT STATUS"(w1771) -> ()
                    n1023 = local write "Current/sthotstatus"(w1771) -> ()
                    n1024 = local write "MeasVelScrnSet1"(w1763) -> ()
                    n1025 = local write "MeasVelScrnSet2"(w1762) -> ()
                    n1026 = Wait (ms)(milliseconds to wait=u32 500 ("number")) -> ()  [unwired: 1 out]
                  }
                  frame "Radar" {
                    # "Radar -- (future)"
                    n1027 = local read "MeasVelScrnSet1"() -> (w1779:sgl)
                    n1028 = local read "MeasVelScrnSet2"() -> (w1778:sgl)
                    n1029 = Add(x=w1779, y=w1778) -> (x+y=w1780:sgl)
                    n1030 = Divide(x=w1780, y=sgl 2.0) -> (x/y=w1777:sgl)
                  }
                  frame "Screens" {
                    # "This section checks to see if the counters have been fired.  If they have then the counter times are read"
                    n1031 = Concatenate Strings("-1|", "F0|") -> (w1789:string)
                    n1032 = case shown="True" w1786 {
                      tunnel: w1784 -> [w1796 w1797]
                      tunnel: [w1796 w1797] -> w1783
                      frame False {
                      }
                      frame True {
                      }
                    }
                    n1033 = global read "BIMS_Collector Globals.vi" "Screens"() -> (w1787)
                    n1034 = Unbundle By Name(w1787) -> ("ScrnSet1CntrID"=w1792)
                    n1035 = Concatenate Strings(w1789, "2|") -> (w1793:string)
                    n1036 = call "Check DAQ Status.vi"("errIN"=w1783, "TL Calling Location"=w1793, "Task ID"=w1792) -> ("error out"=w1795:errorcluster, "Armed?"=w1782:bool)  [unwired: 1 out]
                    n1037 = case shown="False" w1782 {
                      tunnel: w1795 -> [w1825 w1863]
                      tunnel: w1792 -> [w1808 _]
                      tunnel: w1793 -> [w1821 _]
                      tunnel: w1787 -> [w1811 _]
                      tunnel: [w1799 w1864] -> w1788
                      tunnel: [w1798 w1863] -> w1785
                      frame False {
                        n1038 = local read "Set#1 Separation"() -> (w1828:sgl)
                        n1039 = Concatenate Strings(w1821, "F|") -> (w1816:string)
                        n1040 = call "Read TIO Count.vi"("TL Calling Location"=w1816, "error In"=w1825, "task IN"=w1808) -> ("error out"=w1810:errorcluster, "time (secs)"=w1830:sgl)  [unwired: 1 in, 4 out]
                        n1041 = Divide(x=w1828, y=w1830) -> (x/y=w1804:sgl)
                        n1042 = call "Arm TIO Channel.vi"("error IN"=w1810, "task ID IN"=w1808) -> ("error out"=w1809:errorcluster)  [unwired: 1 in, 2 out]
                        n1043 = Unbundle By Name(w1811) -> ("ScrnSet2CntrID"=w1813)
                        n1044 = Concatenate Strings(w1816, "a|") -> (w1819:string)
                        n1045 = call "Check DAQ Status.vi"("errIN"=w1809, "TL Calling Location"=w1819, "Task ID"=w1813) -> ("error out"=w1824:errorcluster, "Armed?"=w1815:bool)  [unwired: 1 out]
                        n1046 = case shown="False" w1815 {
                          tunnel: [w1841 sgl 0.0] -> w1805
                          tunnel: w1824 -> [w1840 w1845]
                          tunnel: [w1835 w1845] -> w1826
                          tunnel: w1813 -> [w1834 _]
                          tunnel: w1816 -> [w1838 _]
                          frame False {
                            n1047 = local read "Set#2 Separation"() -> (w1842:sgl)
                            n1048 = Concatenate Strings(w1838, "Fa|") -> (w1837:string)
                            n1049 = call "Read TIO Count.vi"("TL Calling Location"=w1837, "error In"=w1840, "task IN"=w1834) -> ("error out"=w1836:errorcluster, "time (secs)"=w1843:sgl)  [unwired: 1 in, 4 out]
                            n1050 = Divide(x=w1842, y=w1843) -> (x/y=w1841:sgl)
                            n1051 = call "Arm TIO Channel.vi"("error IN"=w1836, "task ID IN"=w1834) -> ("error out"=w1835:errorcluster)  [unwired: 1 in, 2 out]
                          }
                          frame True {
                          }
                        }
                        n1052 = Unbundle By Name(w1811) -> ("residualCntrID"=w1812)
                        n1053 = Add(x=w1804, y=w1805) -> (x+y=w1806:sgl)
                        n1054 = Concatenate Strings(w1816, "b|") -> (w1817:string)
                        n1055 = call "Check DAQ Status.vi"("errIN"=w1826, "TL Calling Location"=w1817, "Task ID"=w1812) -> ("error out"=w1823:errorcluster, "Armed?"=w1814:bool)  [unwired: 1 out]
                        n1056 = Divide(x=w1806, y=sgl 2.0) -> (x/y=w1799:sgl)
                        n1057 = case shown="True" w1814 {
                          tunnel: w1823 -> [w1852 w1861]
                          tunnel: [w1857 w1862] -> w1829
                          tunnel: w1812 -> [w1847 _]
                          tunnel: [w1846 w1861] -> w1800
                          tunnel: [w1854 sgl 0.0] -> w1827
                          tunnel: w1816 -> [w1849 _]
                          frame False {
                            w1858 = u16 1 items=["Partial", "Complete"] ("SHOT STATUS")
                            w1859 = u16 0 items=["Partial", "Complete"] ("SHOT STATUS")
                            n1058 = local read "Residual/Separation"() -> (w1853:sgl)
                            n1059 = Concatenate Strings(w1849, "Fb|") -> (w1850:string)
                            n1060 = call "Read TIO Count.vi"("TL Calling Location"=w1850, "error In"=w1852, "task IN"=w1847) -> ("error out"=w1848:errorcluster, "timeout"=w1855:bool, "time (secs)"=w1856:sgl)  [unwired: 1 in, 3 out]
                            n1061 = Divide(x=w1853, y=w1856) -> (x/y=w1854:sgl)
                            n1062 = call "Arm TIO Channel.vi"("error IN"=w1848, "task ID IN"=w1847) -> ("error out"=w1846:errorcluster)  [unwired: 1 in, 2 out]
                            n1063 = Select(t=w1859, s=w1855, f=w1858) -> (s? t:f=w1857:u16)
                          }
                          frame True {
                            w1862 = u16 1 items=["Partial", "Complete"] ("SHOT STATUS")
                          }
                        }
                        n1064 = local write "Current/residual/speed"(w1827) -> ()
                        n1065 = local write "MeasVelScrnSet1"(w1804) -> ()
                        n1066 = local write "MeasVelScrnSet2"(w1805) -> ()
                        n1067 = local write "SHOT STATUS"(w1829) -> ()
                        n1068 = local write "Current/sthotstatus"(w1829) -> ()
                        n1069 = case shown="No Error" w1800 {
                          selector: w1800 -> [w1833 _]
                          frame No Error {
                            # "=false"
                            n1070 = Unbundle By Name(w1833) -> ("status"=w1832:bool)
                            n1071 = Not(x=w1832) -> (.not. x?=w1831:bool)
                            n1072 = local write "readyClock"(w1831) -> ()
                          }
                          frame Error {
                          }
                        }
                        n1073 = local read "SafetyInterlock"() -> (w1801:cluster{"ARMED":bool})
                        n1074 = Bundle By Name(cluster=w1801, "ARMED"=FALSE) -> (w1802:cluster{"ARMED":bool})
                        n1075 = local write "SafetyInterlock"(w1802) -> ()
                        n1076 = call <vilib>:"Simple Error Handler.vi"("error in (no error)"=w1800) -> ("error out"=w1798:errorcluster)  [unwired: 1 in, 7 out]
                      }
                      frame True {
                        # "Error -10600 occurrs in \"Read Count.vi\"\n\n  Possible reason(s): NI-DAQ LV: No setup operation has been performed for the specified resources. Or, some resources require a specific ordering of calls for proper setup.  \n\n  Solution: To avoid this error, you must call the Dig_Line_Config function to setup the direction for each digital line prior to calling the Dig_Grp_Config function."
                        n1077 = local read "MeasVelScrnSet1"() -> (w1866:sgl)
                        n1078 = local read "MeasVelScrnSet2"() -> (w1865:sgl)
                        n1079 = Add(x=w1866, y=w1865) -> (x+y=w1867:sgl)
                        n1080 = Divide(x=w1867, y=sgl 2.0) -> (x/y=w1864:sgl)
                      }
                    }
                  }
                }
                "Current/avg/speed" <- w1749
              }
              frame #1 {
              }
            }
          }
        }
      }
    }
    "SMErr" <- w13
  }
  n1081 = while "U/I Event Handler" {
    shift-right: [w1872] -> _
    shift-left: w7 -> [w1873]
    stop <- FALSE stop-if-true
    n1082 = event shown="[11] \"SampleStyle_1\", \"SampleStyle_2\", \"SampleStyle_3\", \"SampleStyle_4\", \"SampleStyle_5\", \"SampleStyle_6\", \"SampleStyle_0\": Value Change" {
      selector: _ -> [_ _ _ _ _ _ _ _ _ _ _ _ _ _ _ _ _ _ _ _ _ _ _ _ _ _]
      dyn-events: _ -> [_ _ _ _ _ _ _ _ _ _ _ _ _ _ _ _ _ _ _ _ _ _ _ _ _ _]
      timeout: 100 -> [_ _ _ _ _ _ _ _ _ _ _ _ _ _ _ _ _ _ _ _ _ _ _ _ _ _]
      tunnel: w1873 -> [w1877 _ w1894 w1904 w1913 w1923 w1960 w1979 w1987 w2013 w2052 w2095 w2131 w2136 w2174 w2211 w2215 w2225 w2253 w2260 w2279 w2306 w2309 w2337 w2369 _]
      tunnel: [w1877 w1881 w1894 w1901 w1912 w1922 w1959 w1978 w1985 w2022 w2051 w2092 w2131 w2136 w2174 w2211 w2214 w2221 w2253 w2257 w2276 w2306 w2309 w2339 w2369 w2377] -> w1872
      tunnel: [FALSE ("UpdateMetadata") "EXIT" "diagPageVisible" "runtimeMenusVisible" "ARM" "QueryLoad" FALSE ("UpdateMetadata") FALSE ("UpdateMetadata") FALSE ("UpdateMetadata") FALSE ("UpdateMetadata") FALSE ("UpdateMetadata") FALSE ("UpdateMetadata") FALSE ("UpdateMetadata") FALSE ("UpdateMetadata") FALSE ("UpdateMetadata") FALSE ("UpdateMetadata") FALSE ("UpdateMetadata") FALSE ("UpdateMetadata") "Drag Corrected" FALSE ("UpdateMetadata") "PublishNewRecords" FALSE ("UpdateMetadata") FALSE ("UpdateMetadata") "RefreshMetadata" FALSE ("UpdateMetadata") FALSE ("UpdateMetadata")] -> w1871
      event Timeout {
        n1083 = event-data() -> ()  [unwired: 2 out]
        n1084 = Get Date/Time In Seconds() -> (seconds since 1Jan1904=w1879:timestamp)
        n1085 = Format Date/Time String(seconds (now)=w1879) -> (date/time string=→"TimeNow":string)  [unwired: 2 out]
      }
      event "EXIT": Value Change {
        n1086 = event-data() -> ()  [unwired: 2 out]
        n1087 = property on="Property Node" class="Application"(error in=errorcluster {"status"=FALSE, "code"=0, "source"=""} ("error in (no error)")) -> (error out=w1881:errorcluster, "Application:Kind"=w1886:T37)  [unwired: 1 in, 1 out]
        n1088 = Two Button Dialog(message="Exit BIMS Collector?\nAll Unsaved data will be lost.", 1:"NO" ("F button name (\"Cancel\")"), 2:"YES" ("T button name (\"OK\")")) -> (T button?=w1887:bool)
        n1089 = case shown="\"Development System\"" w1886 {
          tunnel: w1887 -> [w1888 w1889 w1890]
          frame Default {
            n1090 = Stop(stop? (T)=w1888) -> ()
          }
          frame "Development System" {
            n1091 = Stop(stop? (T)=w1889) -> ()
          }
          frame "Run Time System" {
            n1092 = Quit LabVIEW(quit? (T)=w1890) -> ()
          }
        }
      }
      event "diagPageVisible": Value Change {
        # "Toggles display of \"Internal Use\" tab for diagnostics purposes"
        # "Key navigation ONLY: Cntrl-Shift-F11"
        n1093 = event-data() -> ("NewVal"=w1897:bool)  [unwired: 1 out]
        n1094 = property on="aboutTabCntrl" class="TabCtl (strict)"(error in=errorcluster {"status"=FALSE, "code"=0, "source"=""} ("error in (no error)")) -> (error out=w1896:errorcluster, "Pages"=w1900:refnum<vi>[])  [unwired: 1 in, 1 out]
        n1095 = Index Array(array=w1900, index=3) -> (element=w1898:refnum<vi>)
        n1096 = property on="Property Node" class="Page"(reference=w1898, error in=w1896, "PageVis"=w1897) -> (error out=w1895:errorcluster)  [unwired: 1 out]
        n1097 = property on="diagPageVisible" class="Bool (strict)"(error in=w1895, "Value"=w1897) -> (error out=w1892:errorcluster)  [unwired: 1 in, 1 out]
        n1098 = call <vilib>:"General Error Handler.vi"("error in (no error)"=w1892) -> ()  [unwired: 2 in, 13 out]
      }
      event "runtimeMenusVisible": Value Change {
        # "Key navigation ONLY: Cntrl-Shift-F10"
        n1099 = event-data() -> ("NewVal"=w1906:bool)  [unwired: 1 out]
        n1100 = control-ref of="This VI"() -> (w1905:refnum<vi>)
        n1101 = property class="VI"(reference=w1905, error in=w1904, "Front Panel.ShowMenuBar"=w1906) -> (reference out=w1903:refnum<vi>, error out=w1902:errorcluster)
        n1102 = Close Reference(reference=w1903, error in (no error)=w1902) -> (error out=w1901:errorcluster)
      }
      event "ARM": Value Change {
        # "This section will arm the system"
        n1103 = event-data() -> ()  [unwired: 2 out]
        n1104 = disable-structure shown="Disabled" {
          frame Disabled {
            "DIO" <- u32 21 ("DIO")
          }
          frame Enabled {
          }
        }
        n1105 = Bundle By Name(cluster=cluster{"ARMED":bool} {"ARMED"=FALSE} ("Safety_Interlock"), "ARMED"=TRUE) -> (→"SafetyInterlock":cluster{"ARMED":bool})
        n1106 = local write "SUBMIT DATE/TIME"("" ("Empty String Constant")) -> ()
        n1107 = local read "MeasSrc"() -> (w1914:T6)
        n1108 = case shown="\"Screens\"" w1914 {
          tunnel: w1913 -> [w1917 w1918 w1920]
          tunnel: [w1917 w1918 w1920] -> w1912
          frame "Simulated", Default {
          }
          frame "Radar" {
          }
          frame "Screens" {
            n1109 = local write "readyClock"(TRUE ("readyClock")) -> ()
          }
        }
      }
      event "QueryLoad": Value Change {
        w1928 = "%x" ("time format string (%c)")
        w1944 = "" ("replace string (\"\")")
        # "This section plots  Impact velocity vs. loadingdata"
        n1110 = event-data() -> ()  [unwired: 2 out]
        n1111 = Format Date/Time String(time format string (%c)=w1928, seconds (now)="lkupStartDate") -> (date/time string=w1927:string)  [unwired: 1 out]
        n1112 = Format Date/Time String(time format string (%c)=w1928, seconds (now)="lkupEndDate") -> (date/time string=w1926:string)  [unwired: 1 out]
        n1113 = call "Trim String.vi"("inStr"="Powder.freeTxt") -> ("outStr"=w1942:string)
        n1114 = call "Trim String.vi"("inStr"="Threat.freeTxt") -> ("outStr"=w1943:string)
        n1115 = invoke on="v50_table" class="Tbl" method="Reinit To Default"(error in=w1923) -> (error out=w1935:errorcluster)  [unwired: 2 in, 2 out]
        n1116 = invoke on="Vel.vs.Loading" class="WFGraph (strict)" method="Reinit To Default"(error in=w1935) -> (error out=w1930:errorcluster)  [unwired: 2 in, 2 out]
        n1117 = Format Into String(format string="SELECT TOP %d dbsrc.experiment.threat, dbsrc.shots.loading, dbsrc.shots.impact, dbsrc.experiment.powder, dbsrc.shots.date from dbsrc.shots, dbsrc.experiment where dbsrc.shots.expt = dbsrc.experiment.expt and dbsrc.shots.loading > 0 and dbsrc.shots.date between '%s' and '%s' and dbsrc.shots.impact between 10 and 5000 and dbsrc.experiment.powder like '%%%s%%' and dbsrc.experiment.threat like '%%%s%%' and experiment.threat<>'' order by dbsrc.experiment.threat, dbsrc.shots.loading, dbsrc.shots.impact;" ("Format String"), error in=w1930, "maxRecs", w1927, w1926, w1942, w1943) -> (resulting string=w1948:string, error out=w1933:errorcluster)  [unwired: 1 in]
        n1118 = Search and Replace String(input string=w1948, search string=" and experiment.powder like '%%'", replace string=w1944, error in=w1933) -> (result string=w1946:string, error out=w1934:errorcluster)  [unwired: 6 out]
        n1119 = Search and Replace String(input string=w1946, search string="and experiment.threat like '%%'", replace string=w1944, error in=w1934) -> (result string=w1937:string, error out=w1932:errorcluster)  [unwired: 6 out]
        n1120 = call "Fetch Data (SubVI).vi"("error IN"=w1932, "query string"=w1937) -> ("error OUT"=w1922:errorcluster, "recordset data"=w1938:string[][])  [unwired: 4 out]
        "v50_table" <- w1938
        n1121 = Fract/Exp String To Number(string=w1938) -> (number=w1952:dbl[][])  [unwired: 4 out]
        n1122 = Array Size(array=w1938) -> (size(s)=w1940:i32[])
        n1123 = Index Array(array=w1940) -> (element=→"ActualNumRecs":i32)  [unwired: 1 in]
        n1124 = Index Array(array=w1952, index (col)=2 ("Disabled Index (col)")) -> (element=w1951:dbl[])  [unwired: 1 in]
        n1125 = Index Array(array=w1952, index (col)=1 ("Disabled Index (col)")) -> (element=w1950:dbl[])  [unwired: 1 in]
        n1126 = Bundle(w1950, w1951) -> (→"Vel.vs.Loading":cluster{dbl[], dbl[]})  [unwired: 1 out]
      }
      event "ThreatGroups": Value Change {
        n1127 = event-data() -> ()  [unwired: 2 out]
        n1128 = control-ref of="ThreatGroups"() -> (w1961:refnum<vi>)
        n1129 = property on="Property Node" class="Ring (strict)"(reference=w1961, error in=w1960) -> (error out=w1958:errorcluster, "RingText.Text"=w1956:string)  [unwired: 1 out]
        n1130 = Not Equal?(x=w1956, y="") -> (x != y?=w1955:bool)
        n1131 = case shown="True" w1955 {
          tunnel: w1956 -> [_ w1971]
          tunnel: [w1963 w1969] -> w1959
          tunnel: w1958 -> [w1966 w1968]
          frame False {
            n1132 = property on="ThreatDetails" class="Ring (strict)"(error in=w1966, "Strings []"=string[] [], "Value"=u16 0 ("Value (Signaling)")) -> (error out=w1964:errorcluster)  [unwired: 1 in, 1 out]
            n1133 = invoke on="threatDetails" class="Clust (strict)" method="Reinit To Default"(error in=w1964) -> (error out=w1963:errorcluster)  [unwired: 2 in, 2 out]
          }
          frame True {
            n1134 = call "Select Threat Details.vi"("threatGroup"=w1971) -> ("threatDetails"=w1970:string[])  [unwired: 1 out]
            n1135 = property on="ThreatDetails" class="Ring (strict)"(error in=w1968, "Strings []"=w1970, "Val(Sgnl)"=u16 0 ("Value (Signaling)")) -> (error out=w1969:errorcluster)  [unwired: 1 in, 1 out]
          }
        }
      }
      event "panelSearch": Value Change {
        # "This section returns past panels"
        n1136 = event-data() -> ()  [unwired: 2 out]
        n1137 = control-ref of="pastPanels"() -> (w1981:refnum<vi>)
        n1138 = control-ref of="Mfr_0"() -> (w1975:refnum<vi>)
        n1139 = control-ref of="SampleStyle_0"() -> (w1976:refnum<vi>)
        n1140 = control-ref of="Requestors_0"() -> (w1974:refnum<vi>)
        n1141 = control-ref of="ThreatSize_0"() -> (w1973:refnum<vi>)
        n1142 = call "queryPanels (SubVI).vi"("ThreatSize_0"=w1973, "Mfr_0"=w1975, "Requestors_0"=w1974, "Style_0"=w1976, "error in"=w1979, "srchParams"="srchParams", "pastPanels"=w1981) -> ("error out"=w1978:errorcluster, "recordset data"=→"pastPanels":string[][], "actualNumPanels"=→"actualNumPanels":i32)  [unwired: 2 in]
      }
      event "pastPanels": Mouse Up {
        n1143 = event-data() -> ("CtlRef"=w1995:refnum<vi>)  [unwired: 1 out]
        n1144 = property on="Property Node" class="Tbl (strict)"(reference=w1995, error in=w1987) -> (error out=w1986:errorcluster, "Value"=w1994:string[][], "EditPos"=w1993:T38)  [unwired: 1 out]
        n1145 = Unbundle By Name(w1993) -> ("Row"=w1992:i32)
        n1146 = Index Array(array=w1994, index (row)=w1992, index (col)=0 ("disabled index (col)")) -> (element=w1991:string)
        n1147 = Scan From String(input string=w1991, error in=w1986, default 1=1 ("Record #")) -> (error out=w1985:errorcluster, output 1=w1989:i32)  [unwired: 2 in, 2 out]
        n1148 = local write "Record #"(w1989) -> ()
      }
      event "ThreatDetails", "SampleID": Value Change {
        # "A Sample ID is entered"
        # "A range is selected"
        # "A measurement requires the selection of a threat,\nso delay enabling the \"Measure\" tab until a grain wt\nis chosen."
        n1149 = event-data() -> ()  [unwired: 2 out]
        n1150 = control-ref of="ThreatGroups"() -> (w2014:refnum<vi>)
        n1151 = control-ref of="ThreatDetails"() -> (w2011:refnum<vi>)
        n1152 = call "Get Projectile Atributes from ThreatGroupDetail.vi"("error IN"=w2013, "ThreatDetail"=w2011, "ThreatGroup"=w2014) -> ("error out"=w2012:errorcluster, "projectileAttribs"=w2010:T39)  [unwired: 1 out]
        "threatDetails" <- w2010
        n1153 = Unbundle By Name(w2010) -> ("grainSize"=w2003:string)
        n1154 = Equal?(x=w2003, y="") -> (x = y?=w2004:bool)
        n1155 = case shown="False" w2004 {
          tunnel: w2003 -> [w2032 _]
          tunnel: [w2031 u16 0 ("GrainSize")] -> w2009
          frame False {
            # "A grain size is selected"
            n1156 = Scan From String(input string=w2032) -> (output 1=w2031:u16)  [unwired: 3 in, 4 out]
            "GrainSize" <- w2031
          }
          frame True {
            # "A grain size not selected"
          }
        }
        n1157 = Equal?(x=w2003, y="") -> (x = y?=w2029:bool)
        n1158 = local read "rangeSetup"() -> (w2026:u16)
        n1159 = case shown="False" w2029 {
          tunnel: [w2036 sgl 0.0] -> w2025
          tunnel: w2003 -> [w2034 _]
          frame False {
            w2038 = sgl 0.0  # sgl
            n1160 = Scan From String(format string="%f " ("Format String"), input string=w2034, default 1=w2038) -> (output 1=w2037:sgl)  [unwired: 2 in, 3 out]
            n1161 = disable-structure shown="Enabled" {
              disable-tunnel: w2037 -> [w2041 w2042]
              disable-tunnel: [w2040 w2042] -> w2036
              frame Disabled {
                n1162 = Multiply(x=sgl 0.06479891, y=w2041) -> (x*y=w2040:sgl)
              }
              frame Enabled {
              }
            }
          }
          frame True {
          }
        }
        "Projectile Mass" <- w2025
        n1163 = local read "SampleID"() -> (w2008:string)
        n1164 = Greater Than 0?(x=w2026) -> (x > 0?=w2027:bool)
        n1165 = Greater Than 0?(x=w2009) -> (x > 0?=w2028:bool)
        n1166 = Not Equal?(x=w2008, y="") -> (x != y?=w2006:bool)
        n1167 = Compound Arithmetic op=AND(w2028, w2027, w2006) -> (w2001:bool)
        n1168 = property on="mainTabCntrl" class="TabCtl (strict)"(error in=w2012) -> (error out=w2018:errorcluster, "Pages"=w2021:refnum<vi>[])  [unwired: 1 in, 1 out]
        n1169 = Not(x=w2001) -> (.not. x?=w2017:bool)
        n1170 = Index Array(array=w2021, index=1) -> (element=w2019:refnum<vi>)
        n1171 = Select(t=T15."Page Enabled" ("Page Enabled State"), s=w2001, f=T15."Page Disabled & Grayed" ("Page Enabled State")) -> (s? t:f=w2000:T15)
        n1172 = property on="Property Node" class="Page"(reference=w2019, error in=w2018, "PageEnb"=w2000) -> (error out=w2016:errorcluster)  [unwired: 1 out]
        n1173 = Select(t=T14."Enabled" ("Disabled"), s=w2001, f=T14."Disabled and Grayed Out" ("Disabled")) -> (s? t:f=w1998:T14)
        n1174 = property on="ARM" class="Bool"(error in=w2016, "Disabled"=w1998) -> (error out=w2024:errorcluster)  [unwired: 1 in, 1 out]
        n1175 = property on="addShot" class="Bool"(error in=w2024, "Disabled"=w1998) -> (error out=w2023:errorcluster)  [unwired: 1 in, 1 out]
        n1176 = property on="instruct_addShot" class="Str"(error in=w2023, "Visible"=w2017) -> (error out=w2022:errorcluster)  [unwired: 1 in, 1 out]
      }
      event "Mfr_1", "Mfr_2", "Mfr_3", "Mfr_4", "Mfr_5", "Mfr_6", "Mfr_0": Value Change {
        n1177 = event-data() -> ("CtlRef"=w2060:refnum<vi>)  [unwired: 1 out]
        n1178 = property on="Property Node" class="Ring (strict)"(reference=w2060, error in=w2052) -> (error out=w2050:errorcluster, "Label.Text"=w2056:string, "RingText.Text"=w2057:string)  [unwired: 1 out]
        n1179 = flat-sequence {
          tunnel: ["Mfr_1"] -> _
          tunnel: ["Mfr_2"] -> _
          tunnel: ["Mfr_3"] -> _
          tunnel: ["Mfr_4"] -> _
          tunnel: ["Mfr_5"] -> _
          tunnel: ["Mfr_6"] -> _
          frame #0 {
          }
        }
        n1180 = call "Select Sample Style.vi"("error IN"=w2050, "Mfr"=w2057) -> ("error Out"=w2049:errorcluster, "SampleStyles"=w2045:string[])  [unwired: 4 out]
        n1181 = Scan From String(format string="Mfr_%d", input string=w2056, error in=w2049, default 1=0 ("Mfr#")) -> (error out=w2046:errorcluster, output 1=w2055:i32)  [unwired: 1 in, 2 out]
        n1182 = case shown="1" w2055 {
          tunnel: [w2072 w2075 w2078 w2081 w2084 w2087 w2090] -> w2054
          tunnel: [w2071 w2074 w2077 w2080 w2083 w2086 w2089] -> w2047
          tunnel: w2046 -> [w2071 w2074 w2077 w2080 w2083 w2086 w2089]
          tunnel: w2045 -> [w2070 w2073 w2076 w2079 w2082 w2085 w2088]
          tunnel: [w2069 w2073 w2076 w2079 w2082 w2085 w2088] -> w2044
          frame 0, Default {
            n1183 = Delete From Array(array=w2070, length=1, index=0) -> (array with subset deleted=w2069:string[])  [unwired: 1 out]
            n1184 = control-ref of="SampleStyle_0"() -> (w2072:refnum<vi>)
          }
          frame 1 {
            n1185 = control-ref of="SampleStyle_1"() -> (w2075:refnum<vi>)
          }
          frame 2 {
            n1186 = control-ref of="SampleStyle_2"() -> (w2078:refnum<vi>)
          }
          frame 3 {
            n1187 = control-ref of="SampleStyle_3"() -> (w2081:refnum<vi>)
          }
          frame 4 {
            n1188 = control-ref of="SampleStyle_4"() -> (w2084:refnum<vi>)
          }
          frame 5 {
            n1189 = control-ref of="SampleStyle_5"() -> (w2087:refnum<vi>)
          }
          frame 6 {
            n1190 = control-ref of="SampleStyle_6"() -> (w2090:refnum<vi>)
          }
        }
        n1191 = property on="Property Node" class="Ring (strict)"(reference=w2054, error in=w2047, "Strings []"=w2044, "Val(Sgnl)"=u16 0 ("Value (Signaling)")) -> (error out=w2051:errorcluster)  [unwired: 1 out]
      }
      event "SampleStyle_1", "SampleStyle_2", "SampleStyle_3", "SampleStyle_4", "SampleStyle_5", "SampleStyle_6", "SampleStyle_0": Value Change {
        n1192 = event-data() -> ("CtlRef"=w2101:refnum<vi>)  [unwired: 1 out]
        n1193 = call "Get Sample Style Atributes.vi"("StyleNumRef"=w2101) -> ("SampleSpecs"=w2096:T40)  [unwired: 1 in]
        n1194 = flat-sequence {
          tunnel: ["SampleStyle_1"] -> _
          tunnel: ["SampleStyle_2"] -> _
          tunnel: ["SampleStyle_3"] -> _
          tunnel: ["SampleStyle_4"] -> _
          tunnel: ["SampleStyle_5"] -> _
          tunnel: ["SampleStyle_6"] -> _
          frame #0 {
          }
        }
        n1195 = property on="Property Node" class="Ring (strict)"(reference=w2101, error in=w2095) -> (error out=w2094:errorcluster, "Label.Text"=w2100:string)  [unwired: 1 out]
        n1196 = Scan From String(format string="SampleStyle_%d", input string=w2100, error in=w2094, default 1=0 ("default value 1")) -> (error out=w2093:errorcluster, output 1=w2098:i32)  [unwired: 1 in, 2 out]
        n1197 = case shown="1" w2098 {
          tunnel: w2096 -> [w2110 w2113 w2116 w2119 w2122 w2125 w2128]
          tunnel: w2093 -> [w2109 w2112 w2115 w2118 w2121 w2124 w2127]
          tunnel: [w2108 w2111 w2114 w2117 w2120 w2123 w2126] -> w2092
          frame 0, Default {
            n1198 = property on="SampleAttribs_0" class="Clust (strict)"(error in=w2109, "Val(Sgnl)"=w2110) -> (error out=w2108:errorcluster)  [unwired: 1 in, 1 out]
            "SampleAttribs_0" <- w2110
          }
          frame 1 {
            n1199 = property on="SampleAttribs_1" class="Clust (strict)"(error in=w2112, "Val(Sgnl)"=w2113) -> (error out=w2111:errorcluster)  [unwired: 1 in, 1 out]
            "SampleAttribs_1" <- w2113
          }
          frame 2 {
            n1200 = property on="SampleAttribs_2" class="Clust (strict)"(error in=w2115, "Val(Sgnl)"=w2116) -> (error out=w2114:errorcluster)  [unwired: 1 in, 1 out]
            "SampleAttribs_2" <- w2116
          }
          frame 3 {
            n1201 = property on="SampleAttribs_3" class="Clust (strict)"(error in=w2118, "Val(Sgnl)"=w2119) -> (error out=w2117:errorcluster)  [unwired: 1 in, 1 out]
            "SampleAttribs_3" <- w2119
          }
          frame 4 {
            n1202 = property on="SampleAttribs_4" class="Clust (strict)"(error in=w2121, "Val(Sgnl)"=w2122) -> (error out=w2120:errorcluster)  [unwired: 1 in, 1 out]
            "SampleAttribs_4" <- w2122
          }
          frame 5 {
            n1203 = property on="SampleAttribs_5" class="Clust (strict)"(error in=w2124, "Val(Sgnl)"=w2125) -> (error out=w2123:errorcluster)  [unwired: 1 in, 1 out]
            "SampleAttribs_5" <- w2125
          }
          frame 6 {
            n1204 = property on="SampleAttribs_6" class="Clust (strict)"(error in=w2127, "Val(Sgnl)"=w2128) -> (error out=w2126:errorcluster)  [unwired: 1 in, 1 out]
            "SampleAttribs_6" <- w2128
          }
        }
      }
      event "SHOTS", "Sort by AVG": Value Change {
        n1205 = event-data() -> ()  [unwired: 2 out]
        n1206 = local read "Site"() -> (w2129:string)
        n1207 = local read "SHOTS"() -> (w2133:T7[])
        n1208 = call "Update Shot Table.vi"("Sort by AVG"="Sort by AVG", "Site"=w2129, "shotsArr"=w2133) -> ("shotTable OUT"=→"Table of Shots":string[][])
      }
      event "Layer_1.plyNum", "Layer_2.plyNum", "Layer_3.plyNum", "Layer_4.plyNum", "Layer_5.plyNum", "Layer_6.plyNum", "SampleAttribs_1.ozPerYd2", "SampleAttribs_2.ozPerYd2", "SampleAttribs_3.ozPerYd2", "SampleAttribs_4.ozPerYd2", "SampleAttribs_5.ozPerYd2", "SampleAttribs_6.ozPerYd2": Value Change {
        n1209 = event-data() -> ()  [unwired: 2 out]
        n1210 = global read "BIMS_Collector Globals.vi" "SampleAttribs"() -> (w2144:T23)
        n1211 = Build Array("Layer_1", "Layer_2", "Layer_3", "Layer_4", "Layer_5", "Layer_6") -> (w2137:T41)
        n1212 = global write "BIMS_Collector Globals.vi" "LayerSpecs"(w2137) -> ()
        n1213 = for {
          tunnel: w2137 -> [w2165] mode=indexing
          shift-right: [w2167] -> w2146
          shift-left: 0 -> [w2166]
          tunnel: [w2164] -> w2156 mode=indexing
          tunnel: w2144 -> [w2162] mode=indexing
          n1214 = Unbundle By Name(w2162) -> ("ozPerYd2"=w2158:string)
          n1215 = Equal?(x=w2158, y="" ("Empty String Constant")) -> (x = y?=w2157:bool)
          n1216 = case shown="False" w2157 {
            tunnel: [w2171 sgl 0.0 ("default value 1")] -> w2161
            tunnel: w2158 -> [w2168 _]
            frame False {
              n1217 = Scan From String(format string="%f", input string=w2168, default 1=sgl 0.0 ("default value 1")) -> (output 1=w2171:sgl)  [unwired: 2 in, 3 out]
            }
            frame True {
            }
          }
          n1218 = Unbundle By Name(w2165) -> ("plyNum"=w2163:i32)
          n1219 = Add(x=w2166, y=w2163) -> (x+y=w2167:i32)
          n1220 = To Single Precision Float(number=w2163) -> (single precision float=w2160:sgl)
          n1221 = Multiply(x=w2160, y=w2161) -> (x*y=w2164:sgl)
        }
        "totalNumLayers" <- w2146
        n1222 = Divide(x=w2156, y=sgl 144.0) -> (x/y=w2154:sgl[])
        n1223 = Index Array(array=w2154) -> (element #1=→"fab1_totalWt":sgl, element #2=→"fab2_totalWt":sgl, element #3=→"fab3_totalWt":sgl, element #4=→"fab4_totalWt":sgl, element #5=→"fab5_totalWt":sgl, element #6=→"fab6_totalWt":sgl)  [unwired: 6 in]
        n1224 = Add Array Elements(numeric array=w2154) -> (sum=→"totalBAW":sgl)
      }
      event "clayCalArray": Value Change {
        n1225 = event-data() -> ()  [unwired: 2 out]
        n1226 = for {
          tunnel: "clayCalArray" -> [w2200] mode=indexing
          shift-right: [w2199] -> w2182
          shift-left: "" ("Empty String Constant") -> [w2197]
          shift-right: [w2194] -> w2178
          shift-left: i16[] [] -> [w2193]
          n1227 = Greater Than 0?(x=w2200) -> (x > 0?=w2201:bool)
          n1228 = case shown="False" w2201 {
            tunnel: w2200 -> [_ w2207]
            tunnel: ["##" ("clayCalib") w2209] -> w2198
            tunnel: w2197 -> [w2204 w2208]
            tunnel: [w2204 w2208] -> w2196
            tunnel: [w2202 w2206] -> w2194
            tunnel: w2193 -> [w2202 w2205]
            frame False {
            }
            frame True {
              n1229 = Format Into String(w2207) -> (resulting string=w2209:string)  [unwired: 3 in, 1 out]
              n1230 = Build Array (concatenate)(w2205, w2207) -> (w2206:i16[])
            }
          }
          n1231 = Concatenate Strings(w2196, w2198, "-" ("string")) -> (w2199:string)
        }
        n1232 = String Length(string=w2182) -> (length=w2183:i32)
        n1233 = Add Array Elements(numeric array=w2178) -> (sum=w2187:i16)
        n1234 = Array Size(array=w2178) -> (size(s)=w2188:i32)
        n1235 = Decrement(x=w2183) -> (x-1=w2180:i32)
        n1236 = To Single Precision Float(number=w2187) -> (single precision float=w2186:sgl)
        n1237 = To Single Precision Float(number=w2188) -> (single precision float=w2176:sgl)
        n1238 = String Subset(string=w2182, length (rest)=w2180) -> (substring=w2181:string)  [unwired: 1 out]
        n1239 = Equal To 0?(x=w2176) -> (x = 0?=w2175:bool)
        n1240 = local write "clayCalib"(w2181) -> ()
        n1241 = case shown="True" w2175 {
          tunnel: w2186 -> [w2191 w2192]
          tunnel: w2176 -> [w2190 _]
          tunnel: [w2189 w2192] -> w2185
          frame False {
            n1242 = Divide(x=w2191, y=w2190) -> (x/y=w2189:sgl)
          }
          frame True {
          }
        }
        "clayAverage" <- w2185
      }
      event "reportV50_History": Value Change {
        n1243 = event-data() -> ()  [unwired: 2 out]
        n1244 = local write "lookupRec"(TRUE ("lookupRec")) -> ()
      }
      event "Methods": Value Change {
        n1245 = event-data() -> ("CtlRef"=w2219:refnum<vi>)  [unwired: 1 out]
        n1246 = call "Dropdown Selection (SubVI).vi"("reference"=w2219) -> ("element"=w2218:string)
        n1247 = Equal?(x=w2218, y="V50") -> (x = y?=w2216:bool)
        n1248 = property on="minV50" class="DigNum (strict)"(error in=w2215, "Visible"=w2216) -> (error out=w2214:errorcluster)  [unwired: 1 in, 1 out]
      }
      event "rangeSetup": Value Change {
        n1249 = event-data() -> ("NewVal"=w2229:u16)  [unwired: 1 out]
        n1250 = case shown="2" w2229 {
          tunnel: ["0" ("section") "5.0" ("section") "7.5" ("section") "45.0" ("section")] -> w2235
          frame 0, Default {
          }
          frame 1 {
          }
          frame 2 {
          }
          frame 3 {
          }
        }
        n1251 = local read "configPath"() -> (w2237:path)
        n1252 = local read "GrainSize"() -> (w2228:u16)
        n1253 = Greater Than 0?(x=w2229) -> (x > 0?=w2232:bool)
        n1254 = Greater Than 0?(x=w2228) -> (x > 0?=w2230:bool)
        n1255 = call <vilib>:"Open Config Data (compatibility).vi"("error in (no error)"=w2225, "configuration file path"=w2237) -> ("error out"=w2245:errorcluster, "refnum"=w2247:T35)  [unwired: 7 in, 1 out]
        n1256 = And(x=w2232, y=w2230) -> (x .and. y?=w2231:bool)
        n1257 = call-poly <vilib>:"Write Key.vi"("write raw string? (F)"=TRUE, "section"="Ballistic Parameters", "error in (no error)"=w2245, "value"=w2235, "key"="MidPoint To Target Distance", "refnum"=w2247) -> ("error out"=w2244:errorcluster, "refnum out"=w2243:T35)  [unwired: 4 out]
        n1258 = call <vilib>:"Close Config Data.vi"("error in (no error)"=w2244, "refnum"=w2243) -> ("error out"=w2236:errorcluster)  [unwired: 1 in, 8 out]
        n1259 = Not(x=w2231) -> (.not. x?=w2241:bool)
        n1260 = Select(t=u8 0 ("y"), s=w2231, f=u8 2 ("y")) -> (s? t:f=w2227:u8)
        n1261 = Scan From String(input string=w2235, error in=w2236, default 1=sgl 0.0 ("default value 1")) -> (error out=w2224:errorcluster, output 1=w2234:sgl)  [unwired: 2 in, 2 out]
        n1262 = local write "mid_to_targ_dist"(w2234) -> ()
        n1263 = property on="ARM" class="Bool"(error in=w2224, "Disabled"=w2227) -> (error out=w2223:errorcluster)  [unwired: 1 in, 1 out]
        n1264 = property on="addShot" class="Bool"(error in=w2223, "Disabled"=w2227) -> (error out=w2222:errorcluster)  [unwired: 1 in, 1 out]
        n1265 = property on="instruct_addShot" class="Str"(error in=w2222, "Visible"=w2241) -> (error out=w2221:errorcluster)  [unwired: 1 in, 1 out]
        "instruct_addShot" <- "RANGE SETUP and THREAT must be selected before shots can be added." ("instruct_addShot")
      }
      event "Drag Corrected", "maxDev": Value Change {
        n1266 = event-data() -> ()  [unwired: 2 out]
        n1267 = local write "processShots"(TRUE ("ProcessShots")) -> ()
      }
      event "MC Listbox of Shots": Mouse Up {
        n1268 = event-data() -> ()  [unwired: 2 out]
        n1269 = flat-sequence {
          tunnel: w2260 -> [w2264]
          tunnel: [w2262] -> w2259
          tunnel: ["MC Listbox of Shots"] -> w2256
          tunnel: w2259 -> [w2268]
          tunnel: [w2267] -> w2258
          tunnel: w2256 -> [_]
          tunnel: w2258 -> [w2273]
          tunnel: [w2271] -> w2257
          frame #0 {
            n1270 = property on="Table of Shots" class="Tbl (strict)"(error in=w2264) -> (error out=w2263:errorcluster, "Value"=w2265:string[][])  [unwired: 1 in, 1 out]
            n1271 = local write "STOP (Shots MC LB)"(FALSE ("STOP (Shots MC LB)")) -> ()
            n1272 = property on="MC Listbox of Shots" class="MCListbox (strict)"(error in=w2263, "ItemNames"=w2265) -> (error out=w2262:errorcluster)  [unwired: 1 in, 1 out]
          }
          frame #1 {
            n1273 = control-ref of="MC Listbox of Shots"() -> (w2270:refnum<vi>)
            n1274 = control-ref of="STOP (Shots MC LB)"() -> (w2269:refnum<vi>)
            n1275 = call "multicolumn listbox sort.vi"("error IN"=w2268, "Bool Refnum"=w2269, "MCListbox Refnum"=w2270) -> ("error out"=w2267:errorcluster)  [unwired: 4 in]
          }
          frame #2 {
            n1276 = property on="MC Listbox of Shots" class="MCListbox (strict)"(error in=w2273) -> (error out=w2272:errorcluster, "ItemNames"=w2274:string[][])  [unwired: 1 in, 1 out]
            n1277 = property on="Table of Shots" class="Tbl (strict)"(error in=w2272, "Val(Sgnl)"=w2274) -> (error out=w2271:errorcluster)  [unwired: 1 in, 1 out]
          }
        }
      }
      event "PublishNewRecords": Value Change {
        w2289 = "\\" ("string")
        w2292 = TRUE  # overwrite (F)
        # "2. INSERT new records to Experiments and  \n      Shots tables in local Export.mdb file."
        # "1. SELECT new records from local MDB \n     by comparing against last record numbers \n     found in IMPORT table on BIMS server."
        # "Pushes latest ballistics performance data up to BIMS Server\n\n - Attempts connection with server (reports connection success in msgbox)\n - If successful:\n   - Exports all experiment/shot records since last table marker to [site].mdb file\n   - Sends export.mdb file to drop location on BIMS File Server\n   - Executes SSIS package to import records from export.mdb file\n - Otherwise provides option to try again or cancel"
        # "3. Copy Export.mdb file to [sitename].mdb in [sitename] \n      FileDrop folder on BIMS server."
        n1278 = event-data() -> ()  [unwired: 2 out]
        n1279 = property on="Loading" class="Ring (strict)"(error in=w2279, "Visible"=TRUE) -> (error out=w2278:errorcluster)  [unwired: 1 in, 1 out]
        n1280 = local read "Site"() -> (w2284:string)
        n1281 = call "Export New Records.vi"("error IN"=w2278, "Site"=w2284) -> ("error out"=w2294:errorcluster)  [unwired: 3 in, 6 out]
        n1282 = Concatenate Strings("\\\\" ("string"), "Server", w2289, "icela_" ("string"), "Server", "\\BIMS\\File Drops" ("string"), w2289, w2284, w2289, w2284, ".mdb" ("string")) -> (w2286:string)
        n1283 = String To Path(string=w2286) -> (path=w2282:path)
        n1284 = Copy(8:w2294, 9:w2292, 10:w2282, 11:path "C:/Ballistics/Export.mdb" ("source path")) -> (0:w2291:errorcluster)  [unwired: 3 out]
        n1285 = case shown="No Error" w2291 {
          selector: w2291 -> [w2296 w2298]
          tunnel: [w2296 w2297] -> w2277
          frame No Error {
            n1286 = One Button Dialog(message="New sample performance records submitted \nto BIMS Warehouse successfully.\n\nPublishing will occur in under five minutes.") -> ()  [unwired: 2 out]
          }
          frame Error {
            n1287 = call <vilib>:"General Error Handler.vi"("error in (no error)"=w2298) -> ("error out"=w2297:errorcluster)  [unwired: 2 in, 12 out]
          }
        }
        n1288 = property on="Loading" class="Ring (strict)"(error in=w2277, "Visible"=FALSE) -> (error out=w2276:errorcluster)  [unwired: 1 in, 1 out]
      }
      event "arrIDC": Mouse Up {
        n1289 = event-data() -> ()  [unwired: 2 out]
        "velProfile" <- cluster{dbl, dbl}[] [] ("velProfile")
        "arrIDC" <- dbl[] [] ("arrIDC")
        "relativeTime" <- cluster{"ts2":dbl, "ts3":dbl, "ts1":dbl} {"ts2"=0.0, "ts3"=0.0, "ts1"=0.0} ("relativeTime")
        "velMeasProf" <- T8 {"v2"=0.0, "vB"=0.0, "vOuter"=0.0, "v1"=0.0, "vA"=0.0, "vInner"=0.0} ("velMeasProf")
        "velCompProf" <- cluster{"vStrike":dbl, "vA":dbl} {"vStrike"=0.0, "vA"=0.0} ("velCompProf")
        "displacement" <- T9 {"ds_v2"=6.75, "ds2"=5.0833, "ds_vB"=4.9167, "ds3"=4.75, "ds_vAvg"=6.9167, "ds_v1"=7.0833, "ds1"=8.75, "ds_vA"=8.9167, "ds0"=9.0833} ("displacement")
      }
      event "SampleBackings": Value Change {
        # "Clay is the default sample backing material.\n\n  If another selection is made, then grey out and disable all controls relating to clay."
        n1290 = event-data() -> ()  [unwired: 2 out]
        n1291 = case shown="0, Default" "SampleBackings" {
          tunnel: [T14."Disabled and Grayed Out" ("Disabled") T14."Enabled" ("Disabled") T14."Disabled and Grayed Out" ("Disabled")] -> w2307
          frame 0, Default {
          }
          frame 1 {
          }
          frame 2.. {
          }
        }
        n1292 = property on="clayCalArray" class="Arr (strict)"("DisabledEnum"=w2307) -> ()  [unwired: 2 in, 2 out]
        n1293 = property on="clayAverage" class="DigNum (strict)"("DisabledEnum"=w2307) -> ()  [unwired: 2 in, 2 out]
        n1294 = property on="clayTemp" class="DigNum (strict)"("DisabledEnum"=w2307) -> ()  [unwired: 2 in, 2 out]
      }
      event "RefreshMetadata": Value Change {
        # "Pulls latest metadata down from BIMS Database Server\n - Attempts connection with server \n        (reports failure if connection is unsuccessful)\n - If successful:\n   - Updates local database records from server\n   - Updates dropdown listboxes from local database"
        n1295 = event-data() -> ()  [unwired: 2 out]
        n1296 = property on="Loading" class="Ring (strict)"(error in=w2337, "Visible"=TRUE) -> (error out=w2336:errorcluster)  [unwired: 1 in, 1 out]
        n1297 = control-ref of="LayerStitchTypes"() -> (w2321:refnum<vi>)
        n1298 = control-ref of="BackLayer"() -> (w2332:refnum<vi>)
        n1299 = control-ref of="FrontLayer"() -> (w2333:refnum<vi>)
        n1300 = control-ref of="ThreatGroups"() -> (w2334:refnum<vi>)
        n1301 = control-ref of="SampleClamping"() -> (w2342:refnum<vi>)
        n1302 = control-ref of="SampleTypes"() -> (w2359:refnum<vi>)
        n1303 = control-ref of="SampleDimensions"() -> (w2358:refnum<vi>)
        n1304 = control-ref of="ModelMfrs"() -> (w2357:refnum<vi>)
        n1305 = control-ref of="Assemblers"() -> (w2356:refnum<vi>)
        n1306 = control-ref of="Submitters"() -> (w2355:refnum<vi>)
        n1307 = control-ref of="PowderTypes"() -> (w2354:refnum<vi>)
        n1308 = control-ref of="Methods"() -> (w2351:refnum<vi>)
        n1309 = control-ref of="TestConditions"() -> (w2350:refnum<vi>)
        n1310 = control-ref of="SampleBackings"() -> (w2349:refnum<vi>)
        n1311 = control-ref of="Ballisticians"() -> (w2348:refnum<vi>)
        n1312 = control-ref of="Shooters"() -> (w2347:refnum<vi>)
        n1313 = control-ref of="Recorders"() -> (w2346:refnum<vi>)
        n1314 = Build Array(w2321, w2332, w2333, w2334, w2342, w2359, w2358, w2357, w2356, w2355, w2354, w2351, w2350, w2349, w2348, w2347, w2346) -> (w2353:refnum<vi>[])
        n1315 = call "Update Metadata using listbox names.vi"("error in"=w2336, "Site"="Site", "RefNumArrIn"=w2353) -> ("error out"=w2360:errorcluster, "RefNumArrOut"=w2352:refnum<vi>[])  [unwired: 1 in, 6 out]
        n1316 = call "Fill Lists from DB (1st Pass).vi"("error in"=w2360, "RefNumArray"=w2352) -> ("error out"=w2322:errorcluster)  [unwired: 1 in, 4 out]
        n1317 = call "Fill Stitch Lists.vi"("error IN"=w2322) -> ("error OUT"=w2317:errorcluster)  [unwired: 6 in]
        n1318 = control-ref of="ThreatSize_0"() -> (w2315:refnum<vi>)
        n1319 = control-ref of="Requestors_0"() -> (w2320:refnum<vi>)
        n1320 = Build Array(w2315, w2320) -> (w2319:refnum<vi>[])
        n1321 = call "Fill Lists from DB (2nd Pass).vi"("errorIN"=w2317, "colNames"=string[] ["GrainSize", "requestor"] ("lkupTableNames"), "lkupTableNames"=string[] ["ThreatDetails", "Submitters"], "RefNumArray"=w2319) -> ("error OUT"=w2316:errorcluster)  [unwired: 3 in]
        n1322 = flat-sequence {
          frame #0 {
            n1323 = local write "RefreshMetadata"(FALSE ("UpdateMetadata")) -> ()
            n1324 = local write "TimeNow"("Connecting to BIMS Server . . ." ("TimeNow")) -> ()
          }
        }
        n1325 = call "Create local tables from Server DB.vi"("error in"=w2316, "Site"="Site", "tableNames"=string[] ["Threats", "ThreatDetails", "ThreatCalibers", "Mfrs", "SampleStyles", "SampleSpecs", "FiberTypes"]) -> ("error out"=w2344:errorcluster)  [unwired: 1 in, 7 out]
        n1326 = call "Fill Lists From DB (3rd Pass).vi"("error IN"=w2344) -> ("error OUT"=w2324:errorcluster)  [unwired: 3 in, 3 out]
        n1327 = control-ref of="ModelMfrs"() -> (w2331:refnum<vi>)
        n1328 = property class="Ring (strict)"(reference=w2331, error in=w2324) -> (reference out=w2330:refnum<vi>, error out=w2329:errorcluster, "Strings []"=w2328:string[])
        n1329 = Delete From Array(array=w2328, length=1, index=0) -> (array with subset deleted=w2327:string[])  [unwired: 1 out]
        n1330 = property class="Ring (strict)"(reference=w2330, error in=w2329, "Strings []"=w2327) -> (error out=w2323:errorcluster)  [unwired: 1 out]
        n1331 = case shown="No Error" w2323 {
          selector: w2323 -> [w2361 w2364]
          tunnel: [w2361 w2364] -> w2340
          frame No Error {
            n1332 = local write "TimeNow"("Collector Metadata is READY!" ("TimeNow")) -> ()
            n1333 = Wait (ms)(milliseconds to wait=u32 2000) -> ()  [unwired: 1 out]
          }
          frame Error {
            n1334 = call <vilib>:"General Error Handler.vi"("error in (no error)"=w2364) -> ()  [unwired: 2 in, 13 out]
          }
        }
        n1335 = property on="Loading" class="Ring (strict)"(error in=w2340, "Visible"=FALSE) -> (error out=w2339:errorcluster)  [unwired: 1 in, 1 out]
      }
      event "loadingUnits": Value Change {
        n1336 = local read "Powder Loading"() -> (w2368:sgl)
        n1337 = event-data() -> ("NewVal"=w2367:enum32{"grams", "grains"})  [unwired: 6 out]
        n1338 = case shown="\"grams\", Default" w2367 {
          tunnel: w2368 -> [w2373 w2374]
          frame "grams", Default {
            n1339 = Multiply(x=w2373, y=sgl 0.06479891) -> (x*y=w2371:sgl)
            n1340 = local write "Powder Loading"(w2371) -> ()
          }
          frame "grains" {
            n1341 = Multiply(x=w2374, y=sgl 15.432359) -> (x*y=w2375:sgl)
            n1342 = local write "Powder Loading"(w2375) -> ()
          }
        }
      }
      event "clearErrors": Value Change {
        w2377 = errorcluster {"status"=FALSE, "code"=0, "source"=""} ("error in")
        n1343 = event-data() -> ()  [unwired: 7 out]
        n1344 = local write "SMErr"(w2377) -> ()
      }
    }
    "U/I EvErr" <- w1872
    "booleanDump" <- w1871
  }
